vi "Microscope.vi"() -> ()   [LabVIEW 2012]
uses:
  typedefs/Graph.ctl
  typedefs/HWsettings.ctl
  typedefs/Stage Parameters.ctl
  typedefs/ScanMode.ctl
  typedefs/Scan Parameters.ctl
  typedefs/PMTs.ctl
  classes/Microscope.lvclass
  classes/MCCPMT.lvclass
  typedefs/StageEvent.ctl
  typedefs/MicroscopeEvent.ctl
  variables/GlobalUI.vi
  sequences/full_restart_acquire_sequence.vi
panel:
  out "must be an integer":dbl=82.0
  in  "Tab Control":enum32{"Run", "Settings"}(tab)
  in  "Close":bool
  in  "Rot":bool
  in  "SpecWiz":bool
  in  "MG17Motor":refnum<k7>(container)
  in  "dV":dbl=0.5 min=0.0 step=0.25
  in  "Stokes":bool=TRUE
  in  "Pump":bool=TRUE
  out "XY Graph":T1={[0.0, 0.20101165771484375, 0.4090237617492676, 0.6170353889465332, 0.825047492980957, 1.0170583724975586, 1.2410712242126465, 1.432082176208496, 1.6400938034057617, 1.8321051597595215, 2.0721187591552734], [0.8903510861280485, 0.8953041634908552, 0.8929806592987812, 0.8912776295731716, 0.8909548875762202, 0.8924578410823198, 0.8944300209603651, 0.8951743521341458, 0.8952005525914619, 0.8928044016768294]}
  out "XY Graph 2":T1={[0.0, 0.20101165771484375, 0.4090237617492676, 0.6170353889465332, 0.825047492980957, 1.0170583724975586, 1.2410712242126465, 1.432082176208496, 1.6400938034057617, 1.8321051597595215, 2.0721187591552734], [0.0045469702743902015, 0.004504096798780445, 0.0043075933689024, 0.00459937118902435, 0.004633908155487764, 0.004538633765243861, 0.004433831935975568, 0.004408822408536544, 0.004301638719512153, 0.00419088224085362]}
  out "XY Graph 3":T1={[0.0, 0.20101165771484375, 0.4090237617492676, 0.6170353889465332, 0.825047492980957, 1.0170583724975586, 1.2410712242126465, 1.432082176208496, 1.6400938034057617, 1.8321051597595215, 2.0721187591552734], [3.0555949885670746, 3.0528808593750005, 3.052250857469512, 3.0531321455792657, 3.0502929687499982, 3.0587985899390246, 3.0497058403201254, 3.0519769435975626, 3.0576517244664645, 3.065386814024396]}
  out "intensity1":dbl=0.8928044016768294 format="%#.4f"
  out "intensity2":dbl=0.00419088224085362 format="%#.4f"
  out "intensity3":dbl=3.065386814024396 format="%#.4f"
  in  "Use Image Controls Min Max values for tiff":bool=TRUE
  in  "preset3":bool
  in  "zero3":bool
  out "PMT3":bool
  in  "PMT3":dbl(slide)=0.7 min=0.0 max=1.0 step=0.01 scale=0.0..1.0
  in  "Hi-Res Mode":bool
  in  "autoscale1":bool
  in  "Sample Description":string="AXN static 25d"
  in  "Stokes Power (mW)":string="200"
  in  "Pump Power (mW)":string="5"
  in  "max1":dbl=250.0 caption="max" step=250.0 format="%#.0f"
  in  "min1":dbl format="%#.0f"
  in  "NormalMode":bool
  in  "SpeedMode":bool
  in  "Target position mm":dbl=82.1047 step=0.025 format="%_6g"
  out "PMT2":bool
  out "PMT1":bool
  in  "MoveStageTarget":bool
  in  "grayscale":bool
  in  "jet":bool
  in  "preset2":bool
  in  "preset1":bool
  in  "PMT2":dbl(slide)=0.7 min=0.0 max=1.0 step=0.01 scale=0.0..1.0
  in  "PMT1":dbl(slide)=0.6 min=0.0 max=1.0 step=0.01 scale=0.0..1.0 scale format="%#_1g"
  in  "Save This":bool
  in  "Acquire":bool
  in  "Zoom":dbl=4.0
  out "CH1":dbl[][](graph)=[[93.19026295731707, 104.20636432926828, 92.89253048780488, 100.93130716463415, 83.36509146341463, 82.17416158536585, 89.31974085365853, 99.74037728658537, 93.78572789634147, 90.21293826219512, 85.44921875, 94.08346036585365, 87.23561356707317, 91.4038681402439, 89.02200838414635, 93.78572789634147, 83.66282393292683, 84.8537538109756, 85.44921875, 91.9993330792683, 73.5399199695122, 100.33584222560977, 86.93788109756098, 92.2970655487805, 94.38119283536585, 89.31974085365853, 90.21293826219512, 86.93788109756098, 86.0446836890244, 85.1514862804878, 100.03810975609757, 92.2970655487805, 91.9993330792683, 91.4038681402439, 90.21293826219512, 97.3585175304878, 86.93788109756098, 83.36509146341463, 89.02200838414635, 89.31974085365853, 88.72427591463415, 90.8084032012195, 95.57212271341463, 84.8537538109756, 90.21293826219512, 75.32631478658537, 84.25828887195121, 81.28096417682927, 105.39729420731707, 90.8084032012195], [98.2517149390244, 83.96055640243902, 93.78572789634147, 100.33584222560977, 95.86985518292683, 90.8084032012195, 89.91520579268293, 89.61747332317073, 88.42654344512195, 96.16758765243902, 95.57212271341463, 99.14491234756098, 89.31974085365853, 94.38119283536585, 99.14491234756098, 93.78572789634147, 88.42654344512195, 87.23561356707317, 81.87642911585365, 79.4945693597561, 86.64014862804879, 80.38776676829268, 90.21293826219512, 92.59479801829268, 90.21293826219512, 88.42654344512195, 88.72427591463415, 91.7016006097561, 88.12881097560977, 89.02200838414635, 86.93788109756098, 101.82450457317074, 97.0607850609756, 94.97665777439023, 85.1514862804878, 100.33584222560977, 89.61747332317073, 96.16758765243902, 92.2970655487805, 91.1061356707317, 98.54944740853658, 89.02200838414635, 86.64014862804879, 87.83107850609755, 88.12881097560977, 91.4038681402439, 89.91520579268293, 91.9993330792683, 86.64014862804879, 91.9993330792683], [97.0607850609756, 90.51067073170732, 89.31974085365853, 99.14491234756098, 90.8084032012195, 77.41044207317073, 88.72427591463415, 89.91520579268293, 84.25828887195121, 98.2517149390244, 80.38776676829268, 93.78572789634147, 90.51067073170732, 100.63357469512195, 94.67892530487805, 96.16758765243902, 92.59479801829268, 82.76962652439023, 89.02200838414635, 90.51067073170732, 84.55602134146342, 87.23561356707317, 92.2970655487805, 88.12881097560977, 83.06735899390245, 89.02200838414635, 85.1514862804878, 83.66282393292683, 86.93788109756098, 87.53334603658537, 94.38119283536585, 96.76305259146342, 80.38776676829268, 100.03810975609757, 96.46532012195121, 84.25828887195121, 85.44921875, 103.6108993902439, 92.59479801829268, 87.53334603658537, 89.02200838414635, 86.0446836890244, 98.2517149390244, 88.12881097560977, 95.86985518292683, 91.7016006097561, 87.53334603658537, 84.25828887195121, 80.68549923780488, 89.61747332317073], [90.21293826219512, 88.42654344512195, 96.46532012195121, 93.78572789634147, 90.21293826219512, 88.42654344512195, 91.9993330792683, 85.44921875, 87.53334603658537, 77.11270960365853, 90.21293826219512, 94.67892530487805, 83.96055640243902, 90.8084032012195, 86.0446836890244, 86.34241615853658, 89.91520579268293, 87.83107850609755, 102.12223704268293, 91.9993330792683, 89.31974085365853, 98.54944740853658, 104.20636432926828, 80.98323170731707, 85.44921875, 83.96055640243902, 88.42654344512195, 86.64014862804879, 87.53334603658537, 91.7016006097561, 88.72427591463415, 91.7016006097561, 84.25828887195121, 88.42654344512195, 85.1514862804878, 82.47189405487805, 88.72427591463415, 102.71770198170731, 98.54944740853658, 81.28096417682927, 98.54944740853658, 82.17416158536585, 91.9993330792683, 83.36509146341463, 97.3585175304878, 86.93788109756098, 102.71770198170731, 97.9539824695122, 89.61747332317073, 91.4038681402439], [87.23561356707317, 93.48799542682927, 87.23561356707317, 85.44921875, 93.48799542682927, 89.31974085365853, 89.61747332317073, 92.89253048780488, 95.86985518292683, 86.64014862804879, 79.1968368902439, 85.7469512195122, 82.47189405487805, 89.61747332317073, 78.8991044207317, 86.34241615853658, 84.25828887195121, 83.06735899390245, 92.59479801829268, 88.12881097560977, 92.89253048780488, 78.30363948170732, 94.08346036585365, 82.17416158536585, 87.23561356707317, 94.08346036585365, 80.0900342987805, 92.59479801829268, 87.83107850609755, 87.53334603658537, 77.70817454268293, 76.51724466463415, 86.64014862804879, 81.87642911585365, 86.0446836890244, 80.98323170731707, 96.46532012195121, 88.12881097560977, 97.9539824695122, 86.64014862804879, 93.19026295731707, 91.9993330792683, 86.64014862804879, 87.53334603658537, 91.4038681402439, 85.7469512195122, 88.72427591463415, 85.7469512195122, 86.34241615853658, 81.57869664634147], [105.39729420731707, 88.12881097560977, 89.31974085365853, 88.12881097560977, 98.54944740853658, 76.81497713414635, 96.46532012195121, 94.38119283536585, 84.55602134146342, 76.21951219512195, 97.9539824695122, 80.0900342987805, 89.91520579268293, 87.83107850609755, 84.55602134146342, 86.64014862804879, 87.83107850609755, 95.86985518292683, 93.78572789634147, 84.25828887195121, 98.54944740853658, 87.83107850609755, 87.83107850609755, 89.61747332317073, 84.25828887195121, 94.08346036585365, 83.06735899390245, 98.84717987804879, 83.66282393292683, 77.11270960365853, 91.1061356707317, 90.51067073170732, 83.96055640243902, 86.64014862804879, 90.8084032012195, 85.7469512195122, 76.21951219512195, 84.25828887195121, 87.53334603658537, 86.0446836890244, 89.91520579268293, 88.72427591463415, 83.66282393292683, 88.42654344512195, 94.38119283536585, 90.51067073170732, 95.27439024390245, 84.25828887195121, 87.23561356707317, 84.8537538109756], [91.9993330792683, 88.72427591463415, 79.7923018292683, 75.32631478658537, 90.21293826219512, 86.93788109756098, 90.51067073170732, 94.08346036585365, 94.08346036585365, 94.38119283536585, 91.1061356707317, 99.74037728658537, 85.44921875, 92.2970655487805, 87.83107850609755, 86.93788109756098, 86.93788109756098, 93.19026295731707, 83.66282393292683, 93.48799542682927, 86.0446836890244, 101.82450457317074, 87.83107850609755, 97.9539824695122, 87.23561356707317, 90.8084032012195, 87.23561356707317, 90.8084032012195, 84.8537538109756, 79.4945693597561, 81.28096417682927, 87.23561356707317, 86.34241615853658, 94.08346036585365, 88.12881097560977, 85.7469512195122, 85.7469512195122, 89.91520579268293, 89.61747332317073, 88.42654344512195, 87.53334603658537, 97.65625, 87.23561356707317, 92.59479801829268, 97.65625, 96.16758765243902, 91.4038681402439, 95.86985518292683, 89.61747332317073, 83.66282393292683], [88.42654344512195, 89.02200838414635, 95.57212271341463, 85.44921875, 91.7016006097561, 87.53334603658537, 81.87642911585365, 79.7923018292683, 96.46532012195121, 80.38776676829268, 92.89253048780488, 94.08346036585365, 95.86985518292683, 78.8991044207317, 93.48799542682927, 87.23561356707317, 89.61747332317073, 73.8376524390244, 77.11270960365853, 83.36509146341463, 83.36509146341463, 100.33584222560977, 87.23561356707317, 86.34241615853658, 104.50409679878048, 83.36509146341463, 91.9993330792683, 85.7469512195122, 100.03810975609757, 86.0446836890244, 89.61747332317073, 91.4038681402439, 97.0607850609756, 92.2970655487805, 88.12881097560977, 89.02200838414635, 90.8084032012195, 90.8084032012195, 83.66282393292683, 91.7016006097561, 81.28096417682927, 82.76962652439023, 94.08346036585365, 82.47189405487805, 91.1061356707317, 83.06735899390245, 93.78572789634147, 82.76962652439023, 89.61747332317073, 89.61747332317073], [89.02200838414635, 83.36509146341463, 93.78572789634147, 99.44264481707317, 91.7016006097561, 86.93788109756098, 87.23561356707317, 90.8084032012195, 90.21293826219512, 87.23561356707317, 90.51067073170732, 94.97665777439023, 87.83107850609755, 88.72427591463415, 88.12881097560977, 84.55602134146342, 84.55602134146342, 109.86328125, 75.32631478658537, 85.7469512195122, 80.38776676829268, 82.47189405487805, 93.78572789634147, 80.0900342987805, 91.4038681402439, 85.7469512195122, 87.83107850609755, 79.7923018292683, 95.57212271341463, 90.8084032012195, 89.91520579268293, 84.55602134146342, 88.42654344512195, 91.1061356707317, 87.53334603658537, 95.57212271341463, 95.27439024390245, 69.37166539634147, 94.08346036585365, 90.8084032012195, 82.47189405487805, 86.0446836890244, 98.84717987804879, 90.51067073170732, 97.65625, 84.25828887195121, 100.03810975609757, 79.4945693597561, 89.91520579268293, 94.67892530487805], [96.76305259146342, 84.8537538109756, 96.76305259146342, 85.1514862804878, 90.51067073170732, 88.12881097560977, 89.31974085365853, 84.8537538109756, 96.16758765243902, 78.00590701219512, 82.47189405487805, 92.59479801829268, 87.83107850609755, 84.25828887195121, 94.67892530487805, 86.64014862804879, 92.2970655487805, 78.00590701219512, 86.0446836890244, 91.9993330792683, 84.8537538109756, 86.64014862804879, 90.51067073170732, 81.28096417682927, 75.92177972560977, 86.64014862804879, 79.7923018292683, 71.75352515243902, 89.91520579268293, 83.36509146341463, 88.12881097560977, 82.17416158536585, 95.86985518292683, 90.21293826219512, 88.12881097560977, 88.42654344512195, 94.67892530487805, 91.9993330792683, 90.8084032012195, 84.8537538109756, 88.12881097560977, 93.19026295731707, 95.27439024390245, 94.08346036585365, 81.87642911585365, 94.67892530487805, 94.67892530487805, 96.76305259146342, 83.96055640243902, 82.47189405487805], [86.34241615853658, 91.7016006097561, 96.46532012195121, 88.12881097560977, 89.91520579268293, 103.9086318597561, 98.54944740853658, 96.76305259146342, 92.89253048780488, 98.84717987804879, 81.28096417682927, 94.38119283536585, 89.91520579268293, 90.21293826219512, 92.59479801829268, 88.72427591463415, 92.2970655487805, 90.21293826219512, 86.34241615853658, 91.9993330792683, 78.00590701219512, 84.55602134146342, 81.57869664634147, 97.3585175304878, 83.66282393292683, 88.72427591463415, 100.03810975609757, 83.66282393292683, 91.9993330792683, 104.80182926829269, 89.61747332317073, 90.21293826219512, 92.59479801829268, 88.72427591463415, 96.16758765243902, 89.02200838414635, 88.72427591463415, 88.72427591463415, 91.7016006097561, 87.83107850609755, 89.31974085365853, 87.53334603658537, 104.20636432926828, 86.34241615853658, 85.1514862804878, 96.16758765243902, 88.42654344512195, 78.8991044207317, 92.59479801829268, 94.97665777439023], [91.9993330792683, 86.0446836890244, 98.84717987804879, 89.61747332317073, 85.1514862804878, 85.1514862804878, 94.08346036585365, 88.12881097560977, 100.93130716463415, 84.55602134146342, 89.91520579268293, 86.64014862804879, 83.66282393292683, 93.48799542682927, 99.14491234756098, 86.93788109756098, 93.78572789634147, 95.86985518292683, 86.34241615853658, 104.20636432926828, 104.20636432926828, 93.48799542682927, 94.08346036585365, 86.34241615853658, 102.41996951219512, 93.78572789634147, 94.38119283536585, 79.4945693597561, 86.64014862804879, 88.42654344512195, 89.61747332317073, 86.0446836890244, 80.98323170731707, 86.64014862804879, 84.8537538109756, 90.21293826219512, 88.42654344512195, 91.9993330792683, 87.53334603658537, 98.2517149390244, 93.78572789634147, 87.23561356707317, 93.48799542682927, 81.57869664634147, 91.4038681402439, 98.2517149390244, 86.93788109756098, 92.89253048780488, 84.8537538109756, 99.44264481707317], [87.83107850609755, 91.1061356707317, 91.1061356707317, 90.8084032012195, 90.8084032012195, 76.81497713414635, 79.7923018292683, 95.57212271341463, 89.91520579268293, 93.78572789634147, 94.08346036585365, 93.78572789634147, 89.91520579268293, 88.12881097560977, 96.46532012195121, 95.86985518292683, 93.78572789634147, 88.72427591463415, 83.96055640243902, 89.91520579268293, 88.72427591463415, 86.34241615853658, 88.12881097560977, 87.83107850609755, 98.2517149390244, 90.21293826219512, 95.57212271341463, 89.31974085365853, 89.91520579268293, 82.76962652439023, 88.42654344512195, 86.34241615853658, 93.19026295731707, 95.57212271341463, 85.1514862804878, 89.91520579268293, 87.53334603658537, 101.82450457317074, 93.48799542682927, 86.0446836890244, 89.91520579268293, 85.1514862804878, 82.17416158536585, 93.78572789634147, 90.8084032012195, 94.08346036585365, 87.23561356707317, 100.33584222560977, 89.61747332317073, 80.98323170731707], [94.08346036585365, 94.08346036585365, 92.59479801829268, 91.9993330792683, 86.34241615853658, 87.83107850609755, 86.0446836890244, 79.7923018292683, 94.97665777439023, 88.72427591463415, 95.57212271341463, 81.57869664634147, 83.96055640243902, 93.48799542682927, 87.23561356707317, 94.08346036585365, 85.7469512195122, 88.72427591463415, 94.67892530487805, 100.63357469512195, 84.55602134146342, 95.27439024390245, 88.42654344512195, 102.41996951219512, 91.1061356707317, 93.78572789634147, 98.54944740853658, 100.03810975609757, 94.08346036585365, 90.8084032012195, 91.9993330792683, 92.2970655487805, 96.16758765243902, 89.61747332317073, 92.89253048780488, 91.7016006097561, 87.53334603658537, 91.1061356707317, 86.64014862804879, 79.4945693597561, 82.17416158536585, 93.48799542682927, 94.38119283536585, 91.7016006097561, 85.1514862804878, 92.89253048780488, 86.93788109756098, 99.44264481707317, 92.59479801829268, 87.53334603658537], [91.9993330792683, 87.53334603658537, 87.23561356707317, 91.1061356707317, 78.00590701219512, 83.96055640243902, 78.30363948170732, 99.14491234756098, 94.97665777439023, 86.93788109756098, 94.97665777439023, 91.7016006097561, 84.25828887195121, 90.8084032012195, 82.17416158536585, 98.54944740853658, 88.72427591463415, 91.1061356707317, 81.57869664634147, 85.44921875, 88.72427591463415, 83.06735899390245, 91.4038681402439, 98.2517149390244, 83.96055640243902, 89.31974085365853, 80.0900342987805, 106.88595655487805, 88.72427591463415, 81.87642911585365, 89.02200838414635, 92.2970655487805, 86.93788109756098, 89.61747332317073, 94.08346036585365, 81.87642911585365, 85.7469512195122, 91.4038681402439, 83.06735899390245, 86.64014862804879, 87.83107850609755, 86.0446836890244, 83.66282393292683, 94.67892530487805, 98.2517149390244, 86.93788109756098, 98.84717987804879, 80.38776676829268, 103.9086318597561, 94.38119283536585], [86.64014862804879, 82.76962652439023, 81.57869664634147, 96.16758765243902, 89.91520579268293, 78.8991044207317, 101.22903963414633, 88.42654344512195, 70.26486280487805, 81.28096417682927, 81.28096417682927, 92.89253048780488, 88.12881097560977, 88.72427591463415, 95.27439024390245, 87.83107850609755, 85.44921875, 93.78572789634147, 79.7923018292683, 83.36509146341463, 93.48799542682927, 95.86985518292683, 88.12881097560977, 87.23561356707317, 96.16758765243902, 83.06735899390245, 78.00590701219512, 86.0446836890244, 93.48799542682927, 78.30363948170732, 93.19026295731707, 99.44264481707317, 90.21293826219512, 90.51067073170732, 94.67892530487805, 80.68549923780488, 91.1061356707317, 92.89253048780488, 90.8084032012195, 88.42654344512195, 92.59479801829268, 94.67892530487805, 89.31974085365853, 73.2421875, 94.38119283536585, 94.38119283536585, 89.31974085365853, 93.19026295731707, 89.02200838414635, 88.12881097560977], [92.2970655487805, 92.59479801829268, 97.0607850609756, 98.2517149390244, 82.17416158536585, 95.57212271341463, 78.00590701219512, 88.12881097560977, 95.86985518292683, 89.02200838414635, 91.7016006097561, 83.06735899390245, 80.98323170731707, 90.51067073170732, 82.76962652439023, 99.44264481707317, 85.7469512195122, 89.31974085365853, 86.34241615853658, 97.9539824695122, 88.12881097560977, 91.9993330792683, 72.34899009146342, 95.27439024390245, 94.97665777439023, 91.4038681402439, 87.53334603658537, 81.57869664634147, 83.96055640243902, 91.4038681402439, 94.97665777439023, 83.66282393292683, 95.57212271341463, 84.8537538109756, 94.38119283536585, 91.9993330792683, 92.89253048780488, 81.87642911585365, 103.01543445121952, 95.27439024390245, 94.97665777439023, 85.7469512195122, 91.4038681402439, 94.08346036585365, 94.67892530487805, 81.57869664634147, 95.86985518292683, 96.76305259146342, 89.31974085365853, 87.23561356707317], [85.44921875, 87.83107850609755, 96.76305259146342, 97.0607850609756, 91.9993330792683, 99.14491234756098, 81.57869664634147, 84.55602134146342, 94.38119283536585, 88.72427591463415, 81.87642911585365, 80.0900342987805, 85.1514862804878, 93.19026295731707, 84.55602134146342, 95.86985518292683, 96.76305259146342, 85.7469512195122, 93.19026295731707, 89.31974085365853, 88.42654344512195, 94.97665777439023, 104.80182926829269, 86.34241615853658, 88.72427591463415, 88.72427591463415, 97.65625, 94.67892530487805, 86.93788109756098, 76.51724466463415, 85.7469512195122, 88.42654344512195, 91.9993330792683, 83.06735899390245, 79.4945693597561, 82.76962652439023, 88.72427591463415, 89.61747332317073, 109.86328125, 82.76962652439023, 97.0607850609756, 85.7469512195122, 83.66282393292683, 98.2517149390244, 93.19026295731707, 91.4038681402439, 90.51067073170732, 86.0446836890244, 86.93788109756098, 87.23561356707317], [97.0607850609756, 86.93788109756098, 75.62404725609755, 85.7469512195122, 89.91520579268293, 90.21293826219512, 80.38776676829268, 82.17416158536585, 75.92177972560977, 99.44264481707317, 88.72427591463415, 85.7469512195122, 94.67892530487805, 79.7923018292683, 86.93788109756098, 100.63357469512195, 92.89253048780488, 75.92177972560977, 89.02200838414635, 87.23561356707317, 95.86985518292683, 96.76305259146342, 75.62404725609755, 85.44921875, 83.36509146341463, 100.63357469512195, 96.46532012195121, 87.83107850609755, 93.19026295731707, 91.1061356707317, 88.12881097560977, 97.65625, 86.64014862804879, 94.67892530487805, 81.87642911585365, 89.91520579268293, 99.74037728658537, 96.46532012195121, 81.28096417682927, 87.23561356707317, 90.21293826219512, 92.2970655487805, 101.22903963414633, 97.9539824695122, 88.12881097560977, 88.12881097560977, 97.0607850609756, 86.34241615853658, 88.42654344512195, 101.52677210365854], [86.64014862804879, 92.2970655487805, 89.31974085365853, 84.55602134146342, 83.96055640243902, 95.86985518292683, 86.93788109756098, 86.34241615853658, 87.53334603658537, 83.06735899390245, 86.0446836890244, 97.0607850609756, 89.91520579268293, 94.97665777439023, 88.42654344512195, 99.44264481707317, 92.2970655487805, 88.12881097560977, 88.12881097560977, 84.8537538109756, 90.8084032012195, 85.7469512195122, 90.21293826219512, 95.57212271341463, 90.8084032012195, 90.51067073170732, 84.25828887195121, 87.53334603658537, 92.2970655487805, 79.7923018292683, 82.17416158536585, 91.7016006097561, 97.0607850609756, 88.72427591463415, 87.83107850609755, 87.23561356707317, 87.23561356707317, 80.68549923780488, 88.42654344512195, 93.19026295731707, 91.4038681402439, 78.6013719512195, 92.89253048780488, 93.19026295731707, 95.57212271341463, 82.17416158536585, 98.2517149390244, 89.91520579268293, 102.71770198170731, 89.31974085365853], [89.02200838414635, 89.02200838414635, 98.84717987804879, 86.0446836890244, 80.38776676829268, 89.02200838414635, 91.1061356707317, 94.67892530487805, 78.6013719512195, 87.53334603658537, 89.91520579268293, 89.31974085365853, 88.72427591463415, 93.48799542682927, 83.96055640243902, 92.59479801829268, 86.64014862804879, 86.64014862804879, 91.4038681402439, 95.86985518292683, 89.61747332317073, 87.53334603658537, 88.12881097560977, 85.7469512195122, 93.78572789634147, 94.67892530487805, 90.21293826219512, 91.1061356707317, 85.1514862804878, 89.02200838414635, 88.12881097560977, 84.8537538109756, 81.28096417682927, 92.59479801829268, 83.06735899390245, 85.1514862804878, 85.1514862804878, 90.51067073170732, 89.02200838414635, 81.87642911585365, 93.19026295731707, 93.19026295731707, 89.61747332317073, 81.87642911585365, 89.91520579268293, 91.1061356707317, 108.67235137195121, 89.31974085365853, 84.25828887195121, 79.4945693597561], [98.2517149390244, 95.57212271341463, 81.57869664634147, 87.53334603658537, 105.39729420731707, 97.0607850609756, 91.7016006097561, 91.4038681402439, 97.0607850609756, 90.8084032012195, 90.8084032012195, 86.64014862804879, 90.21293826219512, 90.8084032012195, 85.7469512195122, 84.25828887195121, 78.00590701219512, 82.76962652439023, 92.59479801829268, 95.57212271341463, 85.1514862804878, 86.64014862804879, 83.96055640243902, 89.02200838414635, 88.72427591463415, 91.9993330792683, 91.7016006097561, 95.57212271341463, 88.72427591463415, 94.97665777439023, 89.02200838414635, 94.08346036585365, 93.48799542682927, 98.84717987804879, 83.96055640243902, 81.28096417682927, 87.83107850609755, 84.25828887195121, 89.91520579268293, 88.12881097560977, 93.78572789634147, 89.91520579268293, 82.76962652439023, 82.76962652439023, 95.86985518292683, 79.7923018292683, 91.4038681402439, 81.57869664634147, 81.57869664634147, 83.06735899390245], [89.91520579268293, 86.34241615853658, 95.86985518292683, 82.76962652439023, 78.00590701219512, 89.31974085365853, 84.55602134146342, 97.3585175304878, 91.1061356707317, 88.72427591463415, 90.51067073170732, 94.08346036585365, 89.61747332317073, 82.47189405487805, 89.91520579268293, 83.66282393292683, 78.8991044207317, 88.72427591463415, 86.64014862804879, 91.4038681402439, 93.48799542682927, 86.0446836890244, 89.31974085365853, 102.12223704268293, 83.36509146341463, 90.51067073170732, 93.78572789634147, 96.16758765243902, 83.66282393292683, 81.87642911585365, 83.66282393292683, 83.36509146341463, 83.66282393292683, 94.38119283536585, 96.76305259146342, 85.7469512195122, 97.0607850609756, 87.53334603658537, 90.8084032012195, 87.53334603658537, 97.65625, 80.98323170731707, 89.61747332317073, 77.70817454268293, 81.87642911585365, 80.38776676829268, 87.83107850609755, 93.78572789634147, 90.8084032012195, 87.83107850609755], [82.17416158536585, 87.83107850609755, 87.23561356707317, 81.87642911585365, 83.96055640243902, 86.93788109756098, 98.54944740853658, 94.67892530487805, 83.36509146341463, 92.2970655487805, 90.8084032012195, 92.59479801829268, 90.21293826219512, 83.36509146341463, 85.44921875, 91.9993330792683, 81.57869664634147, 83.96055640243902, 94.67892530487805, 78.6013719512195, 97.0607850609756, 89.61747332317073, 85.44921875, 93.19026295731707, 88.12881097560977, 90.21293826219512, 86.93788109756098, 83.96055640243902, 91.9993330792683, 88.12881097560977, 92.59479801829268, 92.2970655487805, 93.48799542682927, 87.53334603658537, 84.25828887195121, 86.64014862804879, 81.28096417682927, 90.21293826219512, 91.7016006097561, 95.57212271341463, 88.12881097560977, 90.51067073170732, 72.9444550304878, 92.2970655487805, 82.17416158536585, 92.2970655487805, 76.21951219512195, 82.47189405487805, 88.72427591463415, 94.38119283536585], [95.57212271341463, 86.93788109756098, 84.8537538109756, 83.06735899390245, 82.17416158536585, 88.12881097560977, 94.08346036585365, 83.06735899390245, 87.53334603658537, 88.42654344512195, 83.36509146341463, 99.14491234756098, 80.38776676829268, 92.89253048780488, 89.02200838414635, 86.64014862804879, 86.93788109756098, 93.48799542682927, 87.23561356707317, 73.2421875, 81.28096417682927, 89.61747332317073, 91.9993330792683, 79.1968368902439, 85.7469512195122, 85.1514862804878, 83.36509146341463, 89.02200838414635, 91.4038681402439, 85.1514862804878, 92.59479801829268, 94.38119283536585, 94.38119283536585, 84.25828887195121, 81.28096417682927, 82.76962652439023, 79.1968368902439, 97.3585175304878, 96.46532012195121, 85.1514862804878, 97.3585175304878, 89.91520579268293, 99.44264481707317, 93.78572789634147, 93.78572789634147, 102.12223704268293, 92.59479801829268, 77.11270960365853, 83.96055640243902, 91.4038681402439], [93.19026295731707, 86.0446836890244, 83.96055640243902, 76.81497713414635, 90.51067073170732, 88.72427591463415, 88.42654344512195, 86.93788109756098, 87.23561356707317, 91.7016006097561, 98.84717987804879, 105.69502667682926, 96.46532012195121, 84.55602134146342, 99.74037728658537, 86.0446836890244, 82.47189405487805, 95.57212271341463, 90.8084032012195, 90.51067073170732, 80.0900342987805, 78.30363948170732, 88.72427591463415, 86.93788109756098, 97.3585175304878, 88.72427591463415, 91.9993330792683, 90.51067073170732, 83.36509146341463, 86.93788109756098, 91.7016006097561, 88.12881097560977, 103.31316692073172, 87.83107850609755, 95.86985518292683, 85.7469512195122, 98.84717987804879, 92.59479801829268, 93.48799542682927, 94.08346036585365, 94.97665777439023, 87.53334603658537, 84.55602134146342, 86.93788109756098, 97.3585175304878, 80.98323170731707, 82.76962652439023, 89.91520579268293, 87.83107850609755, 88.12881097560977], [103.9086318597561, 90.8084032012195, 88.72427591463415, 79.4945693597561, 83.66282393292683, 84.55602134146342, 80.38776676829268, 91.1061356707317, 93.48799542682927, 92.59479801829268, 96.76305259146342, 91.1061356707317, 94.67892530487805, 94.67892530487805, 89.02200838414635, 90.8084032012195, 88.42654344512195, 90.51067073170732, 89.61747332317073, 93.48799542682927, 85.7469512195122, 86.64014862804879, 84.8537538109756, 101.52677210365854, 92.2970655487805, 94.67892530487805, 89.91520579268293, 93.48799542682927, 87.53334603658537, 78.30363948170732, 89.31974085365853, 86.93788109756098, 78.30363948170732, 91.7016006097561, 84.8537538109756, 86.93788109756098, 100.33584222560977, 79.1968368902439, 87.83107850609755, 87.53334603658537, 89.02200838414635, 90.8084032012195, 101.52677210365854, 87.23561356707317, 87.53334603658537, 87.53334603658537, 101.22903963414633, 73.8376524390244, 87.53334603658537, 86.64014862804879], [93.19026295731707, 84.25828887195121, 69.37166539634147, 90.51067073170732, 84.25828887195121, 85.7469512195122, 91.7016006097561, 87.53334603658537, 91.1061356707317, 90.51067073170732, 77.70817454268293, 86.64014862804879, 89.61747332317073, 81.87642911585365, 78.6013719512195, 92.89253048780488, 84.25828887195121, 96.46532012195121, 89.91520579268293, 97.9539824695122, 99.44264481707317, 95.57212271341463, 84.8537538109756, 85.7469512195122, 83.66282393292683, 86.64014862804879, 80.0900342987805, 83.66282393292683, 84.25828887195121, 89.02200838414635, 86.93788109756098, 91.9993330792683, 88.12881097560977, 101.82450457317074, 101.82450457317074, 90.8084032012195, 84.8537538109756, 82.17416158536585, 83.36509146341463, 96.46532012195121, 109.86328125, 86.64014862804879, 84.8537538109756, 85.44921875, 77.41044207317073, 88.42654344512195, 87.83107850609755, 83.36509146341463, 84.8537538109756, 96.16758765243902], [98.54944740853658, 97.9539824695122, 96.46532012195121, 93.19026295731707, 89.31974085365853, 97.0607850609756, 95.57212271341463, 96.16758765243902, 80.38776676829268, 92.2970655487805, 92.59479801829268, 92.2970655487805, 89.02200838414635, 82.47189405487805, 89.31974085365853, 86.34241615853658, 77.41044207317073, 97.0607850609756, 86.64014862804879, 89.31974085365853, 84.55602134146342, 86.64014862804879, 82.47189405487805, 98.84717987804879, 83.66282393292683, 96.46532012195121, 89.61747332317073, 87.53334603658537, 98.84717987804879, 80.98323170731707, 94.08346036585365, 83.06735899390245, 88.12881097560977, 96.76305259146342, 91.1061356707317, 93.48799542682927, 89.02200838414635, 89.61747332317073, 91.4038681402439, 86.93788109756098, 86.34241615853658, 89.91520579268293, 91.4038681402439, 93.48799542682927, 80.68549923780488, 98.2517149390244, 91.1061356707317, 94.67892530487805, 95.57212271341463, 96.16758765243902], [80.68549923780488, 95.27439024390245, 80.68549923780488, 84.8537538109756, 86.0446836890244, 78.00590701219512, 78.8991044207317, 92.2970655487805, 84.8537538109756, 90.8084032012195, 78.8991044207317, 82.47189405487805, 87.23561356707317, 96.16758765243902, 89.31974085365853, 93.48799542682927, 83.66282393292683, 99.14491234756098, 90.51067073170732, 73.5399199695122, 91.4038681402439, 88.72427591463415, 87.53334603658537, 80.0900342987805, 96.16758765243902, 87.53334603658537, 86.64014862804879, 78.00590701219512, 88.12881097560977, 88.42654344512195, 81.87642911585365, 86.34241615853658, 97.3585175304878, 80.38776676829268, 100.03810975609757, 92.89253048780488, 92.59479801829268, 84.25828887195121, 87.83107850609755, 83.96055640243902, 74.73084984756098, 86.0446836890244, 99.14491234756098, 94.67892530487805, 79.1968368902439, 82.47189405487805, 84.25828887195121, 79.1968368902439, 89.31974085365853, 84.55602134146342], [84.55602134146342, 96.76305259146342, 79.1968368902439, 97.0607850609756, 94.97665777439023, 88.72427591463415, 93.78572789634147, 94.67892530487805, 89.61747332317073, 84.8537538109756, 89.02200838414635, 89.61747332317073, 89.02200838414635, 88.12881097560977, 90.8084032012195, 98.84717987804879, 80.0900342987805, 101.82450457317074, 94.97665777439023, 93.78572789634147, 84.25828887195121, 86.93788109756098, 89.31974085365853, 93.19026295731707, 97.65625, 91.1061356707317, 90.8084032012195, 92.89253048780488, 83.36509146341463, 89.31974085365853, 74.73084984756098, 90.21293826219512, 89.02200838414635, 85.1514862804878, 88.12881097560977, 92.59479801829268, 94.08346036585365, 94.08346036585365, 90.51067073170732, 90.8084032012195, 88.42654344512195, 93.48799542682927, 90.21293826219512, 85.7469512195122, 90.21293826219512, 85.7469512195122, 95.27439024390245, 95.86985518292683, 90.21293826219512, 92.89253048780488], [83.66282393292683, 88.42654344512195, 72.6467225609756, 86.0446836890244, 79.4945693597561, 91.1061356707317, 92.59479801829268, 89.61747332317073, 82.76962652439023, 101.22903963414633, 83.66282393292683, 80.98323170731707, 84.25828887195121, 83.36509146341463, 89.31974085365853, 87.53334603658537, 83.36509146341463, 83.66282393292683, 102.12223704268293, 89.31974085365853, 85.44921875, 90.51067073170732, 85.1514862804878, 90.21293826219512, 85.1514862804878, 92.2970655487805, 93.78572789634147, 93.48799542682927, 80.98323170731707, 91.1061356707317, 87.53334603658537, 81.57869664634147, 92.59479801829268, 102.12223704268293, 87.83107850609755, 96.16758765243902, 91.4038681402439, 87.53334603658537, 91.1061356707317, 88.12881097560977, 91.9993330792683, 86.34241615853658, 86.93788109756098, 84.8537538109756, 84.25828887195121, 97.3585175304878, 86.34241615853658, 84.55602134146342, 80.0900342987805, 82.76962652439023], [91.4038681402439, 88.42654344512195, 96.46532012195121, 90.51067073170732, 86.34241615853658, 87.23561356707317, 88.72427591463415, 87.83107850609755, 89.31974085365853, 101.52677210365854, 83.36509146341463, 75.32631478658537, 94.08346036585365, 94.97665777439023, 95.86985518292683, 90.21293826219512, 85.1514862804878, 94.97665777439023, 88.12881097560977, 90.21293826219512, 91.4038681402439, 96.16758765243902, 89.02200838414635, 94.97665777439023, 93.19026295731707, 86.34241615853658, 96.16758765243902, 91.1061356707317, 98.2517149390244, 81.28096417682927, 90.51067073170732, 82.47189405487805, 93.19026295731707, 88.72427591463415, 83.96055640243902, 85.7469512195122, 89.02200838414635, 89.61747332317073, 91.9993330792683, 82.76962652439023, 89.61747332317073, 89.91520579268293, 86.34241615853658, 96.76305259146342, 86.34241615853658, 83.66282393292683, 88.72427591463415, 92.2970655487805, 83.66282393292683, 98.84717987804879], [78.6013719512195, 86.34241615853658, 83.96055640243902, 76.21951219512195, 80.0900342987805, 90.51067073170732, 85.44921875, 92.2970655487805, 90.21293826219512, 93.19026295731707, 86.64014862804879, 96.16758765243902, 85.1514862804878, 84.25828887195121, 93.48799542682927, 89.61747332317073, 94.97665777439023, 89.02200838414635, 102.41996951219512, 93.78572789634147, 83.96055640243902, 85.44921875, 89.61747332317073, 81.87642911585365, 92.89253048780488, 84.55602134146342, 91.4038681402439, 88.42654344512195, 90.21293826219512, 91.7016006097561, 83.66282393292683, 81.87642911585365, 89.91520579268293, 86.93788109756098, 93.78572789634147, 103.01543445121952, 89.02200838414635, 99.14491234756098, 94.08346036585365, 89.61747332317073, 80.68549923780488, 101.22903963414633, 74.43311737804879, 90.21293826219512, 94.08346036585365, 90.51067073170732, 89.02200838414635, 96.16758765243902, 84.25828887195121, 86.93788109756098], [94.67892530487805, 87.23561356707317, 85.44921875, 94.97665777439023, 94.97665777439023, 89.61747332317073, 93.78572789634147, 93.19026295731707, 86.34241615853658, 89.02200838414635, 104.80182926829269, 80.0900342987805, 95.86985518292683, 89.31974085365853, 85.1514862804878, 88.72427591463415, 88.12881097560977, 86.0446836890244, 86.64014862804879, 90.51067073170732, 100.63357469512195, 87.53334603658537, 84.8537538109756, 75.92177972560977, 88.42654344512195, 89.61747332317073, 94.08346036585365, 96.16758765243902, 92.89253048780488, 76.51724466463415, 90.51067073170732, 91.9993330792683, 83.06735899390245, 76.21951219512195, 88.12881097560977, 83.36509146341463, 98.2517149390244, 99.44264481707317, 91.4038681402439, 80.0900342987805, 91.9993330792683, 80.98323170731707, 86.34241615853658, 87.83107850609755, 83.66282393292683, 89.31974085365853, 96.76305259146342, 83.96055640243902, 91.7016006097561, 100.63357469512195], [89.31974085365853, 93.48799542682927, 77.70817454268293, 91.1061356707317, 96.16758765243902, 87.53334603658537, 74.43311737804879, 89.02200838414635, 91.1061356707317, 77.41044207317073, 85.7469512195122, 92.59479801829268, 89.31974085365853, 98.54944740853658, 83.96055640243902, 90.8084032012195, 88.72427591463415, 85.44921875, 99.44264481707317, 86.64014862804879, 94.97665777439023, 91.1061356707317, 86.0446836890244, 83.36509146341463, 85.1514862804878, 87.23561356707317, 98.54944740853658, 84.25828887195121, 91.7016006097561, 80.38776676829268, 83.66282393292683, 97.0607850609756, 89.61747332317073, 85.44921875, 84.8537538109756, 86.34241615853658, 82.47189405487805, 95.27439024390245, 87.83107850609755, 86.93788109756098, 88.12881097560977, 94.97665777439023, 100.93130716463415, 84.55602134146342, 90.21293826219512, 83.96055640243902, 80.68549923780488, 83.66282393292683, 82.47189405487805, 84.8537538109756], [89.91520579268293, 83.36509146341463, 88.42654344512195, 93.78572789634147, 88.42654344512195, 86.64014862804879, 88.72427591463415, 81.57869664634147, 92.59479801829268, 95.57212271341463, 86.0446836890244, 94.08346036585365, 83.96055640243902, 84.55602134146342, 92.89253048780488, 97.3585175304878, 87.23561356707317, 92.59479801829268, 87.53334603658537, 86.0446836890244, 85.7469512195122, 93.78572789634147, 91.9993330792683, 88.72427591463415, 89.61747332317073, 96.46532012195121, 80.38776676829268, 97.3585175304878, 86.64014862804879, 88.12881097560977, 89.31974085365853, 87.23561356707317, 95.86985518292683, 88.42654344512195, 78.6013719512195, 97.9539824695122, 97.3585175304878, 81.57869664634147, 95.57212271341463, 84.25828887195121, 95.86985518292683, 85.1514862804878, 100.03810975609757, 91.9993330792683, 96.46532012195121, 88.42654344512195, 88.42654344512195, 83.06735899390245, 86.64014862804879, 84.8537538109756], [86.93788109756098, 97.65625, 101.22903963414633, 89.02200838414635, 76.81497713414635, 93.78572789634147, 89.02200838414635, 97.0607850609756, 86.0446836890244, 96.76305259146342, 92.89253048780488, 93.48799542682927, 78.00590701219512, 87.23561356707317, 83.06735899390245, 106.29049161585367, 85.44921875, 78.8991044207317, 90.8084032012195, 93.19026295731707, 87.83107850609755, 83.36509146341463, 88.12881097560977, 94.97665777439023, 85.1514862804878, 83.36509146341463, 91.1061356707317, 86.64014862804879, 93.48799542682927, 96.76305259146342, 80.98323170731707, 92.59479801829268, 84.55602134146342, 91.4038681402439, 94.08346036585365, 84.25828887195121, 100.63357469512195, 100.63357469512195, 88.72427591463415, 81.87642911585365, 88.12881097560977, 80.98323170731707, 98.84717987804879, 88.42654344512195, 92.2970655487805, 96.16758765243902, 90.21293826219512, 81.28096417682927, 93.19026295731707, 94.38119283536585], [72.9444550304878, 101.22903963414633, 90.8084032012195, 95.86985518292683, 92.89253048780488, 94.97665777439023, 85.1514862804878, 91.1061356707317, 92.59479801829268, 89.31974085365853, 81.87642911585365, 84.55602134146342, 83.06735899390245, 94.08346036585365, 72.05125762195121, 82.17416158536585, 91.9993330792683, 89.02200838414635, 94.38119283536585, 84.25828887195121, 87.23561356707317, 88.72427591463415, 75.32631478658537, 89.91520579268293, 91.7016006097561, 91.4038681402439, 90.8084032012195, 93.19026295731707, 98.84717987804879, 99.14491234756098, 86.0446836890244, 77.11270960365853, 94.67892530487805, 78.6013719512195, 91.9993330792683, 85.44921875, 94.67892530487805, 86.0446836890244, 93.78572789634147, 90.8084032012195, 89.91520579268293, 86.64014862804879, 97.65625, 78.8991044207317, 87.83107850609755, 85.7469512195122, 89.31974085365853, 84.25828887195121, 88.12881097560977, 95.86985518292683], [96.76305259146342, 84.55602134146342, 79.7923018292683, 97.65625, 97.65625, 95.27439024390245, 95.86985518292683, 93.19026295731707, 96.46532012195121, 92.89253048780488, 86.34241615853658, 83.36509146341463, 81.87642911585365, 79.1968368902439, 84.25828887195121, 95.86985518292683, 84.55602134146342, 96.76305259146342, 92.59479801829268, 96.16758765243902, 77.70817454268293, 86.34241615853658, 90.8084032012195, 81.87642911585365, 89.91520579268293, 97.0607850609756, 89.31974085365853, 89.91520579268293, 90.8084032012195, 88.42654344512195, 79.7923018292683, 84.25828887195121, 83.06735899390245, 80.98323170731707, 92.89253048780488, 83.66282393292683, 91.1061356707317, 85.1514862804878, 81.57869664634147, 77.11270960365853, 90.21293826219512, 80.68549923780488, 90.21293826219512, 94.38119283536585, 92.59479801829268, 92.2970655487805, 86.93788109756098, 82.76962652439023, 81.57869664634147, 76.81497713414635], [80.0900342987805, 92.59479801829268, 84.55602134146342, 96.46532012195121, 90.21293826219512, 73.5399199695122, 86.34241615853658, 83.36509146341463, 97.3585175304878, 95.57212271341463, 87.83107850609755, 95.27439024390245, 89.91520579268293, 93.19026295731707, 81.28096417682927, 93.48799542682927, 85.44921875, 84.8537538109756, 103.9086318597561, 93.48799542682927, 101.22903963414633, 83.66282393292683, 84.55602134146342, 97.9539824695122, 92.89253048780488, 86.0446836890244, 91.4038681402439, 91.7016006097561, 93.19026295731707, 86.34241615853658, 86.0446836890244, 83.96055640243902, 85.44921875, 80.0900342987805, 91.1061356707317, 89.61747332317073, 83.96055640243902, 89.02200838414635, 98.2517149390244, 99.44264481707317, 82.47189405487805, 90.21293826219512, 87.53334603658537, 87.23561356707317, 97.65625, 86.0446836890244, 80.38776676829268, 101.82450457317074, 95.57212271341463, 93.19026295731707], [83.36509146341463, 97.0607850609756, 88.72427591463415, 86.93788109756098, 89.91520579268293, 94.67892530487805, 89.91520579268293, 89.61747332317073, 87.83107850609755, 98.54944740853658, 77.70817454268293, 92.89253048780488, 91.1061356707317, 93.48799542682927, 100.03810975609757, 94.67892530487805, 85.1514862804878, 89.02200838414635, 92.89253048780488, 94.08346036585365, 90.8084032012195, 87.83107850609755, 89.91520579268293, 80.0900342987805, 89.91520579268293, 94.67892530487805, 85.7469512195122, 82.17416158536585, 94.08346036585365, 85.44921875, 103.6108993902439, 90.8084032012195, 98.54944740853658, 95.57212271341463, 86.0446836890244, 79.7923018292683, 88.12881097560977, 90.21293826219512, 76.51724466463415, 84.25828887195121, 82.17416158536585, 82.76962652439023, 88.12881097560977, 96.46532012195121, 78.8991044207317, 105.69502667682926, 81.87642911585365, 89.31974085365853, 80.98323170731707, 79.7923018292683], [91.1061356707317, 102.71770198170731, 85.7469512195122, 91.4038681402439, 91.4038681402439, 90.8084032012195, 95.27439024390245, 91.7016006097561, 71.75352515243902, 88.42654344512195, 92.89253048780488, 89.02200838414635, 80.38776676829268, 81.87642911585365, 84.8537538109756, 92.2970655487805, 86.0446836890244, 82.47189405487805, 96.16758765243902, 89.61747332317073, 80.98323170731707, 85.44921875, 86.0446836890244, 97.65625, 109.26781631097562, 98.84717987804879, 88.12881097560977, 82.76962652439023, 84.25828887195121, 91.4038681402439, 88.72427591463415, 78.6013719512195, 96.46532012195121, 89.61747332317073, 89.02200838414635, 84.55602134146342, 95.86985518292683, 90.51067073170732, 85.7469512195122, 94.38119283536585, 92.2970655487805, 88.72427591463415, 87.23561356707317, 88.42654344512195, 82.47189405487805, 88.42654344512195, 82.17416158536585, 85.7469512195122, 88.42654344512195, 99.14491234756098], [78.6013719512195, 103.31316692073172, 82.76962652439023, 82.17416158536585, 82.76962652439023, 83.96055640243902, 90.51067073170732, 85.7469512195122, 94.67892530487805, 89.31974085365853, 83.96055640243902, 84.55602134146342, 82.76962652439023, 103.9086318597561, 88.42654344512195, 95.27439024390245, 87.53334603658537, 82.47189405487805, 81.57869664634147, 90.8084032012195, 88.42654344512195, 95.27439024390245, 89.61747332317073, 81.87642911585365, 90.51067073170732, 95.27439024390245, 96.46532012195121, 88.42654344512195, 96.16758765243902, 80.0900342987805, 94.38119283536585, 90.21293826219512, 88.72427591463415, 93.78572789634147, 86.93788109756098, 82.47189405487805, 78.30363948170732, 81.57869664634147, 91.7016006097561, 86.34241615853658, 89.91520579268293, 84.25828887195121, 79.7923018292683, 92.59479801829268, 90.8084032012195, 98.54944740853658, 85.1514862804878, 85.1514862804878, 100.33584222560977, 101.22903963414633], [80.68549923780488, 83.06735899390245, 87.23561356707317, 95.27439024390245, 82.17416158536585, 94.38119283536585, 89.61747332317073, 105.09956173780488, 92.89253048780488, 84.55602134146342, 81.57869664634147, 82.17416158536585, 85.7469512195122, 100.63357469512195, 89.61747332317073, 102.12223704268293, 82.47189405487805, 91.1061356707317, 83.36509146341463, 91.4038681402439, 93.78572789634147, 94.08346036585365, 91.9993330792683, 86.64014862804879, 97.9539824695122, 92.59479801829268, 87.53334603658537, 85.44921875, 89.02200838414635, 90.8084032012195, 90.21293826219512, 83.36509146341463, 106.58822408536585, 94.67892530487805, 90.51067073170732, 88.42654344512195, 89.02200838414635, 77.70817454268293, 83.66282393292683, 103.9086318597561, 71.45579268292683, 93.19026295731707, 94.38119283536585, 90.8084032012195, 91.1061356707317, 85.7469512195122, 84.8537538109756, 87.53334603658537, 91.7016006097561, 83.96055640243902], [89.02200838414635, 81.57869664634147, 78.8991044207317, 85.44921875, 91.7016006097561, 79.1968368902439, 71.45579268292683, 82.17416158536585, 89.02200838414635, 89.91520579268293, 101.82450457317074, 93.48799542682927, 89.02200838414635, 86.34241615853658, 87.23561356707317, 83.96055640243902, 91.7016006097561, 101.82450457317074, 83.66282393292683, 89.31974085365853, 101.22903963414633, 76.81497713414635, 89.31974085365853, 80.68549923780488, 83.66282393292683, 87.83107850609755, 87.53334603658537, 82.17416158536585, 91.4038681402439, 94.08346036585365, 89.61747332317073, 85.1514862804878, 93.48799542682927, 92.59479801829268, 99.44264481707317, 101.22903963414633, 83.36509146341463, 86.93788109756098, 88.72427591463415, 83.06735899390245, 91.4038681402439, 95.86985518292683, 83.66282393292683, 89.61747332317073, 84.25828887195121, 87.83107850609755, 85.44921875, 100.93130716463415, 97.0607850609756, 89.61747332317073], [87.23561356707317, 78.30363948170732, 90.8084032012195, 89.61747332317073, 97.65625, 88.42654344512195, 89.61747332317073, 89.02200838414635, 86.34241615853658, 84.55602134146342, 89.31974085365853, 93.19026295731707, 88.42654344512195, 91.9993330792683, 89.61747332317073, 88.42654344512195, 90.51067073170732, 80.68549923780488, 84.25828887195121, 87.23561356707317, 92.59479801829268, 91.4038681402439, 96.46532012195121, 90.51067073170732, 86.0446836890244, 78.00590701219512, 87.53334603658537, 95.86985518292683, 83.06735899390245, 86.93788109756098, 97.3585175304878, 91.9993330792683, 86.0446836890244, 98.2517149390244, 88.42654344512195, 90.51067073170732, 94.08346036585365, 90.51067073170732, 79.1968368902439, 80.38776676829268, 86.93788109756098, 91.1061356707317, 91.4038681402439, 85.1514862804878, 94.08346036585365, 84.8537538109756, 88.42654344512195, 96.46532012195121, 92.89253048780488, 92.89253048780488], [87.23561356707317, 78.00590701219512, 77.41044207317073, 80.68549923780488, 79.1968368902439, 93.48799542682927, 89.31974085365853, 88.42654344512195, 87.53334603658537, 92.89253048780488, 83.36509146341463, 88.72427591463415, 83.36509146341463, 86.93788109756098, 84.25828887195121, 78.30363948170732, 86.0446836890244, 87.23561356707317, 83.06735899390245, 83.96055640243902, 89.61747332317073, 83.66282393292683, 84.8537538109756, 78.30363948170732, 97.65625, 90.51067073170732, 83.96055640243902, 89.02200838414635, 78.30363948170732, 82.47189405487805, 91.4038681402439, 86.34241615853658, 82.17416158536585, 82.47189405487805, 83.96055640243902, 96.16758765243902, 87.23561356707317, 78.6013719512195, 93.78572789634147, 82.17416158536585, 81.28096417682927, 87.83107850609755, 79.1968368902439, 84.8537538109756, 91.4038681402439, 93.48799542682927, 80.68549923780488, 82.76962652439023, 90.51067073170732, 84.55602134146342], [96.46532012195121, 91.9993330792683, 87.83107850609755, 96.16758765243902, 82.76962652439023, 89.31974085365853, 82.76962652439023, 97.3585175304878, 85.44921875, 93.19026295731707, 82.76962652439023, 93.78572789634147, 78.8991044207317, 87.23561356707317, 88.72427591463415, 89.91520579268293, 81.28096417682927, 88.42654344512195, 86.34241615853658, 97.9539824695122, 98.54944740853658, 89.61747332317073, 90.21293826219512, 86.34241615853658, 90.51067073170732, 94.38119283536585, 74.13538490853658, 93.78572789634147, 95.57212271341463, 86.93788109756098, 83.96055640243902, 92.59479801829268, 87.53334603658537, 82.76962652439023, 90.8084032012195, 82.76962652439023, 83.36509146341463, 91.4038681402439, 89.91520579268293, 90.51067073170732, 95.57212271341463, 86.34241615853658, 78.00590701219512, 76.81497713414635, 85.7469512195122, 99.14491234756098, 85.44921875, 83.66282393292683, 91.1061356707317, 94.38119283536585], [89.02200838414635, 85.7469512195122, 82.47189405487805, 100.33584222560977, 85.7469512195122, 91.9993330792683, 84.25828887195121, 99.14491234756098, 92.59479801829268, 83.36509146341463, 82.76962652439023, 92.89253048780488, 86.0446836890244, 82.76962652439023, 92.59479801829268, 87.23561356707317, 87.23561356707317, 92.89253048780488, 91.9993330792683, 89.31974085365853, 95.86985518292683, 77.11270960365853, 101.52677210365854, 95.27439024390245, 94.38119283536585, 88.42654344512195, 89.31974085365853, 88.72427591463415, 86.34241615853658, 100.03810975609757, 98.2517149390244, 90.8084032012195, 90.8084032012195, 78.30363948170732, 89.91520579268293, 90.8084032012195, 86.93788109756098, 82.17416158536585, 86.34241615853658, 80.0900342987805, 97.9539824695122, 95.86985518292683, 105.39729420731707, 89.61747332317073, 89.02200838414635, 92.59479801829268, 91.9993330792683, 94.08346036585365, 88.72427591463415, 94.67892530487805]]
  out "CH2":dbl[][](graph)=[[0.2977324695121951, 0.5954649390243902, 0.0, 0.0, 0.5954649390243902, 0.2977324695121951, 0.0, 0.2977324695121951, 0.5954649390243902, 0.8931974085365854, 0.0, 0.2977324695121951, 0.2977324695121951, 0.0, 0.0, 0.5954649390243902, 0.2977324695121951, 0.2977324695121951, 0.2977324695121951, 0.8931974085365854, 5.656916920731708, 0.0, 0.5954649390243902, 0.2977324695121951, 0.5954649390243902, 0.0, 0.2977324695121951, 0.0, 0.0, 0.5954649390243902, 0.2977324695121951, 1.1909298780487805, 0.0, 0.0, 0.5954649390243902, 2.0841272865853657, 0.2977324695121951, 0.5954649390243902, 0.5954649390243902, 0.0, 0.0, 0.0, 0.2977324695121951, 0.0, 0.0, 0.0, 0.0, 0.0, 0.5954649390243902, 0.2977324695121951], [0.2977324695121951, 0.0, 0.2977324695121951, 0.0, 0.0, 0.2977324695121951, 0.0, 0.0, 0.0, 1.7863948170731707, 0.0, 0.2977324695121951, 0.5954649390243902, 0.0, 0.2977324695121951, 4.763719512195122, 0.0, 0.8931974085365854, 0.0, 0.2977324695121951, 0.0, 0.0, 0.0, 0.2977324695121951, 0.0, 0.0, 0.5954649390243902, 0.0, 0.0, 0.0, 0.0, 0.0, 5.061451981707317, 0.2977324695121951, 0.0, 1.1909298780487805, 0.0, 0.2977324695121951, 0.2977324695121951, 1.7863948170731707, 0.0, 0.2977324695121951, 1.1909298780487805, 0.0, 0.0, 0.0, 0.0, 0.2977324695121951, 0.0, 0.0], [0.5954649390243902, 0.0, 0.2977324695121951, 0.0, 0.0, 0.0, 0.2977324695121951, 0.0, 0.5954649390243902, 0.0, 0.0, 0.0, 0.0, 0.2977324695121951, 0.0, 0.0, 0.0, 3.2750571646341466, 0.8931974085365854, 0.2977324695121951, 0.0, 0.0, 0.5954649390243902, 0.2977324695121951, 0.2977324695121951, 0.0, 0.5954649390243902, 0.0, 0.2977324695121951, 0.8931974085365854, 0.2977324695121951, 0.8931974085365854, 0.0, 1.7863948170731707, 0.0, 0.0, 0.2977324695121951, 0.5954649390243902, 2.0841272865853657, 0.0, 0.0, 0.0, 0.0, 0.5954649390243902, 0.5954649390243902, 0.0, 0.2977324695121951, 0.5954649390243902, 0.0, 0.2977324695121951], [0.0, 0.2977324695121951, 0.0, 0.0, 0.0, 2.679592225609756, 0.5954649390243902, 0.2977324695121951, 0.2977324695121951, 0.8931974085365854, 0.5954649390243902, 0.0, 0.2977324695121951, 0.0, 0.0, 0.2977324695121951, 0.0, 0.2977324695121951, 0.0, 0.0, 0.0, 0.0, 0.2977324695121951, 0.2977324695121951, 0.2977324695121951, 0.0, 0.0, 0.0, 0.5954649390243902, 0.0, 0.2977324695121951, 0.0, 0.0, 0.0, 0.2977324695121951, 0.2977324695121951, 0.0, 0.2977324695121951, 0.8931974085365854, 0.0, 0.0, 1.1909298780487805, 0.0, 0.2977324695121951, 0.2977324695121951, 0.0, 0.2977324695121951, 0.2977324695121951, 2.0841272865853657, 0.2977324695121951], [0.2977324695121951, 0.2977324695121951, 0.2977324695121951, 0.0, 0.0, 0.2977324695121951, 0.0, 0.0, 0.0, 0.0, 0.0, 0.0, 0.2977324695121951, 0.0, 0.0, 0.0, 0.0, 0.2977324695121951, 0.0, 0.0, 0.2977324695121951, 0.0, 0.0, 0.0, 0.0, 0.5954649390243902, 0.0, 0.0, 0.8931974085365854, 0.0, 0.2977324695121951, 0.0, 1.7863948170731707, 0.8931974085365854, 0.5954649390243902, 0.0, 0.2977324695121951, 0.2977324695121951, 0.2977324695121951, 0.0, 2.679592225609756, 0.0, 0.0, 4.1682545731707314, 1.1909298780487805, 1.4886623475609757, 0.0, 0.0, 0.0, 0.2977324695121951], [0.2977324695121951, 0.0, 0.0, 0.2977324695121951, 0.0, 0.0, 0.0, 0.0, 0.0, 0.0, 0.2977324695121951, 0.0, 0.2977324695121951, 0.2977324695121951, 0.2977324695121951, 0.0, 0.0, 0.2977324695121951, 0.2977324695121951, 0.0, 0.0, 0.0, 0.0, 0.2977324695121951, 2.0841272865853657, 0.0, 0.5954649390243902, 0.0, 0.5954649390243902, 2.9773246951219514, 0.2977324695121951, 0.2977324695121951, 0.0, 0.2977324695121951, 0.2977324695121951, 0.0, 0.0, 3.5727896341463414, 0.0, 0.0, 0.2977324695121951, 0.2977324695121951, 0.2977324695121951, 0.0, 0.2977324695121951, 0.0, 0.0, 0.0, 0.0, 0.0], [0.0, 0.0, 0.5954649390243902, 0.5954649390243902, 0.0, 0.2977324695121951, 0.0, 0.0, 0.0, 0.2977324695121951, 0.0, 0.8931974085365854, 0.2977324695121951, 0.5954649390243902, 0.0, 0.0, 0.2977324695121951, 0.2977324695121951, 1.4886623475609757, 0.2977324695121951, 0.0, 0.0, 0.0, 0.0, 0.0, 0.0, 0.2977324695121951, 0.0, 0.0, 0.0, 0.0, 0.2977324695121951, 0.0, 0.0, 0.0, 0.2977324695121951, 0.5954649390243902, 0.0, 0.5954649390243902, 0.0, 0.0, 0.0, 0.0, 0.0, 0.0, 1.4886623475609757, 0.0, 0.2977324695121951, 0.0, 0.2977324695121951], [0.2977324695121951, 0.2977324695121951, 0.0, 0.0, 0.0, 0.0, 0.0, 0.2977324695121951, 0.2977324695121951, 2.9773246951219514, 0.0, 0.0, 2.0841272865853657, 0.0, 0.0, 0.0, 0.0, 0.0, 0.5954649390243902, 0.2977324695121951, 2.381859756097561, 2.9773246951219514, 0.2977324695121951, 0.0, 0.0, 0.0, 0.0, 0.8931974085365854, 0.0, 0.8931974085365854, 0.0, 0.0, 0.2977324695121951, 0.5954649390243902, 0.0, 0.0, 0.0, 0.0, 0.0, 0.0, 0.5954649390243902, 0.5954649390243902, 0.2977324695121951, 1.4886623475609757, 0.2977324695121951, 0.0, 0.0, 0.2977324695121951, 0.2977324695121951, 0.0], [0.0, 0.0, 0.2977324695121951, 0.2977324695121951, 5.359184451219512, 0.0, 0.5954649390243902, 0.0, 0.2977324695121951, 2.381859756097561, 0.2977324695121951, 0.0, 0.2977324695121951, 0.5954649390243902, 0.2977324695121951, 1.1909298780487805, 0.0, 0.5954649390243902, 0.2977324695121951, 0.5954649390243902, 0.0, 0.0, 0.2977324695121951, 1.1909298780487805, 0.2977324695121951, 0.2977324695121951, 0.0, 0.0, 0.0, 0.5954649390243902, 0.8931974085365854, 0.0, 0.2977324695121951, 0.5954649390243902, 0.0, 0.0, 0.8931974085365854, 0.2977324695121951, 0.0, 0.8931974085365854, 0.5954649390243902, 0.2977324695121951, 0.0, 0.2977324695121951, 0.0, 0.2977324695121951, 0.2977324695121951, 0.0, 0.8931974085365854, 0.2977324695121951], [0.5954649390243902, 0.0, 0.0, 0.0, 0.0, 0.0, 0.0, 0.2977324695121951, 0.0, 0.2977324695121951, 0.2977324695121951, 0.0, 0.2977324695121951, 0.5954649390243902, 0.2977324695121951, 0.0, 0.2977324695121951, 0.0, 0.8931974085365854, 0.0, 0.5954649390243902, 0.0, 0.8931974085365854, 0.5954649390243902, 0.2977324695121951, 0.0, 0.0, 0.2977324695121951, 0.8931974085365854, 0.0, 5.359184451219512, 0.0, 0.8931974085365854, 0.0, 0.2977324695121951, 0.2977324695121951, 0.2977324695121951, 2.0841272865853657, 1.1909298780487805, 0.0, 0.0, 0.0, 0.2977324695121951, 0.8931974085365854, 0.2977324695121951, 0.0, 0.2977324695121951, 0.2977324695121951, 1.7863948170731707, 0.0], [0.0, 0.0, 0.0, 0.2977324695121951, 0.0, 0.0, 0.2977324695121951, 0.0, 0.0, 0.0, 0.5954649390243902, 0.5954649390243902, 2.9773246951219514, 0.8931974085365854, 1.7863948170731707, 0.5954649390243902, 0.2977324695121951, 0.0, 0.5954649390243902, 0.2977324695121951, 0.5954649390243902, 0.0, 0.0, 0.0, 0.5954649390243902, 0.0, 0.5954649390243902, 0.5954649390243902, 0.0, 0.5954649390243902, 0.2977324695121951, 0.5954649390243902, 0.5954649390243902, 0.2977324695121951, 0.2977324695121951, 0.5954649390243902, 0.2977324695121951, 0.0, 0.0, 0.0, 0.2977324695121951, 0.0, 0.0, 1.4886623475609757, 0.2977324695121951, 0.2977324695121951, 0.0, 0.5954649390243902, 0.5954649390243902, 0.0], [0.2977324695121951, 0.0, 0.2977324695121951, 0.5954649390243902, 0.2977324695121951, 0.2977324695121951, 0.5954649390243902, 0.0, 0.5954649390243902, 0.0, 0.2977324695121951, 2.679592225609756, 0.0, 0.0, 0.8931974085365854, 0.5954649390243902, 0.2977324695121951, 0.0, 0.0, 0.0, 0.2977324695121951, 5.656916920731708, 0.0, 0.8931974085365854, 0.0, 0.5954649390243902, 0.0, 0.2977324695121951, 1.1909298780487805, 0.0, 0.0, 0.0, 0.0, 0.0, 0.2977324695121951, 0.2977324695121951, 0.0, 0.0, 0.0, 0.2977324695121951, 1.4886623475609757, 0.2977324695121951, 0.2977324695121951, 0.2977324695121951, 0.0, 0.2977324695121951, 0.0, 0.0, 0.0, 0.8931974085365854], [0.0, 0.8931974085365854, 0.0, 0.2977324695121951, 0.0, 0.2977324695121951, 0.2977324695121951, 0.0, 0.5954649390243902, 0.0, 0.2977324695121951, 0.0, 0.0, 0.0, 1.4886623475609757, 0.2977324695121951, 0.5954649390243902, 0.0, 0.0, 0.0, 0.0, 1.1909298780487805, 0.0, 0.2977324695121951, 0.0, 0.0, 0.2977324695121951, 1.1909298780487805, 0.0, 0.2977324695121951, 0.5954649390243902, 0.2977324695121951, 0.0, 0.0, 0.2977324695121951, 0.0, 0.5954649390243902, 0.0, 0.2977324695121951, 0.0, 0.0, 0.0, 0.0, 0.5954649390243902, 0.2977324695121951, 0.2977324695121951, 0.0, 0.2977324695121951, 0.2977324695121951, 0.0], [0.2977324695121951, 0.0, 0.0, 0.0, 0.2977324695121951, 0.0, 0.2977324695121951, 1.1909298780487805, 0.2977324695121951, 0.0, 0.0, 0.2977324695121951, 0.0, 0.5954649390243902, 0.0, 0.0, 0.0, 0.0, 0.0, 0.0, 0.5954649390243902, 0.0, 0.2977324695121951, 0.5954649390243902, 0.0, 0.0, 0.2977324695121951, 0.0, 0.2977324695121951, 0.2977324695121951, 1.4886623475609757, 0.2977324695121951, 0.2977324695121951, 0.2977324695121951, 0.2977324695121951, 0.2977324695121951, 0.5954649390243902, 0.0, 0.0, 0.5954649390243902, 0.0, 0.0, 0.0, 0.2977324695121951, 0.0, 0.2977324695121951, 0.0, 0.2977324695121951, 0.2977324695121951, 0.2977324695121951], [0.2977324695121951, 0.2977324695121951, 0.5954649390243902, 0.0, 0.0, 2.679592225609756, 0.0, 0.8931974085365854, 0.2977324695121951, 0.0, 1.1909298780487805, 0.0, 0.5954649390243902, 0.5954649390243902, 0.0, 0.2977324695121951, 0.2977324695121951, 1.4886623475609757, 0.0, 1.1909298780487805, 0.5954649390243902, 0.0, 0.2977324695121951, 1.4886623475609757, 0.2977324695121951, 0.0, 1.1909298780487805, 0.5954649390243902, 0.2977324695121951, 0.0, 0.2977324695121951, 0.0, 0.0, 0.2977324695121951, 0.2977324695121951, 0.2977324695121951, 0.2977324695121951, 0.2977324695121951, 0.0, 0.2977324695121951, 0.5954649390243902, 2.679592225609756, 0.2977324695121951, 0.2977324695121951, 0.2977324695121951, 0.2977324695121951, 0.5954649390243902, 0.0, 0.2977324695121951, 1.1909298780487805], [0.0, 0.2977324695121951, 0.0, 0.0, 2.381859756097561, 0.8931974085365854, 0.0, 1.7863948170731707, 0.0, 0.0, 0.0, 0.0, 0.0, 0.5954649390243902, 0.2977324695121951, 0.0, 0.5954649390243902, 0.0, 0.0, 0.0, 0.8931974085365854, 9.527439024390244, 0.0, 0.2977324695121951, 0.2977324695121951, 0.2977324695121951, 0.0, 0.0, 0.2977324695121951, 0.2977324695121951, 0.0, 0.0, 0.0, 1.4886623475609757, 0.8931974085365854, 1.1909298780487805, 0.5954649390243902, 0.0, 0.2977324695121951, 0.0, 0.0, 0.2977324695121951, 0.2977324695121951, 0.2977324695121951, 0.0, 1.7863948170731707, 0.2977324695121951, 0.5954649390243902, 0.0, 0.0], [0.0, 0.2977324695121951, 0.0, 0.0, 0.0, 0.0, 0.2977324695121951, 0.0, 0.2977324695121951, 0.0, 0.5954649390243902, 0.0, 0.0, 0.2977324695121951, 0.8931974085365854, 1.1909298780487805, 0.2977324695121951, 0.2977324695121951, 0.0, 0.2977324695121951, 0.2977324695121951, 1.4886623475609757, 0.2977324695121951, 0.2977324695121951, 0.2977324695121951, 0.0, 0.2977324695121951, 0.0, 0.8931974085365854, 0.8931974085365854, 0.0, 0.0, 0.0, 0.2977324695121951, 0.5954649390243902, 0.8931974085365854, 0.8931974085365854, 0.0, 0.0, 0.0, 0.0, 0.0, 0.2977324695121951, 0.2977324695121951, 0.2977324695121951, 0.0, 0.2977324695121951, 0.0, 0.0, 0.0], [3.2750571646341466, 0.5954649390243902, 0.2977324695121951, 0.0, 0.2977324695121951, 0.2977324695121951, 2.9773246951219514, 0.0, 0.0, 0.2977324695121951, 0.0, 0.0, 0.0, 0.0, 0.0, 0.2977324695121951, 0.0, 0.2977324695121951, 2.381859756097561, 4.465987042682927, 0.8931974085365854, 0.2977324695121951, 0.2977324695121951, 0.2977324695121951, 2.381859756097561, 0.2977324695121951, 0.0, 0.0, 0.0, 0.2977324695121951, 1.4886623475609757, 0.0, 0.0, 0.0, 0.0, 0.0, 0.0, 0.2977324695121951, 0.0, 0.5954649390243902, 0.2977324695121951, 2.381859756097561, 0.0, 0.0, 0.0, 0.0, 0.0, 0.0, 0.0, 0.2977324695121951], [0.2977324695121951, 0.0, 0.0, 0.0, 0.2977324695121951, 0.2977324695121951, 0.5954649390243902, 0.5954649390243902, 0.2977324695121951, 3.2750571646341466, 0.2977324695121951, 0.8931974085365854, 0.8931974085365854, 0.0, 0.0, 0.0, 0.2977324695121951, 0.5954649390243902, 0.5954649390243902, 0.0, 2.679592225609756, 0.0, 0.0, 0.2977324695121951, 0.2977324695121951, 0.0, 0.0, 0.2977324695121951, 0.5954649390243902, 0.5954649390243902, 0.2977324695121951, 0.2977324695121951, 0.0, 3.5727896341463414, 0.8931974085365854, 0.0, 0.2977324695121951, 0.2977324695121951, 0.0, 0.2977324695121951, 0.0, 1.1909298780487805, 0.2977324695121951, 0.2977324695121951, 0.0, 0.5954649390243902, 0.5954649390243902, 0.0, 0.2977324695121951, 0.5954649390243902], [0.0, 0.0, 0.2977324695121951, 0.0, 0.0, 0.2977324695121951, 0.0, 0.5954649390243902, 0.0, 0.2977324695121951, 0.0, 0.0, 0.0, 0.0, 1.4886623475609757, 2.0841272865853657, 0.2977324695121951, 9.527439024390244, 0.0, 0.8931974085365854, 0.0, 0.0, 0.0, 0.2977324695121951, 0.2977324695121951, 0.2977324695121951, 0.8931974085365854, 0.2977324695121951, 0.2977324695121951, 0.0, 0.2977324695121951, 0.8931974085365854, 0.0, 0.0, 0.2977324695121951, 0.8931974085365854, 0.0, 0.8931974085365854, 0.0, 0.0, 0.0, 0.0, 0.0, 0.0, 0.0, 0.2977324695121951, 0.2977324695121951, 0.0, 0.2977324695121951, 0.0], [0.0, 0.2977324695121951, 0.0, 0.2977324695121951, 0.2977324695121951, 0.0, 0.2977324695121951, 0.0, 0.0, 0.2977324695121951, 0.2977324695121951, 0.8931974085365854, 0.2977324695121951, 0.8931974085365854, 0.2977324695121951, 0.0, 0.2977324695121951, 0.2977324695121951, 0.5954649390243902, 1.7863948170731707, 0.2977324695121951, 0.2977324695121951, 0.2977324695121951, 0.2977324695121951, 0.0, 0.0, 0.2977324695121951, 0.2977324695121951, 0.8931974085365854, 0.0, 0.2977324695121951, 0.2977324695121951, 0.0, 0.2977324695121951, 0.0, 1.1909298780487805, 1.1909298780487805, 0.2977324695121951, 0.0, 0.2977324695121951, 0.0, 0.2977324695121951, 1.1909298780487805, 0.2977324695121951, 0.8931974085365854, 0.2977324695121951, 0.0, 0.0, 0.0, 0.0], [2.679592225609756, 0.8931974085365854, 0.2977324695121951, 0.0, 0.0, 0.0, 0.0, 1.1909298780487805, 2.9773246951219514, 0.2977324695121951, 2.381859756097561, 0.0, 0.2977324695121951, 0.2977324695121951, 1.7863948170731707, 0.8931974085365854, 0.0, 0.0, 0.0, 0.5954649390243902, 0.2977324695121951, 0.2977324695121951, 0.0, 0.0, 0.2977324695121951, 0.0, 0.0, 0.0, 0.0, 0.0, 0.5954649390243902, 0.0, 0.0, 0.0, 0.0, 2.679592225609756, 0.2977324695121951, 0.0, 0.0, 0.0, 0.2977324695121951, 0.2977324695121951, 0.2977324695121951, 0.0, 0.0, 0.0, 0.2977324695121951, 0.2977324695121951, 0.8931974085365854, 0.0], [0.0, 0.2977324695121951, 0.0, 0.8931974085365854, 0.2977324695121951, 0.0, 0.2977324695121951, 0.0, 0.0, 0.2977324695121951, 1.4886623475609757, 1.4886623475609757, 0.2977324695121951, 0.0, 0.0, 1.1909298780487805, 0.5954649390243902, 0.5954649390243902, 0.2977324695121951, 0.0, 0.0, 0.0, 0.2977324695121951, 0.8931974085365854, 0.2977324695121951, 0.0, 0.0, 0.0, 0.0, 0.0, 0.2977324695121951, 0.0, 0.2977324695121951, 5.061451981707317, 0.2977324695121951, 0.2977324695121951, 0.2977324695121951, 0.0, 0.0, 0.0, 0.0, 0.0, 0.8931974085365854, 0.2977324695121951, 0.2977324695121951, 0.2977324695121951, 0.8931974085365854, 0.0, 0.5954649390243902, 0.0], [0.0, 0.2977324695121951, 0.2977324695121951, 0.2977324695121951, 0.0, 0.2977324695121951, 0.5954649390243902, 0.0, 0.5954649390243902, 2.0841272865853657, 0.0, 0.0, 0.5954649390243902, 0.0, 0.8931974085365854, 0.0, 1.7863948170731707, 0.8931974085365854, 0.2977324695121951, 0.0, 0.5954649390243902, 0.2977324695121951, 2.381859756097561, 0.2977324695121951, 0.2977324695121951, 0.2977324695121951, 0.0, 2.9773246951219514, 0.2977324695121951, 0.0, 0.0, 0.0, 0.2977324695121951, 0.2977324695121951, 0.0, 0.2977324695121951, 0.0, 0.0, 0.0, 0.0, 0.8931974085365854, 0.2977324695121951, 0.2977324695121951, 0.2977324695121951, 0.2977324695121951, 3.5727896341463414, 0.5954649390243902, 0.0, 0.2977324695121951, 1.7863948170731707], [0.0, 0.0, 0.0, 0.0, 0.0, 0.0, 0.5954649390243902, 0.8931974085365854, 0.0, 2.679592225609756, 0.2977324695121951, 0.0, 0.0, 0.5954649390243902, 2.0841272865853657, 0.0, 0.2977324695121951, 1.1909298780487805, 0.0, 0.2977324695121951, 0.0, 0.2977324695121951, 0.0, 0.2977324695121951, 0.2977324695121951, 0.0, 0.2977324695121951, 0.0, 1.1909298780487805, 0.0, 0.5954649390243902, 0.0, 1.1909298780487805, 1.4886623475609757, 0.0, 1.7863948170731707, 0.0, 0.2977324695121951, 0.5954649390243902, 0.2977324695121951, 0.2977324695121951, 0.2977324695121951, 0.0, 2.679592225609756, 3.5727896341463414, 0.2977324695121951, 0.5954649390243902, 2.679592225609756, 0.0, 0.2977324695121951], [0.2977324695121951, 0.2977324695121951, 0.5954649390243902, 0.0, 0.0, 0.0, 0.5954649390243902, 0.0, 0.2977324695121951, 0.0, 0.5954649390243902, 0.0, 0.0, 0.0, 0.5954649390243902, 0.2977324695121951, 0.0, 0.8931974085365854, 0.0, 0.0, 0.0, 0.0, 0.2977324695121951, 1.7863948170731707, 0.0, 0.2977324695121951, 0.0, 0.5954649390243902, 0.2977324695121951, 0.2977324695121951, 0.0, 0.0, 0.0, 0.0, 1.4886623475609757, 2.0841272865853657, 0.5954649390243902, 0.2977324695121951, 0.2977324695121951, 0.0, 0.2977324695121951, 0.0, 0.0, 0.2977324695121951, 0.0, 0.0, 0.0, 1.4886623475609757, 2.679592225609756, 0.0], [0.2977324695121951, 0.2977324695121951, 0.0, 4.1682545731707314, 0.0, 0.0, 0.5954649390243902, 0.2977324695121951, 0.0, 1.4886623475609757, 0.2977324695121951, 0.5954649390243902, 0.2977324695121951, 0.5954649390243902, 0.2977324695121951, 0.2977324695121951, 0.0, 0.8931974085365854, 0.8931974085365854, 0.0, 0.2977324695121951, 0.2977324695121951, 0.0, 0.0, 0.2977324695121951, 0.8931974085365854, 0.2977324695121951, 0.2977324695121951, 0.0, 0.0, 0.2977324695121951, 0.0, 0.0, 0.0, 0.0, 0.8931974085365854, 0.0, 1.4886623475609757, 3.5727896341463414, 0.0, 0.0, 0.0, 0.0, 0.0, 0.0, 0.2977324695121951, 0.0, 0.0, 1.7863948170731707, 0.0], [0.5954649390243902, 0.2977324695121951, 0.2977324695121951, 0.5954649390243902, 0.0, 0.2977324695121951, 0.5954649390243902, 1.7863948170731707, 0.2977324695121951, 0.0, 0.2977324695121951, 0.0, 1.1909298780487805, 0.0, 0.5954649390243902, 0.0, 0.2977324695121951, 0.2977324695121951, 0.2977324695121951, 0.2977324695121951, 0.2977324695121951, 0.0, 2.679592225609756, 0.0, 1.1909298780487805, 0.2977324695121951, 1.7863948170731707, 0.0, 0.0, 0.2977324695121951, 0.0, 0.2977324695121951, 0.2977324695121951, 0.2977324695121951, 0.8931974085365854, 0.5954649390243902, 0.2977324695121951, 0.5954649390243902, 1.1909298780487805, 0.0, 0.0, 0.0, 0.0, 1.1909298780487805, 0.0, 1.4886623475609757, 2.679592225609756, 0.2977324695121951, 1.4886623475609757, 0.2977324695121951], [0.2977324695121951, 0.0, 0.2977324695121951, 0.2977324695121951, 0.0, 1.4886623475609757, 0.2977324695121951, 0.0, 0.0, 0.2977324695121951, 0.0, 2.381859756097561, 0.2977324695121951, 0.0, 2.381859756097561, 0.0, 0.2977324695121951, 0.0, 0.0, 0.2977324695121951, 2.0841272865853657, 0.5954649390243902, 0.5954649390243902, 1.4886623475609757, 0.0, 0.2977324695121951, 0.0, 0.0, 0.0, 0.0, 0.0, 0.2977324695121951, 0.8931974085365854, 0.0, 0.0, 0.2977324695121951, 0.2977324695121951, 0.0, 5.359184451219512, 0.2977324695121951, 1.7863948170731707, 1.1909298780487805, 0.2977324695121951, 1.4886623475609757, 0.2977324695121951, 0.0, 0.0, 0.0, 0.2977324695121951, 0.0], [0.0, 0.2977324695121951, 0.0, 0.0, 1.7863948170731707, 0.0, 0.5954649390243902, 0.2977324695121951, 0.5954649390243902, 0.0, 5.061451981707317, 0.8931974085365854, 0.0, 0.0, 0.0, 0.2977324695121951, 0.0, 0.2977324695121951, 0.5954649390243902, 0.0, 0.2977324695121951, 0.2977324695121951, 0.0, 0.2977324695121951, 0.2977324695121951, 0.2977324695121951, 0.0, 0.2977324695121951, 0.0, 0.0, 0.0, 0.0, 0.0, 0.0, 0.2977324695121951, 0.5954649390243902, 0.0, 2.679592225609756, 0.5954649390243902, 0.0, 0.2977324695121951, 0.5954649390243902, 0.2977324695121951, 0.5954649390243902, 0.0, 0.0, 0.0, 0.2977324695121951, 0.5954649390243902, 2.381859756097561], [0.2977324695121951, 0.5954649390243902, 0.0, 0.2977324695121951, 0.2977324695121951, 2.381859756097561, 0.2977324695121951, 0.2977324695121951, 1.1909298780487805, 0.2977324695121951, 0.2977324695121951, 2.9773246951219514, 0.5954649390243902, 0.2977324695121951, 0.2977324695121951, 0.0, 0.5954649390243902, 3.8705221036585367, 0.0, 0.2977324695121951, 0.2977324695121951, 0.0, 0.2977324695121951, 0.2977324695121951, 0.2977324695121951, 0.2977324695121951, 0.2977324695121951, 0.2977324695121951, 0.0, 0.0, 0.2977324695121951, 0.2977324695121951, 0.2977324695121951, 0.0, 0.2977324695121951, 0.0, 0.0, 1.1909298780487805, 1.7863948170731707, 0.2977324695121951, 0.2977324695121951, 0.2977324695121951, 0.2977324695121951, 0.2977324695121951, 0.2977324695121951, 0.2977324695121951, 0.2977324695121951, 0.0, 0.2977324695121951, 0.5954649390243902], [0.2977324695121951, 0.0, 0.5954649390243902, 0.0, 0.2977324695121951, 0.0, 0.2977324695121951, 0.2977324695121951, 0.2977324695121951, 0.0, 0.2977324695121951, 0.0, 0.0, 0.5954649390243902, 1.4886623475609757, 0.2977324695121951, 0.0, 0.5954649390243902, 0.5954649390243902, 0.5954649390243902, 0.0, 0.8931974085365854, 0.2977324695121951, 0.0, 0.5954649390243902, 0.2977324695121951, 0.0, 0.2977324695121951, 1.1909298780487805, 0.2977324695121951, 0.8931974085365854, 0.2977324695121951, 0.0, 0.8931974085365854, 0.0, 0.0, 1.4886623475609757, 0.0, 0.2977324695121951, 2.381859756097561, 0.2977324695121951, 1.1909298780487805, 0.2977324695121951, 2.381859756097561, 0.0, 0.0, 1.1909298780487805, 0.0, 0.0, 0.2977324695121951], [0.2977324695121951, 1.4886623475609757, 0.0, 0.0, 0.2977324695121951, 0.5954649390243902, 0.2977324695121951, 0.2977324695121951, 0.2977324695121951, 0.2977324695121951, 0.5954649390243902, 0.2977324695121951, 0.5954649390243902, 0.2977324695121951, 0.0, 0.2977324695121951, 0.2977324695121951, 0.0, 0.0, 0.2977324695121951, 0.2977324695121951, 0.2977324695121951, 0.0, 0.2977324695121951, 0.0, 0.0, 0.2977324695121951, 0.0, 0.0, 0.2977324695121951, 0.0, 0.0, 0.5954649390243902, 0.8931974085365854, 0.0, 0.0, 0.2977324695121951, 0.2977324695121951, 0.0, 0.2977324695121951, 0.2977324695121951, 0.0, 2.9773246951219514, 1.1909298780487805, 0.0, 0.2977324695121951, 0.0, 0.2977324695121951, 0.2977324695121951, 0.2977324695121951], [0.2977324695121951, 0.2977324695121951, 0.0, 0.0, 0.0, 0.0, 3.2750571646341466, 0.8931974085365854, 0.0, 0.2977324695121951, 0.0, 0.2977324695121951, 0.2977324695121951, 0.2977324695121951, 0.0, 0.2977324695121951, 0.2977324695121951, 0.0, 0.0, 0.0, 0.0, 0.5954649390243902, 0.0, 0.0, 0.0, 0.0, 0.5954649390243902, 2.0841272865853657, 0.0, 0.2977324695121951, 2.0841272865853657, 0.0, 0.2977324695121951, 0.2977324695121951, 0.0, 3.5727896341463414, 0.2977324695121951, 0.8931974085365854, 2.9773246951219514, 3.5727896341463414, 0.0, 0.0, 0.0, 0.5954649390243902, 0.8931974085365854, 0.2977324695121951, 0.5954649390243902, 0.0, 0.5954649390243902, 0.2977324695121951], [0.0, 0.0, 0.2977324695121951, 0.0, 0.2977324695121951, 0.2977324695121951, 0.0, 0.5954649390243902, 0.0, 2.381859756097561, 4.1682545731707314, 0.2977324695121951, 0.0, 0.8931974085365854, 0.2977324695121951, 0.2977324695121951, 0.8931974085365854, 0.0, 0.0, 0.0, 3.2750571646341466, 0.0, 0.2977324695121951, 0.0, 0.2977324695121951, 0.0, 0.2977324695121951, 0.5954649390243902, 0.0, 0.0, 0.0, 3.2750571646341466, 0.0, 0.2977324695121951, 0.2977324695121951, 0.2977324695121951, 0.0, 4.763719512195122, 0.5954649390243902, 0.2977324695121951, 0.2977324695121951, 0.0, 0.0, 2.0841272865853657, 1.7863948170731707, 1.7863948170731707, 0.0, 0.0, 0.0, 0.0], [0.8931974085365854, 2.0841272865853657, 0.2977324695121951, 0.0, 0.0, 0.0, 0.0, 0.0, 0.8931974085365854, 2.381859756097561, 2.9773246951219514, 0.0, 0.0, 0.2977324695121951, 0.2977324695121951, 0.0, 0.0, 0.0, 0.0, 0.5954649390243902, 0.0, 0.0, 0.0, 0.0, 0.0, 0.2977324695121951, 1.1909298780487805, 0.0, 0.0, 0.5954649390243902, 0.0, 0.0, 0.0, 0.0, 0.2977324695121951, 0.2977324695121951, 0.8931974085365854, 0.2977324695121951, 0.8931974085365854, 0.0, 0.8931974085365854, 0.0, 0.5954649390243902, 0.8931974085365854, 1.1909298780487805, 0.5954649390243902, 0.8931974085365854, 0.5954649390243902, 0.8931974085365854, 0.0], [0.5954649390243902, 1.4886623475609757, 0.8931974085365854, 0.5954649390243902, 0.0, 1.7863948170731707, 0.2977324695121951, 0.5954649390243902, 0.0, 0.8931974085365854, 0.0, 0.0, 0.0, 2.0841272865853657, 0.0, 0.2977324695121951, 1.7863948170731707, 0.0, 0.0, 1.7863948170731707, 0.2977324695121951, 0.8931974085365854, 0.5954649390243902, 2.0841272865853657, 0.5954649390243902, 1.4886623475609757, 0.2977324695121951, 0.0, 0.2977324695121951, 0.2977324695121951, 1.1909298780487805, 0.2977324695121951, 0.2977324695121951, 0.5954649390243902, 2.9773246951219514, 2.9773246951219514, 0.2977324695121951, 0.2977324695121951, 0.2977324695121951, 0.2977324695121951, 0.0, 0.0, 0.2977324695121951, 0.5954649390243902, 0.0, 0.2977324695121951, 0.0, 0.0, 0.0, 0.2977324695121951], [0.8931974085365854, 0.0, 0.2977324695121951, 0.0, 0.2977324695121951, 0.2977324695121951, 0.0, 0.0, 0.2977324695121951, 0.5954649390243902, 0.5954649390243902, 0.0, 0.2977324695121951, 0.2977324695121951, 1.4886623475609757, 0.0, 1.7863948170731707, 0.2977324695121951, 0.5954649390243902, 0.5954649390243902, 0.0, 0.0, 0.0, 0.2977324695121951, 0.0, 0.0, 0.0, 3.2750571646341466, 0.2977324695121951, 0.2977324695121951, 0.0, 0.2977324695121951, 0.5954649390243902, 0.0, 0.0, 0.2977324695121951, 0.2977324695121951, 0.0, 0.2977324695121951, 0.2977324695121951, 0.0, 0.2977324695121951, 0.0, 0.0, 0.2977324695121951, 0.2977324695121951, 0.2977324695121951, 0.8931974085365854, 0.0, 0.0], [0.2977324695121951, 0.2977324695121951, 0.0, 0.5954649390243902, 2.381859756097561, 1.7863948170731707, 0.2977324695121951, 0.0, 1.4886623475609757, 0.2977324695121951, 0.2977324695121951, 0.0, 0.0, 0.0, 0.2977324695121951, 0.5954649390243902, 0.0, 0.0, 0.0, 0.0, 0.0, 0.0, 0.0, 0.2977324695121951, 1.4886623475609757, 0.0, 0.0, 0.0, 0.0, 0.0, 2.0841272865853657, 0.0, 0.8931974085365854, 0.0, 0.0, 2.679592225609756, 0.8931974085365854, 0.2977324695121951, 0.2977324695121951, 0.0, 2.381859756097561, 0.5954649390243902, 0.2977324695121951, 0.0, 0.0, 0.2977324695121951, 0.0, 0.0, 0.0, 0.0], [0.0, 3.2750571646341466, 0.0, 0.2977324695121951, 0.2977324695121951, 0.0, 0.2977324695121951, 0.0, 0.2977324695121951, 0.0, 0.0, 0.0, 0.0, 0.2977324695121951, 0.0, 0.5954649390243902, 0.0, 0.5954649390243902, 0.0, 2.0841272865853657, 1.1909298780487805, 0.2977324695121951, 0.8931974085365854, 0.0, 0.2977324695121951, 0.0, 0.0, 0.0, 0.0, 0.0, 0.0, 0.0, 0.2977324695121951, 0.0, 0.2977324695121951, 1.4886623475609757, 0.0, 0.0, 1.1909298780487805, 0.2977324695121951, 0.2977324695121951, 0.0, 0.0, 0.0, 0.0, 0.0, 0.2977324695121951, 2.679592225609756, 0.0, 0.8931974085365854], [1.1909298780487805, 0.0, 0.0, 0.8931974085365854, 0.5954649390243902, 0.2977324695121951, 0.0, 0.0, 0.0, 0.2977324695121951, 0.2977324695121951, 0.0, 0.2977324695121951, 0.8931974085365854, 0.2977324695121951, 0.0, 0.2977324695121951, 0.5954649390243902, 0.0, 0.0, 0.0, 0.2977324695121951, 0.2977324695121951, 0.2977324695121951, 0.2977324695121951, 0.0, 0.2977324695121951, 0.2977324695121951, 0.0, 0.0, 0.0, 0.0, 0.2977324695121951, 0.2977324695121951, 0.0, 5.656916920731708, 0.2977324695121951, 0.8931974085365854, 0.2977324695121951, 0.5954649390243902, 0.2977324695121951, 4.1682545731707314, 3.5727896341463414, 7.741044207317073, 0.2977324695121951, 0.2977324695121951, 0.2977324695121951, 0.0, 0.0, 0.0], [0.0, 0.5954649390243902, 0.5954649390243902, 0.0, 0.0, 0.0, 1.7863948170731707, 0.8931974085365854, 0.0, 0.2977324695121951, 0.8931974085365854, 2.9773246951219514, 0.0, 0.2977324695121951, 1.4886623475609757, 0.0, 0.0, 0.0, 0.0, 0.2977324695121951, 0.2977324695121951, 0.0, 0.0, 0.5954649390243902, 0.2977324695121951, 0.5954649390243902, 0.5954649390243902, 2.9773246951219514, 2.381859756097561, 0.0, 0.8931974085365854, 0.8931974085365854, 0.5954649390243902, 0.2977324695121951, 0.0, 0.0, 2.381859756097561, 0.2977324695121951, 0.0, 1.1909298780487805, 0.0, 1.1909298780487805, 0.8931974085365854, 0.0, 0.5954649390243902, 0.8931974085365854, 0.2977324695121951, 8.931974085365853, 0.0, 0.0], [0.2977324695121951, 0.2977324695121951, 0.2977324695121951, 0.2977324695121951, 0.2977324695121951, 0.5954649390243902, 0.2977324695121951, 2.381859756097561, 0.5954649390243902, 1.1909298780487805, 0.0, 0.0, 0.0, 0.0, 0.0, 0.0, 0.8931974085365854, 0.0, 0.2977324695121951, 0.2977324695121951, 0.8931974085365854, 0.0, 0.0, 0.0, 0.2977324695121951, 0.0, 0.2977324695121951, 0.2977324695121951, 0.0, 0.0, 0.0, 0.8931974085365854, 0.0, 0.0, 0.0, 0.0, 0.0, 0.5954649390243902, 0.2977324695121951, 0.5954649390243902, 1.7863948170731707, 0.5954649390243902, 0.0, 0.0, 0.0, 1.7863948170731707, 0.0, 0.0, 0.0, 0.0], [0.0, 0.0, 0.0, 0.0, 0.0, 0.2977324695121951, 0.2977324695121951, 0.2977324695121951, 0.0, 0.0, 0.0, 0.2977324695121951, 0.0, 0.2977324695121951, 0.2977324695121951, 0.2977324695121951, 0.0, 0.5954649390243902, 0.0, 0.2977324695121951, 0.0, 0.8931974085365854, 0.8931974085365854, 0.2977324695121951, 0.2977324695121951, 0.0, 0.2977324695121951, 0.2977324695121951, 0.0, 0.2977324695121951, 2.0841272865853657, 4.1682545731707314, 0.0, 0.2977324695121951, 0.8931974085365854, 0.0, 0.8931974085365854, 0.0, 3.2750571646341466, 0.2977324695121951, 0.2977324695121951, 0.0, 0.8931974085365854, 1.1909298780487805, 0.2977324695121951, 0.5954649390243902, 0.8931974085365854, 0.2977324695121951, 0.0, 0.2977324695121951], [0.0, 0.2977324695121951, 0.0, 0.2977324695121951, 0.5954649390243902, 0.5954649390243902, 0.2977324695121951, 0.5954649390243902, 0.0, 0.5954649390243902, 0.0, 0.0, 0.0, 0.2977324695121951, 0.0, 0.5954649390243902, 0.2977324695121951, 0.2977324695121951, 2.0841272865853657, 0.2977324695121951, 0.0, 0.0, 0.0, 0.0, 0.0, 0.2977324695121951, 0.5954649390243902, 0.0, 1.4886623475609757, 1.1909298780487805, 0.5954649390243902, 0.0, 0.2977324695121951, 0.2977324695121951, 1.1909298780487805, 0.2977324695121951, 0.2977324695121951, 0.2977324695121951, 0.2977324695121951, 0.5954649390243902, 1.1909298780487805, 0.2977324695121951, 0.0, 0.2977324695121951, 4.1682545731707314, 0.2977324695121951, 0.2977324695121951, 0.8931974085365854, 0.0, 0.0], [0.0, 0.0, 0.2977324695121951, 0.0, 0.0, 0.0, 3.8705221036585367, 0.0, 0.0, 0.0, 1.1909298780487805, 0.5954649390243902, 0.2977324695121951, 0.0, 0.8931974085365854, 0.0, 1.1909298780487805, 0.0, 0.2977324695121951, 0.0, 0.0, 1.4886623475609757, 0.0, 0.0, 0.0, 0.0, 0.0, 0.2977324695121951, 2.0841272865853657, 0.0, 0.0, 0.2977324695121951, 0.2977324695121951, 0.2977324695121951, 0.0, 2.0841272865853657, 0.2977324695121951, 0.2977324695121951, 0.8931974085365854, 0.5954649390243902, 0.8931974085365854, 3.8705221036585367, 0.0, 1.7863948170731707, 2.679592225609756, 0.2977324695121951, 0.2977324695121951, 0.8931974085365854, 0.0, 0.2977324695121951], [0.2977324695121951, 0.2977324695121951, 0.2977324695121951, 1.1909298780487805, 0.0, 1.4886623475609757, 0.0, 0.2977324695121951, 1.1909298780487805, 0.0, 1.1909298780487805, 3.2750571646341466, 0.0, 0.2977324695121951, 2.679592225609756, 0.5954649390243902, 0.0, 0.2977324695121951, 0.2977324695121951, 0.0, 0.8931974085365854, 0.0, 0.0, 0.0, 0.2977324695121951, 0.2977324695121951, 0.2977324695121951, 0.2977324695121951, 0.0, 0.0, 0.2977324695121951, 0.5954649390243902, 0.0, 0.2977324695121951, 0.0, 0.0, 0.0, 0.0, 1.4886623475609757, 0.2977324695121951, 0.0, 0.0, 2.9773246951219514, 0.5954649390243902, 1.4886623475609757, 3.2750571646341466, 1.1909298780487805, 0.0, 0.5954649390243902, 0.2977324695121951], [0.2977324695121951, 0.2977324695121951, 0.0, 0.0, 0.2977324695121951, 0.0, 0.2977324695121951, 0.5954649390243902, 0.2977324695121951, 0.2977324695121951, 0.5954649390243902, 0.2977324695121951, 0.0, 0.2977324695121951, 5.359184451219512, 0.0, 0.0, 0.2977324695121951, 0.0, 0.8931974085365854, 0.2977324695121951, 0.2977324695121951, 0.0, 0.0, 0.0, 2.381859756097561, 0.2977324695121951, 0.0, 0.0, 0.0, 0.2977324695121951, 0.5954649390243902, 0.5954649390243902, 0.0, 0.0, 0.2977324695121951, 0.5954649390243902, 0.0, 0.0, 0.0, 0.5954649390243902, 0.5954649390243902, 0.0, 0.2977324695121951, 0.2977324695121951, 0.8931974085365854, 0.2977324695121951, 0.5954649390243902, 3.5727896341463414, 0.8931974085365854], [0.0, 0.0, 0.0, 0.5954649390243902, 0.0, 0.2977324695121951, 0.2977324695121951, 0.0, 0.2977324695121951, 0.0, 0.0, 1.1909298780487805, 0.0, 0.0, 0.0, 0.8931974085365854, 0.0, 0.0, 0.2977324695121951, 0.0, 0.0, 0.2977324695121951, 0.0, 0.2977324695121951, 0.0, 0.0, 0.2977324695121951, 0.0, 0.5954649390243902, 0.2977324695121951, 0.0, 0.2977324695121951, 1.4886623475609757, 0.0, 2.9773246951219514, 0.2977324695121951, 0.5954649390243902, 0.0, 0.0, 0.0, 0.8931974085365854, 0.2977324695121951, 0.0, 1.4886623475609757, 1.4886623475609757, 0.0, 0.2977324695121951, 0.0, 0.2977324695121951, 0.5954649390243902], [0.0, 0.0, 0.2977324695121951, 2.0841272865853657, 1.1909298780487805, 0.2977324695121951, 1.1909298780487805, 0.0, 0.0, 0.2977324695121951, 0.2977324695121951, 1.1909298780487805, 0.5954649390243902, 0.2977324695121951, 0.8931974085365854, 0.2977324695121951, 0.0, 0.0, 0.0, 0.0, 0.5954649390243902, 0.0, 0.2977324695121951, 0.2977324695121951, 0.2977324695121951, 0.0, 0.8931974085365854, 0.2977324695121951, 0.0, 0.2977324695121951, 0.2977324695121951, 1.4886623475609757, 0.0, 0.5954649390243902, 0.2977324695121951, 0.2977324695121951, 0.0, 0.0, 1.1909298780487805, 3.8705221036585367, 0.0, 0.5954649390243902, 0.0, 0.0, 0.5954649390243902, 0.2977324695121951, 0.2977324695121951, 0.0, 0.0, 0.2977324695121951]]
  in  "right":bool
  in  "left":bool
  in  "up":bool
  in  "down":bool
  in  "center":bool
  in  "zero1":bool
  in  "zero2":bool
  in  "MoveStageTarget 2":bool
  in  "Target position mm 2":dbl=78.45775 step=0.025 format="%_6g"
  in  "Target position mm 3":dbl=77.0 step=0.025 format="%_6g"
  in  "MoveStageTarget 3":bool
  in  "min2":dbl caption="min1" format="%#.0f"
  in  "max2":dbl=250.0 caption="max" step=250.0 format="%#.0f"
  in  "max3":dbl=500.0 caption="max" min=0.0 step=250.0 format="%#.0f"
  in  "min3":dbl=283.1435785060976 caption="min1" format="%#.0f"
  in  "autoscale3":bool
  in  "autoscale2":bool
  in  "Stage Acquire Parameters":T2={"Scan Mode"=enum."None", "Start position mm"=79.5, "End position mm"=83.0, "Velocity um/sec (continuous)"=100.0, "Step size microns (discrete)"=100.0, "Frames to grab (grab)"=1} {"Frames to grab (grab)" min=1 step=1; "Velocity um/sec (continuous)" min=0.1 max=10000.0 step=1.0 format="%.1f"; "End position mm" min=0.0 max=220.0 step=0.1 format="%_6g"; "Start position mm" min=0.0 max=220.0 step=0.1 format="%_6g"; "Step size microns (discrete)" min=0.1 max=1000.0 step=1.0 format="%.1f"}
  in  "Velocity mm/s":sgl=5.0 min=0.01 max=10 step=0.1
  in  "Save Path":path=path "C:/Users/Trent/Documents/Jeremy"
  out "CH3":dbl[][](graph)=[[399.854706554878, 357.8744283536585, 360.8517530487805, 356.3857660060976, 398.06831173780483, 372.7610518292683, 358.4698932926829, 373.0587842987805, 353.1107088414634, 352.51524390243907, 342.3923399390244, 355.49256859756093, 352.51524390243907, 362.9358803353659, 383.7771532012195, 357.2789634146341, 327.8034489329268, 350.1333841463415, 349.24018673780483, 322.7419969512195, 347.4537919207317, 331.07850609756093, 372.4633193597561, 331.9717035060976, 392.11366234756093, 367.4018673780488, 350.1333841463415, 316.4896150914634, 368.8905297256098, 349.5379192073171, 324.5283917682927, 394.4955221036585, 357.8744283536585, 366.5086699695122, 347.4537919207317, 367.9973323170732, 351.026581554878, 363.233612804878, 373.3565167682927, 363.8290777439024, 370.0814596036585, 348.3469893292683, 364.1268102134146, 359.9585556402439, 372.7610518292683, 384.9680830792683, 354.8971036585366, 388.5408727134146, 364.1268102134146, 384.6703506097561], [400.7479039634147, 356.0880335365854, 356.0880335365854, 382.5862233231707, 381.6930259146341, 372.4633193597561, 377.2270388719512, 370.97465701219517, 338.2240853658537, 362.9358803353659, 372.1655868902439, 360.2562881097561, 338.2240853658537, 376.6315739329268, 349.24018673780483, 356.981230945122, 368.8905297256098, 369.4859946646341, 353.1107088414634, 373.9519817073171, 340.30821265243907, 349.5379192073171, 340.30821265243907, 342.6900724085366, 346.8583269817073, 350.4311166158537, 367.4018673780488, 331.3762385670732, 347.1560594512195, 352.2175114329268, 364.4245426829268, 348.0492568597561, 321.5510670731707, 329.58984375, 346.8583269817073, 366.2109375, 355.1948361280488, 371.5701219512195, 374.2497141768293, 337.03315548780483, 357.2789634146341, 373.3565167682927, 367.1041349085366, 393.3045922256098, 388.8386051829268, 368.5927972560976, 376.92930640243907, 373.3565167682927, 368.5927972560976, 384.6703506097561], [379.3111661585366, 381.395293445122, 384.6703506097561, 365.0200076219512, 351.3243140243902, 334.9490282012195, 364.72227515243907, 365.9132050304878, 372.4633193597561, 339.1172827743902, 372.4633193597561, 338.2240853658537, 322.7419969512195, 359.0653582317073, 333.7580983231707, 337.03315548780483, 323.0397294207317, 340.6059451219512, 339.4150152439024, 342.0946074695122, 323.6351943597561, 370.3791920731707, 326.3147865853659, 325.1238567073171, 363.8290777439024, 371.8678544207317, 359.6608231707317, 307.5576410060976, 374.5474466463415, 351.3243140243902, 346.56059451219517, 335.5444931402439, 376.0361089939024, 381.9907583841463, 363.8290777439024, 314.1077553353659, 362.3404153963415, 344.4764672256098, 369.4859946646341, 359.6608231707317, 375.440644054878, 380.5020960365854, 381.9907583841463, 372.7610518292683, 358.4698932926829, 379.3111661585366, 362.3404153963415, 368.2950647865854, 410.57307545731703, 365.0200076219512], [353.4084413109756, 376.6315739329268, 372.4633193597561, 373.3565167682927, 311.4281631097561, 355.49256859756093, 352.51524390243907, 351.026581554878, 387.3499428353659, 365.0200076219512, 347.1560594512195, 340.6059451219512, 318.87147484756093, 359.3630907012195, 370.6769245426829, 345.9651295731707, 335.5444931402439, 327.5057164634146, 352.8129763719512, 326.612519054878, 325.7193216463415, 340.30821265243907, 356.981230945122, 344.1787347560976, 327.2079839939024, 310.8326981707317, 324.2306592987805, 342.9878048780488, 359.0653582317073, 349.24018673780483, 331.07850609756093, 360.8517530487805, 368.2950647865854, 358.4698932926829, 336.7354230182927, 368.5927972560976, 352.8129763719512, 371.8678544207317, 379.0134336890244, 358.76762576219517, 379.6088986280488, 354.5993711890244, 357.2789634146341, 370.3791920731707, 379.6088986280488, 380.7998285060976, 380.2043635670732, 343.8810022865854, 358.1721608231707, 376.92930640243907], [384.0748856707317, 350.1333841463415, 346.2628620426829, 372.7610518292683, 356.981230945122, 354.3016387195122, 354.00390625, 394.4955221036585, 350.4311166158537, 339.1172827743902, 348.3469893292683, 347.1560594512195, 352.2175114329268, 367.4018673780488, 354.3016387195122, 357.2789634146341, 328.9943788109756, 341.4991425304878, 328.3989138719512, 326.3147865853659, 346.56059451219517, 343.28553734756093, 313.8100228658537, 318.2760099085366, 329.58984375, 359.0653582317073, 317.6805449695122, 363.8290777439024, 347.1560594512195, 360.2562881097561, 368.2950647865854, 320.360137195122, 368.2950647865854, 330.4830411585366, 355.7903010670732, 311.1304306402439, 356.0880335365854, 359.6608231707317, 382.2884908536585, 329.58984375, 379.3111661585366, 340.9036775914634, 336.4376905487805, 381.395293445122, 399.2592416158537, 356.0880335365854, 346.8583269817073, 357.5766958841463, 378.7157012195122, 358.1721608231707], [373.0587842987805, 365.3177400914634, 355.7903010670732, 373.0587842987805, 347.7515243902439, 394.1977896341463, 347.4537919207317, 364.1268102134146, 321.8487995426829, 362.3404153963415, 322.7419969512195, 339.1172827743902, 354.3016387195122, 319.1692073170732, 294.45741234756093, 343.8810022865854, 351.3243140243902, 319.1692073170732, 335.2467606707317, 333.7580983231707, 357.2789634146341, 362.9358803353659, 319.4669397865854, 327.2079839939024, 327.8034489329268, 348.9424542682927, 305.7712461890244, 329.2921112804878, 330.7807736280488, 340.0104801829268, 359.0653582317073, 357.5766958841463, 338.819550304878, 349.24018673780483, 336.1399580792683, 354.3016387195122, 358.1721608231707, 330.7807736280488, 356.6834984756098, 376.6315739329268, 354.3016387195122, 354.5993711890244, 396.8773818597561, 365.3177400914634, 343.28553734756093, 353.4084413109756, 407.00028582317077, 379.0134336890244, 372.4633193597561, 347.4537919207317], [379.3111661585366, 351.026581554878, 341.2014100609756, 346.56059451219517, 359.3630907012195, 375.7383765243902, 357.2789634146341, 356.6834984756098, 358.76762576219517, 350.7288490853659, 367.4018673780488, 347.1560594512195, 326.3147865853659, 355.1948361280488, 304.5803163109756, 338.819550304878, 322.7419969512195, 373.9519817073171, 299.5188643292683, 350.1333841463415, 361.44721798780483, 342.6900724085366, 321.8487995426829, 348.6447217987805, 311.1304306402439, 331.9717035060976, 360.8517530487805, 327.8034489329268, 314.405487804878, 333.7580983231707, 342.9878048780488, 348.0492568597561, 341.4991425304878, 362.3404153963415, 324.82612423780483, 347.7515243902439, 338.5218178353659, 349.8356516768293, 356.981230945122, 327.2079839939024, 391.5181974085366, 349.5379192073171, 371.8678544207317, 388.2431402439024, 345.6673971036585, 367.69959984756093, 365.0200076219512, 379.0134336890244, 371.5701219512195, 378.41796875], [388.2431402439024, 372.1655868902439, 324.5283917682927, 373.0587842987805, 334.35356326219517, 363.5313452743902, 323.9329268292683, 351.6220464939024, 316.7873475609756, 363.8290777439024, 301.0075266768293, 351.026581554878, 356.0880335365854, 337.9263528963415, 372.4633193597561, 323.6351943597561, 328.9943788109756, 342.3923399390244, 320.0624047256098, 333.7580983231707, 340.9036775914634, 336.1399580792683, 318.5737423780488, 366.5086699695122, 297.73246951219517, 308.4508384146341, 329.8875762195122, 347.4537919207317, 334.0558307926829, 348.0492568597561, 300.1143292682927, 322.14653201219517, 338.5218178353659, 372.4633193597561, 381.395293445122, 330.1853086890244, 314.7032202743902, 373.65424923780483, 362.3404153963415, 364.1268102134146, 392.11366234756093, 341.4991425304878, 342.6900724085366, 369.4859946646341, 373.65424923780483, 337.03315548780483, 362.6381478658537, 376.3338414634146, 398.06831173780483, 335.2467606707317], [358.1721608231707, 382.2884908536585, 377.2270388719512, 370.6769245426829, 314.1077553353659, 365.6154725609756, 347.7515243902439, 363.8290777439024, 341.4991425304878, 367.4018673780488, 342.6900724085366, 349.8356516768293, 332.8649009146341, 315.5964176829268, 335.2467606707317, 334.6512957317073, 351.6220464939024, 337.3308879573171, 370.0814596036585, 348.0492568597561, 326.9102515243902, 344.4764672256098, 326.0170541158537, 352.2175114329268, 314.405487804878, 337.3308879573171, 350.1333841463415, 358.1721608231707, 338.2240853658537, 328.6966463414634, 370.3791920731707, 352.51524390243907, 311.7258955792683, 312.9168254573171, 328.10118140243907, 349.5379192073171, 336.1399580792683, 361.1494855182927, 396.2819169207317, 367.69959984756093, 354.8971036585366, 357.5766958841463, 362.3404153963415, 346.2628620426829, 353.1107088414634, 392.7091272865854, 299.5188643292683, 357.5766958841463, 343.8810022865854, 379.3111661585366], [393.0068597560976, 347.4537919207317, 375.1429115853659, 345.9651295731707, 362.6381478658537, 350.7288490853659, 374.8451791158537, 314.405487804878, 330.4830411585366, 314.405487804878, 326.612519054878, 333.4603658536585, 312.9168254573171, 339.1172827743902, 365.0200076219512, 284.9299733231707, 317.9782774390244, 308.153105945122, 315.89415015243907, 322.4442644817073, 344.774199695122, 318.87147484756093, 319.4669397865854, 294.7551448170732, 343.8810022865854, 366.2109375, 368.5927972560976, 326.9102515243902, 335.8422256097561, 326.0170541158537, 340.30821265243907, 342.0946074695122, 355.1948361280488, 348.3469893292683, 332.567168445122, 329.58984375, 340.9036775914634, 320.6578696646341, 324.5283917682927, 373.0587842987805, 360.8517530487805, 358.4698932926829, 358.4698932926829, 326.9102515243902, 391.2204649390244, 371.8678544207317, 368.8905297256098, 345.6673971036585, 338.5218178353659, 375.440644054878], [360.8517530487805, 369.7837271341463, 348.3469893292683, 333.1626333841463, 343.8810022865854, 361.44721798780483, 356.6834984756098, 333.1626333841463, 354.00390625, 334.6512957317073, 324.82612423780483, 330.1853086890244, 335.8422256097561, 319.1692073170732, 315.89415015243907, 339.1172827743902, 319.1692073170732, 316.1918826219512, 333.1626333841463, 311.4281631097561, 298.9233993902439, 354.5993711890244, 312.9168254573171, 315.2986852134146, 315.2986852134146, 299.5188643292683, 303.68711890243907, 325.7193216463415, 320.6578696646341, 339.4150152439024, 326.3147865853659, 330.4830411585366, 308.153105945122, 325.1238567073171, 355.7903010670732, 326.612519054878, 341.2014100609756, 327.2079839939024, 334.9490282012195, 377.8225038109756, 325.7193216463415, 366.5086699695122, 341.4991425304878, 354.3016387195122, 334.35356326219517, 357.5766958841463, 326.0170541158537, 376.3338414634146, 334.9490282012195, 379.90663109756093], [377.2270388719512, 307.2599085365854, 339.1172827743902, 353.7061737804878, 358.1721608231707, 330.7807736280488, 315.0009527439024, 302.198456554878, 313.8100228658537, 329.8875762195122, 327.5057164634146, 305.17578125, 328.9943788109756, 346.56059451219517, 357.2789634146341, 333.4603658536585, 341.2014100609756, 277.1889291158537, 304.5803163109756, 298.6256669207317, 303.3893864329268, 311.4281631097561, 342.9878048780488, 331.3762385670732, 297.4347370426829, 319.4669397865854, 310.8326981707317, 315.0009527439024, 291.48008765243907, 317.3828125, 321.8487995426829, 342.6900724085366, 305.17578125, 315.2986852134146, 315.5964176829268, 330.7807736280488, 318.87147484756093, 356.981230945122, 328.6966463414634, 346.8583269817073, 345.9651295731707, 336.1399580792683, 361.7449504573171, 356.3857660060976, 356.3857660060976, 371.5701219512195, 334.9490282012195, 323.0397294207317, 345.9651295731707, 351.026581554878], [367.4018673780488, 366.5086699695122, 338.819550304878, 373.3565167682927, 359.9585556402439, 322.7419969512195, 308.4508384146341, 359.0653582317073, 340.9036775914634, 335.8422256097561, 337.6286204268293, 294.45741234756093, 340.30821265243907, 303.0916539634146, 309.6417682926829, 333.1626333841463, 336.1399580792683, 302.7939214939024, 345.3696646341463, 306.9621760670732, 340.6059451219512, 316.7873475609756, 298.6256669207317, 294.1596798780488, 310.8326981707317, 289.991425304878, 315.89415015243907, 303.0916539634146, 332.8649009146341, 325.7193216463415, 362.6381478658537, 354.5993711890244, 317.0850800304878, 345.6673971036585, 348.9424542682927, 348.9424542682927, 337.6286204268293, 341.4991425304878, 328.6966463414634, 305.7712461890244, 354.00390625, 362.6381478658537, 340.9036775914634, 354.3016387195122, 357.8744283536585, 335.5444931402439, 374.2497141768293, 377.2270388719512, 375.1429115853659, 334.9490282012195], [387.647675304878, 349.24018673780483, 375.7383765243902, 353.4084413109756, 348.6447217987805, 358.1721608231707, 346.56059451219517, 330.4830411585366, 312.9168254573171, 305.17578125, 333.4603658536585, 345.0719321646341, 304.5803163109756, 278.6775914634146, 317.6805449695122, 347.7515243902439, 338.5218178353659, 301.6029916158537, 285.52543826219517, 322.4442644817073, 286.1209032012195, 329.58984375, 293.5642149390244, 311.7258955792683, 288.20503048780483, 322.4442644817073, 317.6805449695122, 319.1692073170732, 293.8619474085366, 297.1370045731707, 326.612519054878, 309.93950076219517, 341.4991425304878, 333.7580983231707, 325.1238567073171, 337.6286204268293, 308.4508384146341, 279.5707888719512, 348.6447217987805, 296.8392721036585, 334.35356326219517, 312.61909298780483, 338.5218178353659, 361.1494855182927, 343.28553734756093, 396.5796493902439, 381.6930259146341, 351.026581554878, 367.69959984756093, 352.2175114329268], [342.6900724085366, 363.5313452743902, 354.5993711890244, 373.0587842987805, 318.5737423780488, 344.1787347560976, 348.3469893292683, 292.96875, 323.6351943597561, 324.5283917682927, 343.5832698170732, 301.0075266768293, 321.5510670731707, 324.82612423780483, 329.2921112804878, 303.68711890243907, 271.8297446646341, 298.6256669207317, 291.48008765243907, 282.8458460365854, 327.8034489329268, 302.4961890243902, 287.6095655487805, 339.7127477134146, 258.7295160060976, 341.2014100609756, 324.82612423780483, 283.4413109756098, 313.5122903963415, 339.1172827743902, 337.3308879573171, 310.2372332317073, 334.35356326219517, 316.1918826219512, 301.6029916158537, 288.5027629573171, 312.61909298780483, 312.9168254573171, 324.2306592987805, 356.3857660060976, 315.5964176829268, 330.1853086890244, 362.9358803353659, 329.2921112804878, 303.3893864329268, 359.6608231707317, 349.24018673780483, 367.9973323170732, 342.9878048780488, 353.7061737804878], [373.0587842987805, 351.6220464939024, 343.5832698170732, 328.10118140243907, 296.2438071646341, 329.8875762195122, 311.7258955792683, 325.4215891768293, 296.5415396341463, 347.7515243902439, 302.198456554878, 322.4442644817073, 309.0463033536585, 275.7002667682927, 305.4735137195122, 265.577362804878, 313.5122903963415, 279.27305640243907, 284.0367759146341, 264.6841653963415, 287.6095655487805, 298.6256669207317, 326.0170541158537, 317.0850800304878, 303.9848513719512, 335.2467606707317, 322.14653201219517, 317.3828125, 292.0755525914634, 311.4281631097561, 287.9072980182927, 328.9943788109756, 339.4150152439024, 350.1333841463415, 349.24018673780483, 347.7515243902439, 343.8810022865854, 356.6834984756098, 298.6256669207317, 347.4537919207317, 348.3469893292683, 321.8487995426829, 309.0463033536585, 347.7515243902439, 305.17578125, 367.1041349085366, 365.0200076219512, 352.51524390243907, 342.9878048780488, 348.0492568597561], [353.4084413109756, 294.7551448170732, 364.1268102134146, 326.0170541158537, 341.2014100609756, 288.20503048780483, 311.1304306402439, 345.3696646341463, 349.8356516768293, 320.0624047256098, 304.2825838414634, 309.6417682926829, 316.1918826219512, 335.5444931402439, 318.2760099085366, 345.6673971036585, 290.2891577743902, 304.8780487804878, 321.8487995426829, 294.7551448170732, 325.7193216463415, 321.5510670731707, 309.3440358231707, 336.1399580792683, 330.4830411585366, 285.52543826219517, 317.0850800304878, 248.90434451219514, 325.1238567073171, 339.7127477134146, 307.2599085365854, 315.89415015243907, 313.5122903963415, 307.8553734756098, 323.3374618902439, 298.3279344512195, 301.3052591463415, 301.3052591463415, 319.1692073170732, 315.89415015243907, 332.8649009146341, 347.7515243902439, 331.9717035060976, 352.51524390243907, 342.6900724085366, 358.4698932926829, 334.6512957317073, 374.8451791158537, 352.2175114329268, 326.612519054878], [339.4150152439024, 311.1304306402439, 323.9329268292683, 342.6900724085366, 333.4603658536585, 301.6029916158537, 315.89415015243907, 315.5964176829268, 272.4252096036585, 358.1721608231707, 307.2599085365854, 322.14653201219517, 312.61909298780483, 313.8100228658537, 299.8165967987805, 294.45741234756093, 293.5642149390244, 296.2438071646341, 335.5444931402439, 304.8780487804878, 326.612519054878, 297.1370045731707, 273.31840701219517, 323.9329268292683, 282.5481135670732, 287.3118330792683, 297.1370045731707, 311.7258955792683, 290.8846227134146, 317.3828125, 281.9526486280488, 330.7807736280488, 300.7097942073171, 298.9233993902439, 317.9782774390244, 326.9102515243902, 288.8004954268293, 333.7580983231707, 328.6966463414634, 309.3440358231707, 356.0880335365854, 363.5313452743902, 288.8004954268293, 341.2014100609756, 344.774199695122, 318.5737423780488, 370.97465701219517, 337.03315548780483, 389.4340701219512, 343.28553734756093], [356.6834984756098, 350.4311166158537, 336.4376905487805, 300.41206173780483, 322.14653201219517, 318.2760099085366, 325.1238567073171, 317.3828125, 297.1370045731707, 331.6739710365854, 319.4669397865854, 282.8458460365854, 310.5349657012195, 307.8553734756098, 345.0719321646341, 300.41206173780483, 338.5218178353659, 318.5737423780488, 309.0463033536585, 287.0141006097561, 300.7097942073171, 275.4025342987805, 298.0302019817073, 265.2796303353659, 307.5576410060976, 304.8780487804878, 306.9621760670732, 307.5576410060976, 261.11137576219517, 322.14653201219517, 275.7002667682927, 353.1107088414634, 326.612519054878, 281.0594512195122, 291.7778201219512, 334.0558307926829, 302.198456554878, 259.324980945122, 309.93950076219517, 329.8875762195122, 300.7097942073171, 312.61909298780483, 328.10118140243907, 362.6381478658537, 311.7258955792683, 330.7807736280488, 358.4698932926829, 353.7061737804878, 328.6966463414634, 349.5379192073171], [364.4245426829268, 301.6029916158537, 311.4281631097561, 302.198456554878, 351.9197789634146, 315.89415015243907, 325.7193216463415, 280.4639862804878, 310.8326981707317, 323.3374618902439, 327.8034489329268, 283.739043445122, 315.2986852134146, 314.7032202743902, 294.45741234756093, 290.8846227134146, 309.93950076219517, 310.2372332317073, 303.0916539634146, 311.7258955792683, 277.784394054878, 278.9753239329268, 287.9072980182927, 304.2825838414634, 306.66444359756093, 315.0009527439024, 302.4961890243902, 302.4961890243902, 322.4442644817073, 313.2145579268293, 305.4735137195122, 281.6549161585366, 299.8165967987805, 294.1596798780488, 321.8487995426829, 321.5510670731707, 276.5934641768293, 331.9717035060976, 305.7712461890244, 332.8649009146341, 347.4537919207317, 348.3469893292683, 348.9424542682927, 323.3374618902439, 320.6578696646341, 327.5057164634146, 313.2145579268293, 343.5832698170732, 331.07850609756093, 364.4245426829268], [326.9102515243902, 321.8487995426829, 295.3506097560976, 303.0916539634146, 333.1626333841463, 338.2240853658537, 292.0755525914634, 311.4281631097561, 283.739043445122, 295.6483422256098, 281.9526486280488, 318.5737423780488, 354.8971036585366, 271.8297446646341, 307.5576410060976, 278.0821265243902, 276.5934641768293, 297.73246951219517, 314.7032202743902, 289.991425304878, 309.6417682926829, 299.5188643292683, 280.4639862804878, 275.7002667682927, 304.5803163109756, 259.9204458841463, 297.4347370426829, 290.2891577743902, 334.6512957317073, 295.6483422256098, 336.7354230182927, 287.0141006097561, 348.0492568597561, 292.96875, 296.2438071646341, 348.3469893292683, 304.5803163109756, 336.7354230182927, 309.6417682926829, 335.5444931402439, 250.98847179878047, 315.2986852134146, 330.4830411585366, 326.3147865853659, 332.2694359756098, 326.3147865853659, 362.6381478658537, 346.8583269817073, 350.1333841463415, 349.5379192073171], [358.1721608231707, 346.56059451219517, 327.2079839939024, 356.6834984756098, 326.612519054878, 344.1787347560976, 308.7485708841463, 333.1626333841463, 279.27305640243907, 308.4508384146341, 267.6614900914634, 320.6578696646341, 281.9526486280488, 296.8392721036585, 326.612519054878, 290.2891577743902, 283.739043445122, 285.52543826219517, 261.11137576219517, 298.6256669207317, 285.2277057926829, 288.5027629573171, 300.41206173780483, 303.0916539634146, 285.8231707317073, 305.17578125, 272.7229420731707, 269.7456173780488, 261.4091082317073, 271.2342797256098, 318.2760099085366, 292.6710175304878, 319.7646722560976, 310.8326981707317, 292.6710175304878, 309.6417682926829, 304.2825838414634, 288.5027629573171, 306.9621760670732, 312.0236280487805, 303.3893864329268, 331.07850609756093, 337.9263528963415, 325.4215891768293, 325.7193216463415, 369.4859946646341, 342.6900724085366, 351.6220464939024, 286.1209032012195, 327.2079839939024], [362.9358803353659, 307.5576410060976, 289.991425304878, 301.3052591463415, 309.93950076219517, 347.4537919207317, 297.1370045731707, 303.0916539634146, 270.3410823170732, 303.9848513719512, 289.991425304878, 312.9168254573171, 334.9490282012195, 277.1889291158537, 275.7002667682927, 302.198456554878, 278.6775914634146, 298.9233993902439, 251.28620426829266, 288.5027629573171, 272.4252096036585, 306.0689786585366, 275.99799923780483, 342.9878048780488, 270.04334984756093, 275.7002667682927, 259.6227134146341, 305.17578125, 294.45741234756093, 267.6614900914634, 253.07259908536585, 285.8231707317073, 311.7258955792683, 316.1918826219512, 313.2145579268293, 315.2986852134146, 304.8780487804878, 302.7939214939024, 308.7485708841463, 288.5027629573171, 345.3696646341463, 314.7032202743902, 294.45741234756093, 306.66444359756093, 325.7193216463415, 326.612519054878, 352.8129763719512, 337.3308879573171, 357.2789634146341, 326.0170541158537], [344.1787347560976, 279.5707888719512, 323.9329268292683, 312.3213605182927, 334.0558307926829, 306.66444359756093, 269.1501524390244, 334.0558307926829, 253.37033155487805, 310.8326981707317, 291.7778201219512, 264.9818978658537, 278.0821265243902, 277.4866615853659, 307.5576410060976, 289.3959603658537, 278.6775914634146, 304.2825838414634, 260.8136432926829, 241.16330030487805, 314.1077553353659, 284.0367759146341, 313.5122903963415, 307.2599085365854, 302.4961890243902, 274.2116044207317, 260.8136432926829, 328.3989138719512, 271.532012195122, 301.3052591463415, 297.73246951219517, 320.360137195122, 273.31840701219517, 309.3440358231707, 292.6710175304878, 296.2438071646341, 283.1435785060976, 320.0624047256098, 306.0689786585366, 278.3798589939024, 314.405487804878, 332.2694359756098, 331.6739710365854, 325.7193216463415, 330.4830411585366, 320.9556021341463, 330.4830411585366, 323.0397294207317, 335.8422256097561, 338.2240853658537], [342.3923399390244, 325.4215891768293, 299.2211318597561, 313.2145579268293, 298.6256669207317, 314.7032202743902, 266.7682926829268, 328.10118140243907, 281.6549161585366, 295.6483422256098, 330.7807736280488, 308.153105945122, 295.946074695122, 283.1435785060976, 291.1823551829268, 303.68711890243907, 298.3279344512195, 339.1172827743902, 298.6256669207317, 304.8780487804878, 262.8977705792683, 256.9431211890244, 316.1918826219512, 282.8458460365854, 287.3118330792683, 284.6322408536585, 289.991425304878, 295.946074695122, 299.5188643292683, 282.5481135670732, 271.8297446646341, 319.7646722560976, 283.4413109756098, 285.52543826219517, 341.2014100609756, 300.41206173780483, 297.73246951219517, 351.6220464939024, 320.0624047256098, 325.1238567073171, 300.1143292682927, 339.7127477134146, 292.3732850609756, 329.8875762195122, 322.7419969512195, 344.4764672256098, 339.4150152439024, 354.5993711890244, 322.14653201219517, 342.3923399390244], [327.8034489329268, 315.89415015243907, 300.1143292682927, 331.9717035060976, 306.3667111280488, 314.405487804878, 284.6322408536585, 273.0206745426829, 306.9621760670732, 275.4025342987805, 289.6936928353659, 297.1370045731707, 280.1662538109756, 285.52543826219517, 291.48008765243907, 282.8458460365854, 304.2825838414634, 311.1304306402439, 301.6029916158537, 278.9753239329268, 262.8977705792683, 289.3959603658537, 263.4932355182927, 223.8948170731707, 300.41206173780483, 297.1370045731707, 326.0170541158537, 310.8326981707317, 247.41568216463415, 292.96875, 261.11137576219517, 315.5964176829268, 233.12452362804876, 301.3052591463415, 301.3052591463415, 272.1274771341463, 314.7032202743902, 274.8070693597561, 287.0141006097561, 310.8326981707317, 289.0982278963415, 328.6966463414634, 274.2116044207317, 333.1626333841463, 351.3243140243902, 321.5510670731707, 301.3052591463415, 344.1787347560976, 334.0558307926829, 357.8744283536585], [325.7193216463415, 349.5379192073171, 275.1048018292683, 334.35356326219517, 298.6256669207317, 282.25038109756093, 280.4639862804878, 308.4508384146341, 307.8553734756098, 293.2664824695122, 287.3118330792683, 309.6417682926829, 265.2796303353659, 260.2181783536585, 258.4317835365854, 272.4252096036585, 310.5349657012195, 258.7295160060976, 295.946074695122, 284.9299733231707, 271.2342797256098, 301.0075266768293, 284.9299733231707, 278.0821265243902, 267.9592225609756, 312.0236280487805, 291.1823551829268, 273.6161394817073, 284.6322408536585, 286.7163681402439, 296.5415396341463, 309.93950076219517, 261.7068407012195, 274.8070693597561, 265.8750952743902, 297.73246951219517, 305.7712461890244, 285.52543826219517, 270.3410823170732, 337.9263528963415, 311.1304306402439, 311.4281631097561, 307.2599085365854, 289.6936928353659, 331.9717035060976, 312.61909298780483, 340.9036775914634, 320.0624047256098, 348.6447217987805, 321.8487995426829], [354.8971036585366, 318.5737423780488, 323.6351943597561, 312.61909298780483, 312.0236280487805, 282.25038109756093, 261.4091082317073, 287.0141006097561, 308.7485708841463, 267.3637576219512, 287.0141006097561, 269.7456173780488, 251.8816692073171, 302.4961890243902, 333.1626333841463, 265.2796303353659, 290.8846227134146, 270.9365472560976, 299.2211318597561, 310.5349657012195, 298.9233993902439, 319.4669397865854, 288.5027629573171, 315.2986852134146, 278.9753239329268, 315.2986852134146, 272.7229420731707, 243.8428925304878, 272.7229420731707, 305.7712461890244, 270.6388147865854, 264.6841653963415, 275.7002667682927, 282.8458460365854, 268.8524199695122, 294.45741234756093, 264.6841653963415, 303.3893864329268, 299.5188643292683, 317.6805449695122, 332.8649009146341, 346.2628620426829, 330.7807736280488, 322.7419969512195, 334.9490282012195, 310.2372332317073, 317.6805449695122, 337.3308879573171, 331.6739710365854, 316.4896150914634], [327.2079839939024, 285.2277057926829, 331.6739710365854, 312.3213605182927, 343.28553734756093, 313.5122903963415, 213.1764481707317, 261.7068407012195, 287.0141006097561, 277.4866615853659, 304.2825838414634, 257.5385861280488, 298.6256669207317, 256.0499237804878, 286.1209032012195, 277.1889291158537, 249.20207698170734, 270.3410823170732, 293.5642149390244, 270.6388147865854, 284.9299733231707, 277.1889291158537, 273.9138719512195, 313.5122903963415, 261.4091082317073, 270.04334984756093, 242.3542301829268, 266.1728277439024, 289.3959603658537, 260.5159108231707, 278.3798589939024, 309.0463033536585, 286.1209032012195, 323.6351943597561, 256.0499237804878, 280.76171875, 299.2211318597561, 320.6578696646341, 323.0397294207317, 344.4764672256098, 296.5415396341463, 316.1918826219512, 295.3506097560976, 296.5415396341463, 297.4347370426829, 339.1172827743902, 318.5737423780488, 344.1787347560976, 331.6739710365854, 339.7127477134146], [292.96875, 333.1626333841463, 298.0302019817073, 298.0302019817073, 296.2438071646341, 304.8780487804878, 270.3410823170732, 291.7778201219512, 280.4639862804878, 258.4317835365854, 281.6549161585366, 317.3828125, 272.7229420731707, 315.89415015243907, 314.7032202743902, 257.2408536585366, 270.9365472560976, 318.87147484756093, 277.784394054878, 306.66444359756093, 275.4025342987805, 273.6161394817073, 271.532012195122, 311.4281631097561, 279.5707888719512, 280.4639862804878, 292.3732850609756, 268.2569550304878, 255.15672637195124, 266.7682926829268, 272.4252096036585, 298.6256669207317, 303.68711890243907, 297.73246951219517, 312.61909298780483, 284.0367759146341, 263.79096798780483, 289.3959603658537, 319.1692073170732, 252.1794016768293, 287.9072980182927, 309.6417682926829, 349.24018673780483, 324.5283917682927, 344.4764672256098, 320.9556021341463, 321.8487995426829, 315.5964176829268, 298.6256669207317, 339.4150152439024], [317.3828125, 300.7097942073171, 264.9818978658537, 277.4866615853659, 296.2438071646341, 275.1048018292683, 288.5027629573171, 317.9782774390244, 299.5188643292683, 263.79096798780483, 247.71341463414635, 306.3667111280488, 301.6029916158537, 319.7646722560976, 252.1794016768293, 254.85899390243904, 262.8977705792683, 281.6549161585366, 258.4317835365854, 278.6775914634146, 281.6549161585366, 256.0499237804878, 229.84946646341461, 246.52248475609758, 279.27305640243907, 302.4961890243902, 248.6066120426829, 302.4961890243902, 280.1662538109756, 302.198456554878, 301.3052591463415, 281.3571836890244, 270.3410823170732, 304.5803163109756, 299.8165967987805, 299.5188643292683, 322.14653201219517, 293.2664824695122, 276.8911966463415, 308.7485708841463, 315.2986852134146, 278.3798589939024, 289.3959603658537, 312.0236280487805, 268.8524199695122, 304.5803163109756, 325.7193216463415, 304.5803163109756, 335.2467606707317, 372.1655868902439], [300.7097942073171, 266.1728277439024, 278.0821265243902, 291.7778201219512, 253.37033155487805, 284.9299733231707, 285.8231707317073, 279.5707888719512, 292.0755525914634, 260.8136432926829, 266.7682926829268, 260.2181783536585, 302.198456554878, 275.99799923780483, 269.7456173780488, 221.81068978658539, 292.96875, 295.3506097560976, 267.9592225609756, 250.3930068597561, 264.0887004573171, 297.73246951219517, 309.6417682926829, 270.9365472560976, 301.0075266768293, 244.4383574695122, 271.2342797256098, 247.71341463414635, 259.9204458841463, 279.27305640243907, 253.07259908536585, 281.6549161585366, 278.9753239329268, 283.1435785060976, 297.1370045731707, 310.8326981707317, 298.6256669207317, 308.7485708841463, 316.1918826219512, 289.991425304878, 317.9782774390244, 302.4961890243902, 337.6286204268293, 290.8846227134146, 312.9168254573171, 306.9621760670732, 303.3893864329268, 305.17578125, 357.5766958841463, 331.3762385670732], [298.3279344512195, 286.4186356707317, 270.6388147865854, 306.3667111280488, 318.87147484756093, 286.1209032012195, 309.93950076219517, 262.8977705792683, 282.5481135670732, 278.3798589939024, 256.9431211890244, 261.7068407012195, 290.8846227134146, 262.6000381097561, 259.6227134146341, 268.8524199695122, 256.0499237804878, 270.04334984756093, 283.1435785060976, 259.6227134146341, 268.5546875, 294.45741234756093, 298.0302019817073, 239.07917301829266, 231.04039634146343, 301.3052591463415, 272.7229420731707, 261.11137576219517, 263.79096798780483, 298.3279344512195, 298.6256669207317, 245.33155487804876, 302.4961890243902, 285.52543826219517, 270.3410823170732, 242.94969512195124, 255.45445884146343, 293.8619474085366, 273.0206745426829, 295.6483422256098, 264.0887004573171, 298.9233993902439, 305.4735137195122, 305.4735137195122, 291.7778201219512, 342.9878048780488, 295.6483422256098, 365.9132050304878, 334.0558307926829, 314.1077553353659], [293.5642149390244, 326.0170541158537, 285.8231707317073, 286.1209032012195, 285.8231707317073, 250.6907393292683, 305.4735137195122, 276.5934641768293, 281.6549161585366, 240.27010289634148, 304.8780487804878, 272.7229420731707, 278.3798589939024, 293.8619474085366, 234.31545350609758, 284.6322408536585, 258.1340510670732, 296.8392721036585, 245.62928734756096, 323.0397294207317, 239.6746379573171, 270.3410823170732, 329.58984375, 244.7360899390244, 260.8136432926829, 262.8977705792683, 262.0045731707317, 280.4639862804878, 257.5385861280488, 277.784394054878, 287.6095655487805, 252.77486661585365, 249.7975419207317, 257.5385861280488, 263.79096798780483, 345.6673971036585, 261.7068407012195, 296.8392721036585, 282.25038109756093, 275.4025342987805, 273.6161394817073, 289.6936928353659, 285.8231707317073, 303.68711890243907, 298.3279344512195, 362.9358803353659, 292.3732850609756, 337.03315548780483, 356.3857660060976, 316.7873475609756], [340.30821265243907, 283.739043445122, 284.9299733231707, 312.61909298780483, 255.45445884146343, 311.4281631097561, 314.1077553353659, 289.991425304878, 281.6549161585366, 310.8326981707317, 257.2408536585366, 278.0821265243902, 295.6483422256098, 294.1596798780488, 293.8619474085366, 287.9072980182927, 245.33155487804876, 289.6936928353659, 268.8524199695122, 270.04334984756093, 257.5385861280488, 287.3118330792683, 284.9299733231707, 236.69731326219514, 289.0982278963415, 250.98847179878047, 257.83631859756093, 262.0045731707317, 267.3637576219512, 288.5027629573171, 287.3118330792683, 294.7551448170732, 287.9072980182927, 268.8524199695122, 264.3864329268293, 276.2957317073171, 292.3732850609756, 260.2181783536585, 287.3118330792683, 242.65196265243904, 295.6483422256098, 275.1048018292683, 299.5188643292683, 304.2825838414634, 301.9007240853659, 322.4442644817073, 319.7646722560976, 313.5122903963415, 323.9329268292683, 310.2372332317073], [315.2986852134146, 318.2760099085366, 266.7682926829268, 293.5642149390244, 304.5803163109756, 225.08574695121953, 296.2438071646341, 287.9072980182927, 267.9592225609756, 276.5934641768293, 237.29277820121953, 277.4866615853659, 311.1304306402439, 287.0141006097561, 289.0982278963415, 274.5093368902439, 271.2342797256098, 306.9621760670732, 292.96875, 263.1955030487805, 244.4383574695122, 224.49028201219514, 254.85899390243904, 252.47713414634148, 264.9818978658537, 248.6066120426829, 262.3023056402439, 242.94969512195124, 272.7229420731707, 256.34765625, 291.1823551829268, 294.1596798780488, 270.6388147865854, 283.739043445122, 309.0463033536585, 252.1794016768293, 327.5057164634146, 262.0045731707317, 254.85899390243904, 305.17578125, 256.34765625, 296.8392721036585, 294.7551448170732, 295.3506097560976, 339.1172827743902, 308.7485708841463, 300.1143292682927, 309.0463033536585, 341.4991425304878, 334.9490282012195], [295.946074695122, 258.7295160060976, 291.1823551829268, 273.9138719512195, 327.2079839939024, 299.5188643292683, 277.1889291158537, 253.96579649390242, 315.0009527439024, 255.7521913109756, 300.41206173780483, 253.37033155487805, 275.99799923780483, 315.89415015243907, 257.83631859756093, 295.0528772865854, 274.8070693597561, 222.70388719512195, 281.9526486280488, 254.26352896341461, 255.45445884146343, 290.8846227134146, 227.16987423780486, 219.1310975609756, 254.85899390243904, 259.0272484756098, 230.44493140243904, 304.2825838414634, 223.59708460365852, 211.9855182926829, 243.8428925304878, 308.153105945122, 272.7229420731707, 294.7551448170732, 267.9592225609756, 277.4866615853659, 270.04334984756093, 300.1143292682927, 275.4025342987805, 276.5934641768293, 270.04334984756093, 267.9592225609756, 276.8911966463415, 352.51524390243907, 312.3213605182927, 323.3374618902439, 273.0206745426829, 323.9329268292683, 308.153105945122, 342.0946074695122], [345.0719321646341, 283.739043445122, 276.8911966463415, 296.5415396341463, 280.4639862804878, 246.52248475609758, 236.1018483231707, 292.6710175304878, 275.7002667682927, 301.9007240853659, 294.45741234756093, 303.9848513719512, 256.6453887195122, 287.0141006097561, 239.9723704268293, 266.1728277439024, 263.79096798780483, 228.06307164634148, 283.4413109756098, 249.49980945121953, 262.0045731707317, 242.65196265243904, 236.69731326219514, 249.7975419207317, 274.5093368902439, 262.0045731707317, 246.82021722560975, 230.44493140243904, 236.69731326219514, 278.6775914634146, 259.6227134146341, 253.37033155487805, 271.532012195122, 285.8231707317073, 252.47713414634148, 294.1596798780488, 265.8750952743902, 289.6936928353659, 276.2957317073171, 316.7873475609756, 308.4508384146341, 266.1728277439024, 314.405487804878, 280.76171875, 324.2306592987805, 340.0104801829268, 355.49256859756093, 287.6095655487805, 290.2891577743902, 308.4508384146341], [325.1238567073171, 310.8326981707317, 303.68711890243907, 317.0850800304878, 272.1274771341463, 258.1340510670732, 288.20503048780483, 263.1955030487805, 282.25038109756093, 286.7163681402439, 318.87147484756093, 250.3930068597561, 281.6549161585366, 301.9007240853659, 292.3732850609756, 251.58393673780486, 274.2116044207317, 265.8750952743902, 269.7456173780488, 234.61318597560975, 260.2181783536585, 237.8882431402439, 240.56783536585365, 264.0887004573171, 249.20207698170734, 249.7975419207317, 277.1889291158537, 308.4508384146341, 259.324980945122, 249.7975419207317, 246.82021722560975, 253.37033155487805, 241.16330030487805, 260.8136432926829, 255.7521913109756, 281.9526486280488, 296.5415396341463, 286.7163681402439, 306.9621760670732, 254.26352896341461, 287.9072980182927, 282.5481135670732, 243.5451600609756, 301.6029916158537, 295.3506097560976, 345.6673971036585, 292.0755525914634, 324.2306592987805, 331.9717035060976, 306.0689786585366], [324.5283917682927, 289.6936928353659, 296.8392721036585, 277.4866615853659, 272.4252096036585, 272.4252096036585, 286.1209032012195, 247.11794969512195, 320.9556021341463, 322.7419969512195, 295.3506097560976, 255.15672637195124, 257.83631859756093, 265.8750952743902, 232.82679115853657, 253.07259908536585, 259.6227134146341, 245.62928734756096, 221.81068978658539, 239.9723704268293, 219.1310975609756, 231.04039634146343, 282.5481135670732, 254.85899390243904, 226.57440929878047, 262.8977705792683, 258.7295160060976, 251.28620426829266, 263.79096798780483, 291.48008765243907, 230.44493140243904, 261.11137576219517, 265.577362804878, 283.739043445122, 290.8846227134146, 281.0594512195122, 291.48008765243907, 234.01772103658539, 308.7485708841463, 291.1823551829268, 306.3667111280488, 288.20503048780483, 314.1077553353659, 298.3279344512195, 314.1077553353659, 336.7354230182927, 326.9102515243902, 330.1853086890244, 315.5964176829268, 310.2372332317073], [345.6673971036585, 281.9526486280488, 314.7032202743902, 283.4413109756098, 273.6161394817073, 274.2116044207317, 270.6388147865854, 252.47713414634148, 284.9299733231707, 278.6775914634146, 268.2569550304878, 258.7295160060976, 244.140625, 253.37033155487805, 250.6907393292683, 231.93359375, 233.7199885670732, 240.86556783536585, 265.2796303353659, 260.8136432926829, 258.7295160060976, 253.07259908536585, 274.2116044207317, 279.5707888719512, 246.82021722560975, 256.9431211890244, 295.946074695122, 248.3088795731707, 220.3220274390244, 267.06602515243907, 287.9072980182927, 278.3798589939024, 264.6841653963415, 273.6161394817073, 270.04334984756093, 281.9526486280488, 271.8297446646341, 298.3279344512195, 285.8231707317073, 306.0689786585366, 267.9592225609756, 307.8553734756098, 284.0367759146341, 310.2372332317073, 325.1238567073171, 297.4347370426829, 314.7032202743902, 316.1918826219512, 288.5027629573171, 318.87147484756093], [329.58984375, 313.8100228658537, 278.6775914634146, 279.5707888719512, 304.8780487804878, 258.1340510670732, 301.6029916158537, 251.28620426829266, 299.5188643292683, 277.1889291158537, 284.9299733231707, 306.9621760670732, 288.20503048780483, 205.43540396341461, 234.61318597560975, 237.8882431402439, 235.80411585365852, 252.1794016768293, 246.82021722560975, 258.7295160060976, 234.31545350609758, 232.82679115853657, 234.01772103658539, 185.18959603658536, 234.31545350609758, 309.3440358231707, 252.47713414634148, 297.4347370426829, 248.6066120426829, 260.8136432926829, 283.1435785060976, 271.532012195122, 284.9299733231707, 280.1662538109756, 272.4252096036585, 246.52248475609758, 295.6483422256098, 291.1823551829268, 273.6161394817073, 285.8231707317073, 307.8553734756098, 300.1143292682927, 269.4478849085366, 293.8619474085366, 302.198456554878, 290.2891577743902, 294.45741234756093, 287.9072980182927, 333.4603658536585, 314.405487804878], [342.6900724085366, 300.1143292682927, 266.1728277439024, 320.360137195122, 261.7068407012195, 239.07917301829266, 300.7097942073171, 285.2277057926829, 270.3410823170732, 273.9138719512195, 250.98847179878047, 225.3834794207317, 273.6161394817073, 244.140625, 260.2181783536585, 275.4025342987805, 232.5290586890244, 230.44493140243904, 219.1310975609756, 237.8882431402439, 231.93359375, 275.7002667682927, 280.1662538109756, 277.784394054878, 209.3059260670732, 236.1018483231707, 220.61975990853657, 261.11137576219517, 241.75876524390242, 262.6000381097561, 236.99504573170734, 267.9592225609756, 230.44493140243904, 244.140625, 238.4837080792683, 274.2116044207317, 287.6095655487805, 273.0206745426829, 287.9072980182927, 271.2342797256098, 289.6936928353659, 298.9233993902439, 310.8326981707317, 259.324980945122, 318.87147484756093, 349.24018673780483, 292.0755525914634, 275.99799923780483, 332.2694359756098, 283.1435785060976], [312.0236280487805, 240.56783536585365, 313.2145579268293, 302.198456554878, 278.9753239329268, 271.532012195122, 262.8977705792683, 250.0952743902439, 277.784394054878, 250.6907393292683, 250.3930068597561, 288.8004954268293, 239.9723704268293, 274.5093368902439, 272.1274771341463, 260.5159108231707, 272.1274771341463, 225.08574695121953, 258.7295160060976, 206.03086890243904, 265.577362804878, 273.0206745426829, 219.4288300304878, 244.7360899390244, 268.8524199695122, 288.8004954268293, 200.9694169207317, 276.5934641768293, 281.9526486280488, 267.6614900914634, 278.9753239329268, 235.20865091463415, 261.7068407012195, 286.7163681402439, 244.7360899390244, 239.37690548780486, 286.1209032012195, 283.4413109756098, 316.7873475609756, 257.5385861280488, 305.4735137195122, 257.2408536585366, 267.3637576219512, 323.6351943597561, 293.5642149390244, 320.9556021341463, 312.3213605182927, 318.5737423780488, 322.14653201219517, 288.5027629573171], [335.2467606707317, 293.8619474085366, 264.0887004573171, 284.0367759146341, 311.1304306402439, 312.9168254573171, 262.8977705792683, 267.3637576219512, 259.6227134146341, 239.6746379573171, 283.1435785060976, 222.10842225609758, 283.739043445122, 309.0463033536585, 265.2796303353659, 211.6877858231707, 274.5093368902439, 284.3345083841463, 259.0272484756098, 241.16330030487805, 202.45807926829266, 253.66806402439025, 256.34765625, 242.05649771341461, 233.7199885670732, 218.83336509146343, 280.76171875, 242.3542301829268, 207.8172637195122, 242.3542301829268, 280.76171875, 280.76171875, 239.6746379573171, 262.8977705792683, 287.6095655487805, 259.9204458841463, 272.4252096036585, 275.4025342987805, 301.0075266768293, 324.82612423780483, 303.0916539634146, 287.0141006097561, 280.76171875, 292.6710175304878, 332.8649009146341, 337.3308879573171, 309.0463033536585, 280.4639862804878, 333.7580983231707, 322.14653201219517], [307.8553734756098, 283.4413109756098, 289.991425304878, 272.1274771341463, 256.6453887195122, 306.9621760670732, 289.0982278963415, 254.85899390243904, 242.3542301829268, 308.153105945122, 279.8685213414634, 269.1501524390244, 287.6095655487805, 233.12452362804876, 249.49980945121953, 232.5290586890244, 220.3220274390244, 272.7229420731707, 188.7623856707317, 256.6453887195122, 270.6388147865854, 225.6812118902439, 203.64900914634148, 247.41568216463415, 257.5385861280488, 208.71046112804876, 223.00161966463415, 243.24742759146343, 258.4317835365854, 230.44493140243904, 259.9204458841463, 222.70388719512195, 304.2825838414634, 275.4025342987805, 260.5159108231707, 275.7002667682927, 268.5546875, 293.8619474085366, 248.90434451219514, 302.4961890243902, 261.4091082317073, 307.2599085365854, 293.8619474085366, 308.4508384146341, 315.0009527439024, 316.4896150914634, 330.4830411585366, 315.5964176829268, 320.6578696646341, 307.2599085365854], [311.4281631097561, 326.3147865853659, 301.3052591463415, 338.5218178353659, 308.153105945122, 319.7646722560976, 287.3118330792683, 221.81068978658539, 268.2569550304878, 261.4091082317073, 247.41568216463415, 250.98847179878047, 290.2891577743902, 226.57440929878047, 253.37033155487805, 257.5385861280488, 249.20207698170734, 215.5583079268293, 256.34765625, 275.7002667682927, 301.0075266768293, 265.577362804878, 228.06307164634148, 245.9270198170732, 257.5385861280488, 254.85899390243904, 196.5034298780488, 263.4932355182927, 237.29277820121953, 277.4866615853659, 266.4705602134146, 224.49028201219514, 262.6000381097561, 270.9365472560976, 288.5027629573171, 282.8458460365854, 276.5934641768293, 273.9138719512195, 275.7002667682927, 287.9072980182927, 323.9329268292683, 259.6227134146341, 318.5737423780488, 262.6000381097561, 267.9592225609756, 328.10118140243907, 339.7127477134146, 315.0009527439024, 315.0009527439024, 326.0170541158537], [328.6966463414634, 330.4830411585366, 258.4317835365854, 253.37033155487805, 274.5093368902439, 283.1435785060976, 265.577362804878, 235.50638338414635, 279.8685213414634, 243.24742759146343, 295.3506097560976, 215.2605754573171, 291.7778201219512, 249.7975419207317, 250.6907393292683, 236.99504573170734, 248.3088795731707, 276.8911966463415, 251.28620426829266, 253.37033155487805, 262.6000381097561, 228.95626905487805, 256.6453887195122, 256.34765625, 276.2957317073171, 218.23790015243904, 229.84946646341461, 245.03382240853657, 243.24742759146343, 265.577362804878, 244.7360899390244, 225.6812118902439, 270.6388147865854, 272.7229420731707, 272.1274771341463, 286.1209032012195, 267.6614900914634, 269.1501524390244, 251.8816692073171, 275.99799923780483, 289.0982278963415, 252.47713414634148, 295.0528772865854, 299.2211318597561, 318.5737423780488, 317.6805449695122, 320.6578696646341, 316.7873475609756, 341.4991425304878, 282.8458460365854], [257.2408536585366, 277.784394054878, 312.61909298780483, 266.4705602134146, 300.41206173780483, 272.4252096036585, 306.0689786585366, 273.0206745426829, 259.9204458841463, 297.4347370426829, 287.6095655487805, 298.9233993902439, 261.7068407012195, 244.7360899390244, 257.5385861280488, 237.29277820121953, 251.58393673780486, 224.1925495426829, 261.4091082317073, 250.0952743902439, 257.2408536585366, 257.83631859756093, 259.324980945122, 267.3637576219512, 257.2408536585366, 287.6095655487805, 244.4383574695122, 249.49980945121953, 241.16330030487805, 224.49028201219514, 253.66806402439025, 259.9204458841463, 240.27010289634148, 275.7002667682927, 264.3864329268293, 291.1823551829268, 256.6453887195122, 294.45741234756093, 270.3410823170732, 281.0594512195122, 306.9621760670732, 293.2664824695122, 281.9526486280488, 260.8136432926829, 273.9138719512195, 309.0463033536585, 325.7193216463415, 342.0946074695122, 311.1304306402439, 293.5642149390244], [298.3279344512195, 299.8165967987805, 303.9848513719512, 299.5188643292683, 305.17578125, 272.4252096036585, 312.61909298780483, 284.0367759146341, 237.8882431402439, 229.84946646341461, 245.62928734756096, 309.93950076219517, 241.16330030487805, 265.8750952743902, 268.2569550304878, 248.3088795731707, 262.0045731707317, 211.6877858231707, 251.58393673780486, 253.37033155487805, 251.58393673780486, 211.9855182926829, 236.99504573170734, 259.9204458841463, 264.6841653963415, 259.9204458841463, 239.07917301829266, 249.20207698170734, 262.6000381097561, 281.0594512195122, 271.532012195122, 223.8948170731707, 280.4639862804878, 305.4735137195122, 243.8428925304878, 296.5415396341463, 291.48008765243907, 310.2372332317073, 250.6907393292683, 302.198456554878, 284.6322408536585, 283.1435785060976, 300.41206173780483, 302.7939214939024, 292.3732850609756, 302.4961890243902, 288.5027629573171, 314.7032202743902, 333.4603658536585, 302.4961890243902]]
  out "error out":errorcluster
  in  "Reading thresholds":dbl[](array[numeric])=[0.0, 0.0, 0.0]
  in  "Reading thresholds defaults":dbl[](array[numeric])=[0.0, 0.0, 0.0]
  in  "Preset PMT2":dbl=0.7 format="%.2f"
  in  "Scan Parameters":T4={"x pixels"=50, "x voltage min"=-7.0, "x voltage max"=9.0, "y voltage min"=-8.75, "y voltage max"=7.25, "fill frac"=0.5, "Zoom"=4.0, "BiDi"=FALSE, "scan rate (ms/line)"=4.0} {"fill frac" min=0.0 step=0.05 format="%.2f"; "y voltage max" format="%0.2p"; "y voltage min" format="%.2f"; "x voltage max" format="%0.2p"; "x voltage min" format="%0.2p"}
  in  "Preset PMT1":dbl=0.7 format="%.2g"
  in  "Hardware Settings":T5={"Galvo Channels"="Dev1/ao0:1", "Detector Channels"="Dev1/ai0:2", "Galvo Trigger"="/Dev1/ai/StartTrigger", "Shutter Lines"=["Dev1/port0/line7"], "Max Acquisition Rate"=5000000.0, "Recommended Acquisition Rate"=5000000.0, "Galvo Write Rate"=2500000.0, "Max Timebase Frequency (Hz)"=20000000.0, "MCC Shutter Lines"=["Dev0/AuxPort/Do1", "Dev0/AuxPort/Do2"], "Detector Task"="", "Shutter Tasks"=[], "Galvo Task"="", "Digital Image Multiplier"=[100.0, 100.0, 100.0]} {"Max Acquisition Rate" min=0.0 max=5000000.0 step=100000.0}
  out "Actual scan rate ms/line":dbl=3.3696 format="%#_3g"
  out "frames/sec":dbl=1.1592622269705604 format="%#_3g"
  in  "show flyback data":bool
  in  "disable averaging":bool
  in  "PMTs":T6={"PMT1"="Dev0/Ao0", "PMT2"="Dev0/Ao1", "PMT3"="Dev0/Ao2"}
  in  "Preset PMT3":dbl=0.7 format="%.2g"
  in  "Pass UI values":bool
  in  "configuration file":path=path "C:/Users/Trent/Dropbox/Shared/Jeremy/microscoper 2012/ConfigFiles/Jeremy.ini"
  # "Stage Controls"
  # "Detector Controls"
  # "575-625 nm"
  # "360-520 nm and < 425nm = 360-425 nm"
  # "425 nm - 775 nm"
  # "Image Controls"
  # "Scan Controls"
  # "Channel 1"
  # "Channel 2"
  # "Channel 3"
  # "File Controls"
  # "Photon Counting"
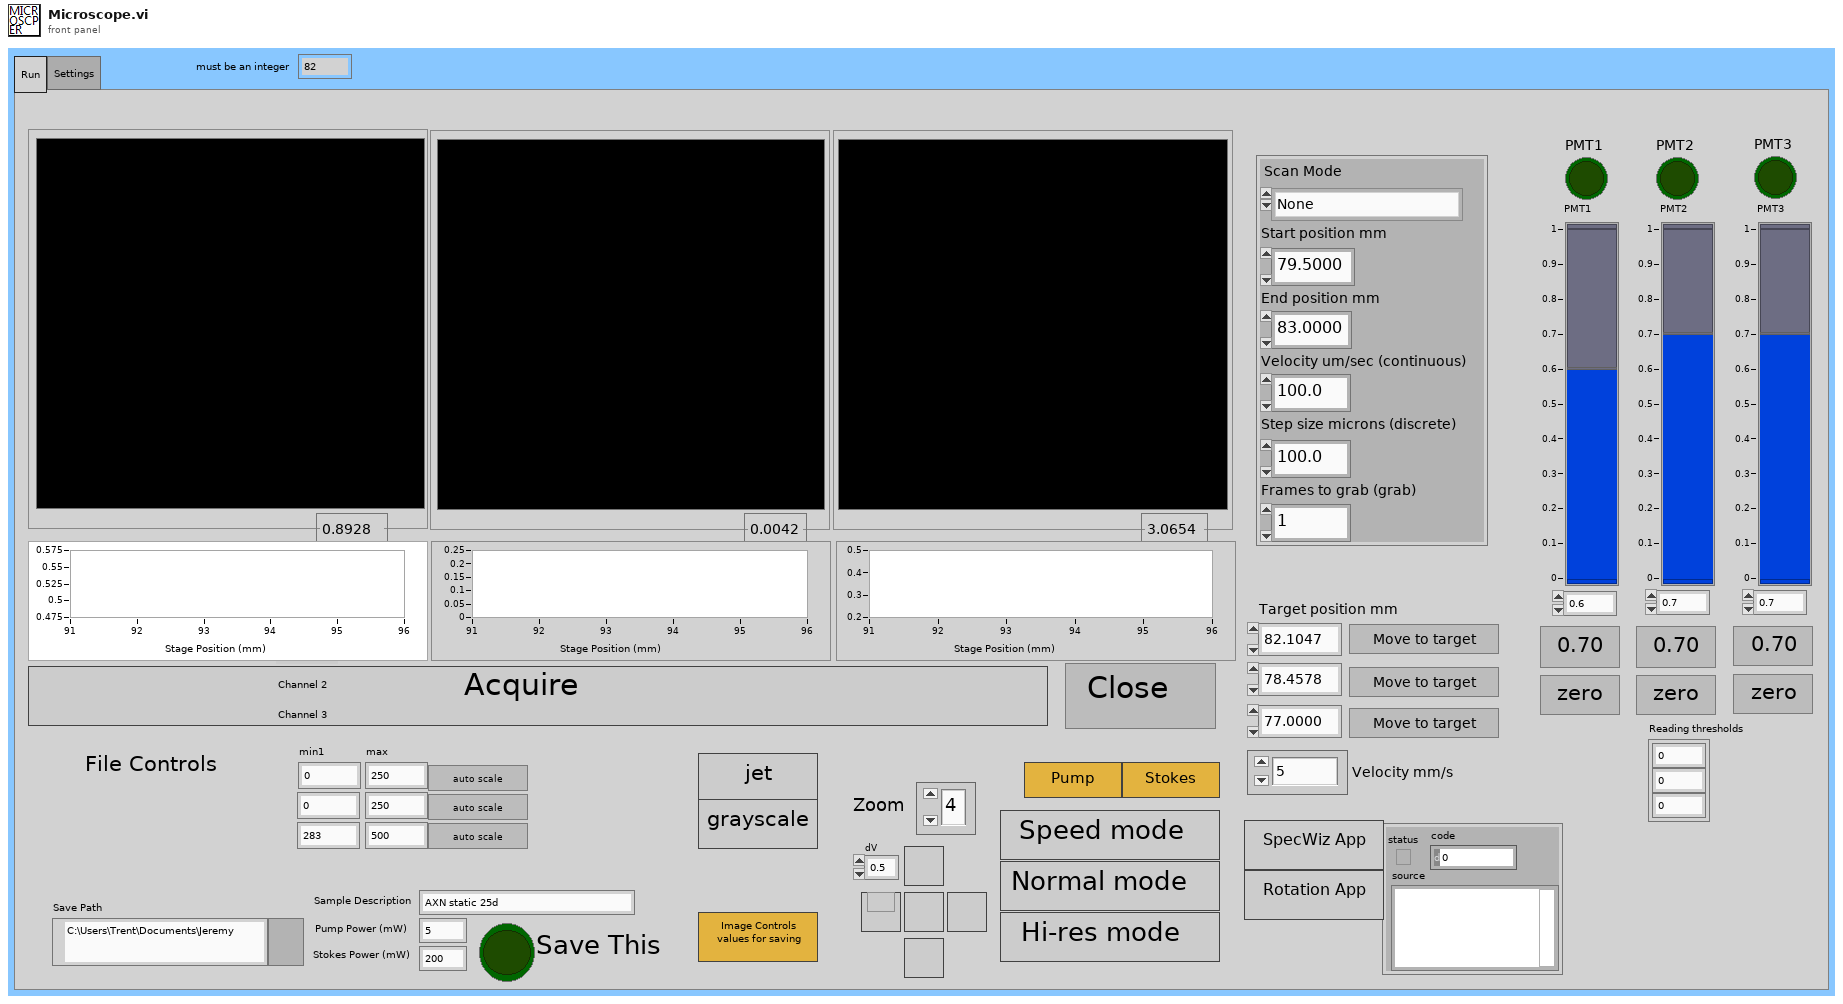
[diagram p1: front panel]
types:
  T1 = typedef "Graph.ctl" = cluster{dbl[], dbl[]}
  T2 = typedef "Stage Parameters.ctl" = cluster{"Scan Mode":T3, "Start position mm":dbl, "End position mm":dbl, "Velocity um/sec (continuous)":dbl, "Step size microns (discrete)":dbl, "Frames to grab (grab)":i32}
  T3 = typedef "ScanMode.ctl" = enum16{"None", "Continuous", "Point Scan (CH3 cursor)", "Point Scan Move (CH3 cursor)", "Grab", "Grab Move Stage", "Grab Move Z-stage", "Cont. Move Z-stage", "Spec Move Stage", "Spec Move Cont", "Surf Calib"}
  T4 = typedef "Scan Parameters.ctl" = cluster{"x pixels":i32, "x voltage min":dbl, "x voltage max":dbl, "y voltage min":dbl, "y voltage max":dbl, "fill frac":dbl, "Zoom":dbl, "BiDi":bool, "scan rate (ms/line)":dbl}
  T5 = typedef "HWsettings.ctl" = cluster{"Galvo Channels":tag, "Detector Channels":tag, "Galvo Trigger":tag, "Shutter Lines":tag[], "Max Acquisition Rate":dbl, "Recommended Acquisition Rate":dbl, "Galvo Write Rate":dbl, "Max Timebase Frequency (Hz)":dbl, "MCC Shutter Lines":refnum<k21>[], "Detector Task":refnum<k21>, "Shutter Tasks":refnum<k21>[], "Galvo Task":refnum<k21>, "Digital Image Multiplier":dbl[]}
  T6 = typedef "PMTs.ctl" = cluster{"PMT1":refnum<k21>, "PMT2":refnum<k21>, "PMT3":refnum<k21>}
  T7 = typedef "StageEvent.ctl" = enum16{"stage.TimeOut", "stage.FlushData", "stage.GetPosition", "stage.Init", "stage.MoveTo1", "stage.MoveTo2", "stage.MoveTo3", "stage.Stop"}
  T8 = enum32{"Invalid", "Standard", "Closed", "Hidden", "Minimized", "Maximized"}
  T9 = typedef "MicroscopeEvent.ctl" = enum16{"M.Wait", "M.RunRotation", "M.Flush", "M.Init", "M.InitStage", "M.InitImageData", "M.ReinitImageData", "M.ReinitImageParams", "M.GetSetParams", "M.InitFastHardware", "M.Pre-Acquire", "M.Acquire", "M.PostAcquire", "M.StopAcquire", "M.SetAcqStatusTrue", "M.SetAcqStatusFalse", "M.ClearImageData", "M.MoveStageDiscrete", "M.MoveStageToTarget1", "M.MoveStageToTarget2", "M.MoveStageToTarget3", "M.OpenShutters", "M.CloseShutters", "M.StartAcquireSequence", "M.ChangeParameters", "M.OpenStokes", "M.OpenPump", "M.RunSW"}
  T10 = typedef "Move Type.ctl" = enum16{"None", "Continuous", "Discrete"}
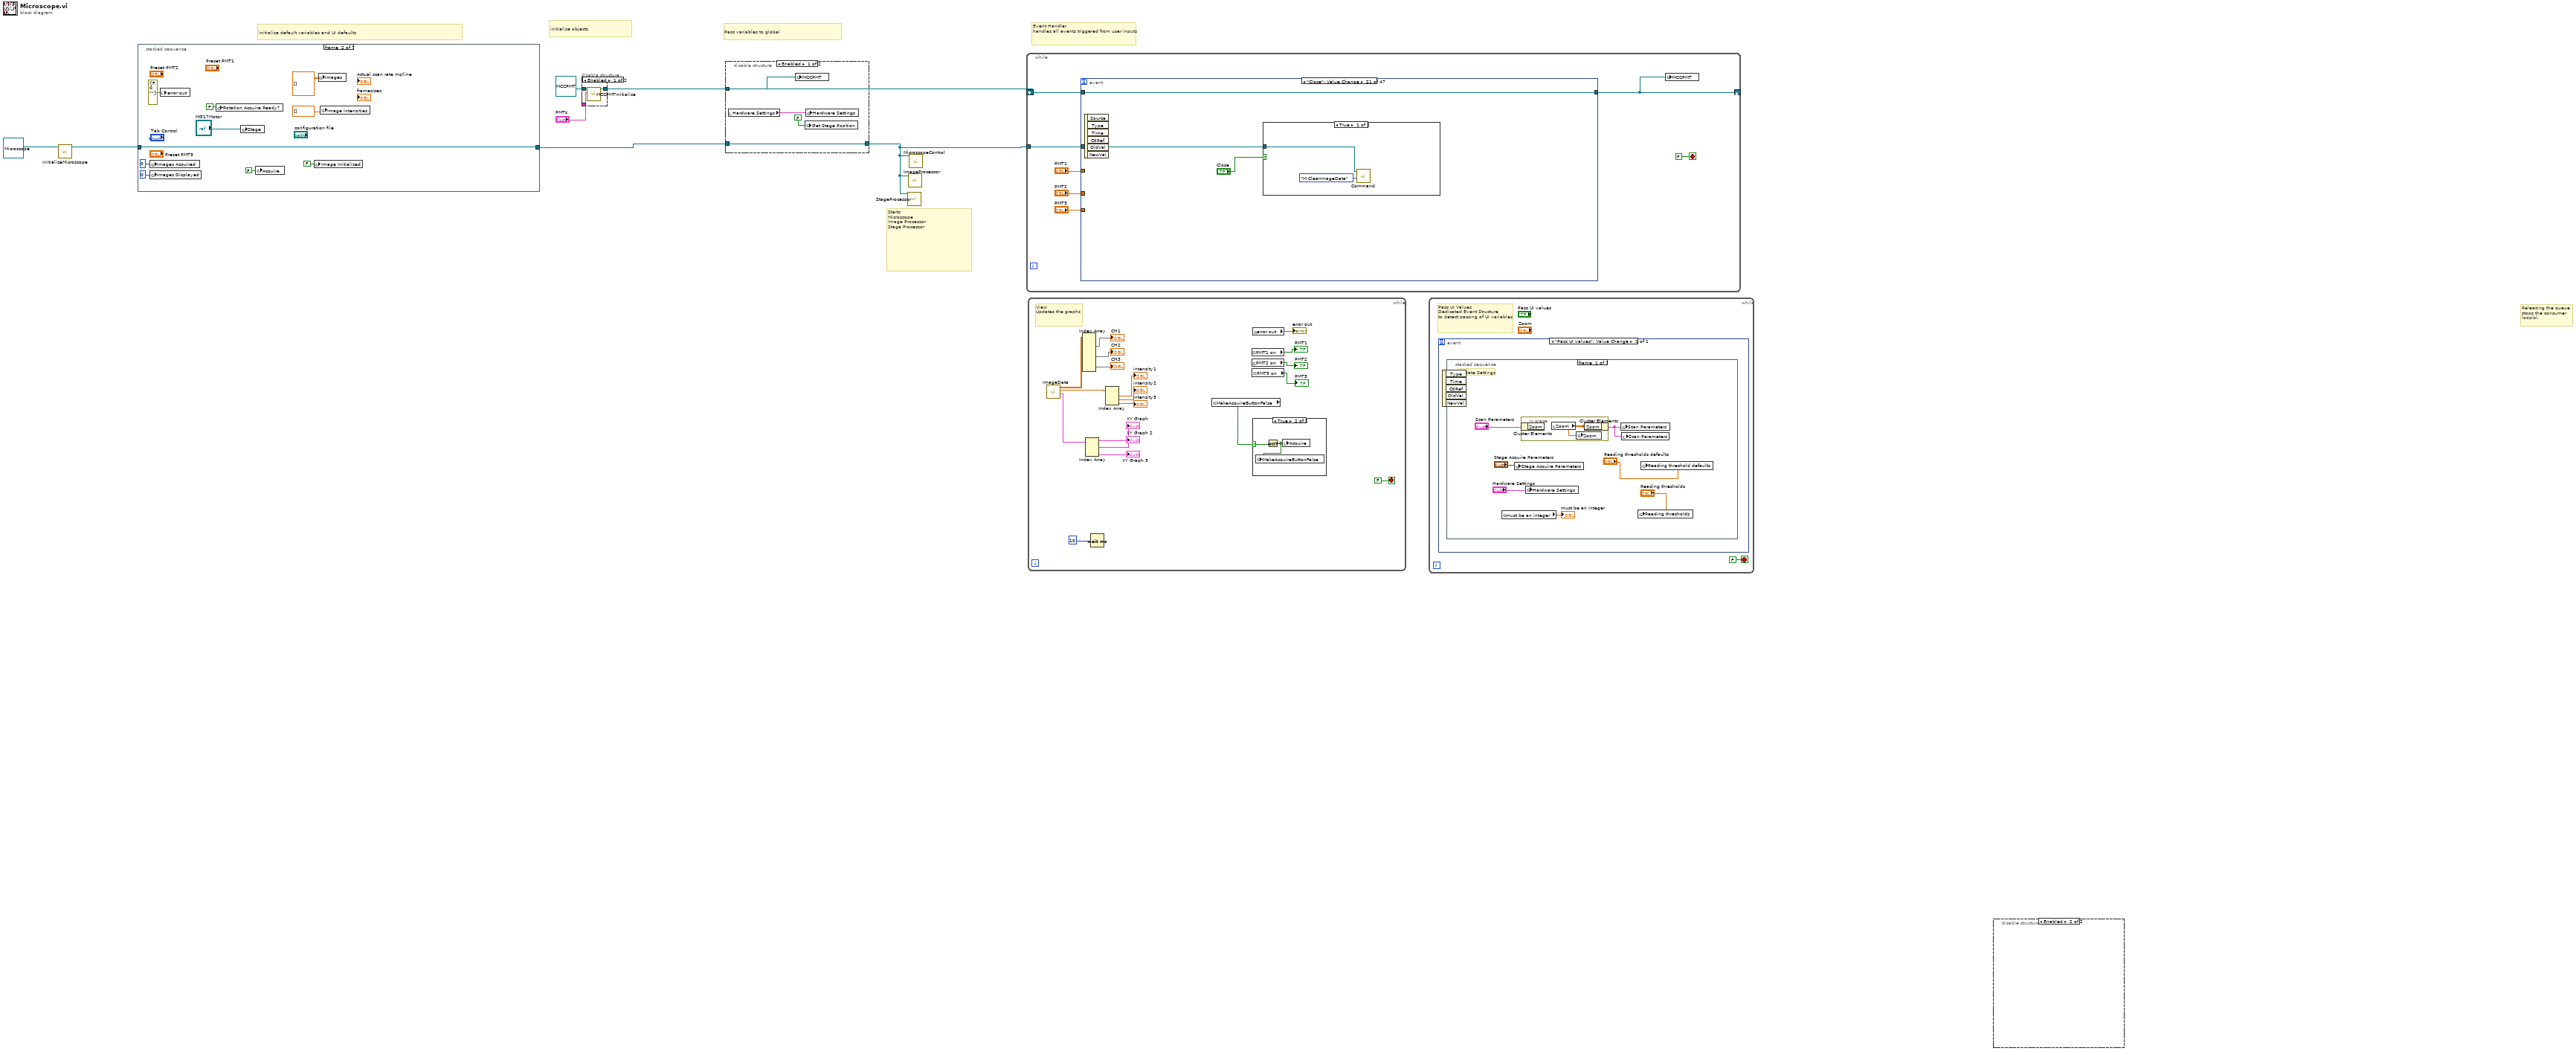
[diagram p0: block diagram]
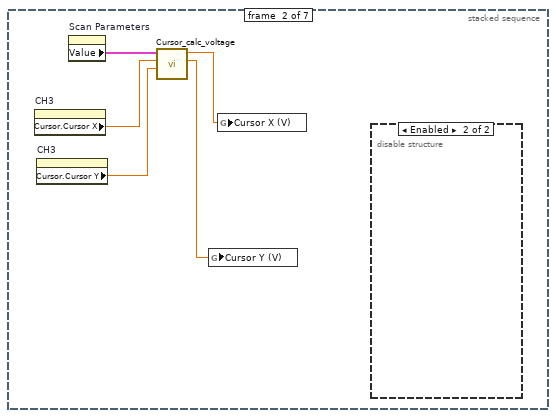
[diagram p2: hidden frame]
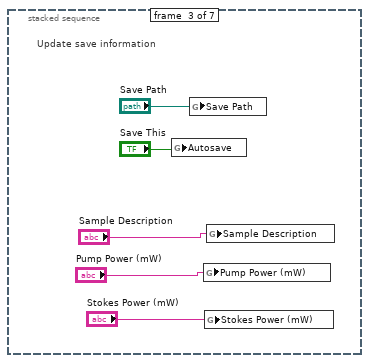
[diagram p4: hidden frame]
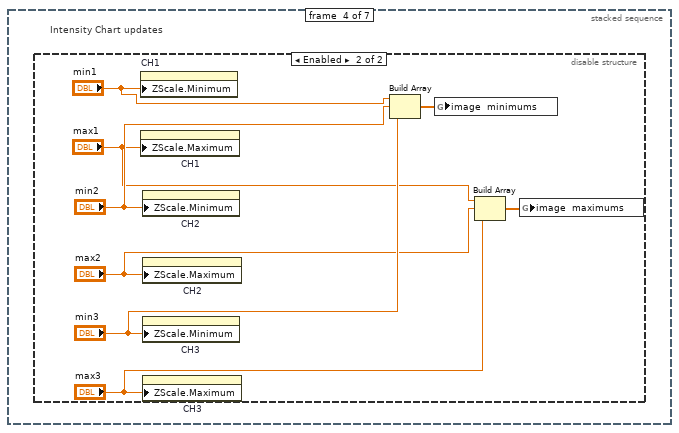
[diagram p5: hidden frame]
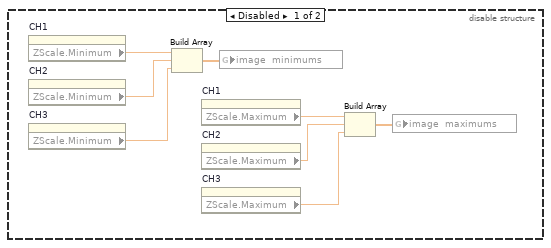
[diagram p6: hidden frame]
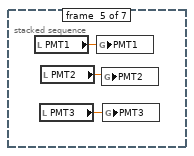
[diagram p7: hidden frame]
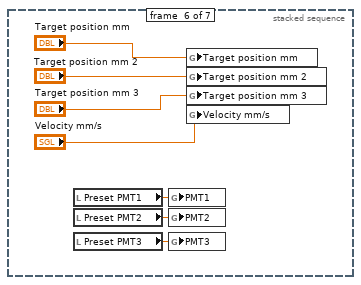
[diagram p8: hidden frame]
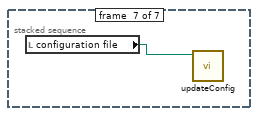
[diagram p9: hidden frame]
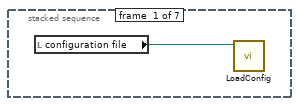
[diagram p13: hidden frame]
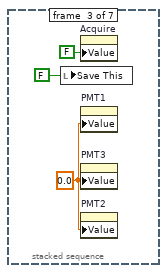
[diagram p14: hidden frame]
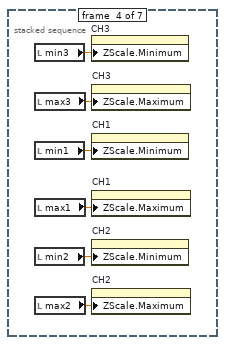
[diagram p15: hidden frame]
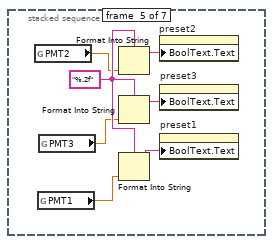
[diagram p16: hidden frame]
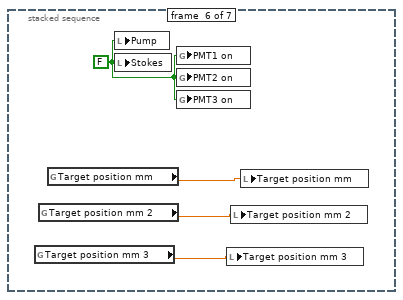
[diagram p17: hidden frame]
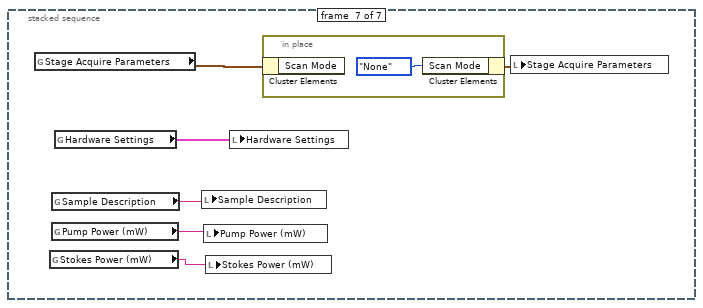
[diagram p18: hidden frame]
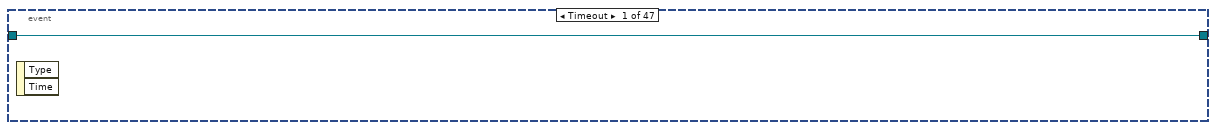
[diagram p19: hidden frame]
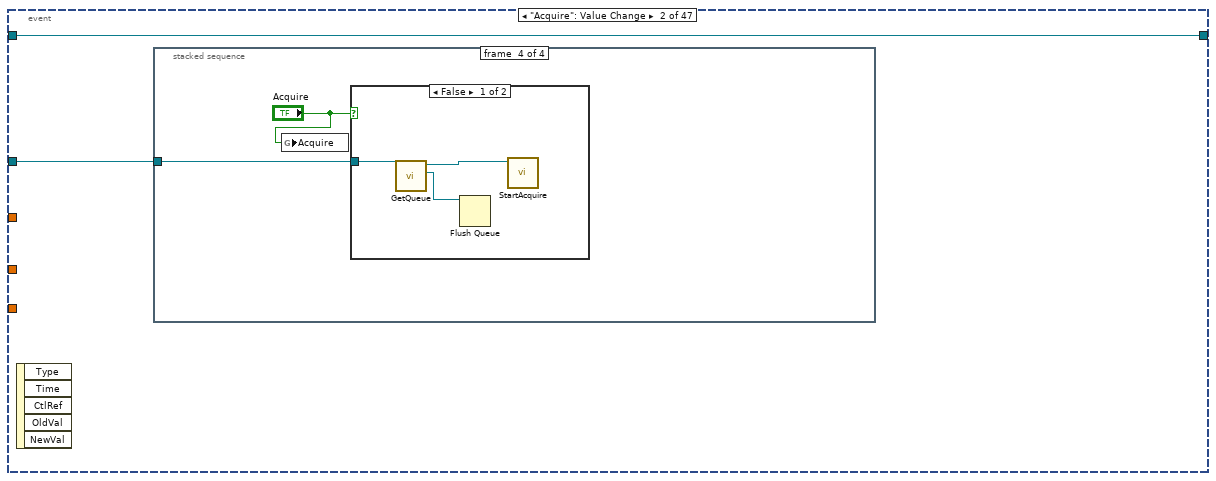
[diagram p20: hidden frame]
diagram:
  # "Starts\nMicroscope\nImage Processor\nStage Processor"
  # "Pass variables to global"
  # "initialize objects"
  # "initialize default variables and UI defaults"
  # "Event Handler\nhandles all events triggered from user inputs"
  # "Releasing the queue stops the consumer loop(s)."
  n1 = call "InitializeMicroscope.vi"("Microscope in"=refnum<class "Microscope.lvclass"> refnum ("Microscope.lvclass")) -> ("Microscope out"=w2:refnum<class "Microscope.lvclass">)  [unwired: 9 in, 1 out]
  n2 = stacked-sequence {
    tunnel: [_ w12 _ _ _ _ _] -> w1
    tunnel: w2 -> [_ w12 _ _ _ _ _]
    frame #0 {
      n3 = local read "configuration file"() -> (w8:path)
      n4 = call "LoadConfig.vi"("configuration file"=w8) -> ()  [unwired: 11 in]
    }
    frame #1 {
      n5 = global write "GlobalUI.vi" "Images Acquired"(0 ("Dgrabbed")) -> ()
      n6 = global write "GlobalUI.vi" "Images Displayed"(0 ("Frames grabbed")) -> ()
      n7 = local write "error out"(errorcluster {"status"=FALSE, "code"=0, "source"=""} ("error out")) -> ()
      n8 = global write "GlobalUI.vi" "Rotation Acquire Ready?"(FALSE ("Acquire Ready?")) -> ()
      n9 = global write "GlobalUI.vi" "Stage"("MG17Motor") -> ()
      n10 = global write "GlobalUI.vi" "Acquire"(FALSE ("Acquire")) -> ()
      n11 = global write "GlobalUI.vi" "Image Initialized"(FALSE ("Image Initialized")) -> ()
      n12 = global write "GlobalUI.vi" "Images"(dbl[][][] [] ("Images")) -> ()
      n13 = global write "GlobalUI.vi" "Image intensities"(dbl[] [] ("Images")) -> ()
    }
    frame #2 {
      w19 = 0.0 ("PMT1")
      n14 = local write "Save This"(FALSE ("Autosave")) -> ()
      n15 = property on="Acquire" class="Bool (strict)"("Value"=FALSE ("Acquire")) -> ()  [unwired: 2 in, 2 out]
      n16 = property on="PMT1" class="Slide (strict)"("Value"=w19) -> ()  [unwired: 2 in, 2 out]
      n17 = property on="PMT3" class="Slide (strict)"("Value"=w19) -> ()  [unwired: 2 in, 2 out]
      n18 = property on="PMT2" class="Slide (strict)"("Value"=w19) -> ()  [unwired: 2 in, 2 out]
    }
    frame #3 {
      n19 = local read "min3"() -> (w26:dbl)
      n20 = local read "max3"() -> (w27:dbl)
      n21 = local read "min1"() -> (w22:dbl)
      n22 = local read "max1"() -> (w23:dbl)
      n23 = local read "min2"() -> (w24:dbl)
      n24 = local read "max2"() -> (w25:dbl)
      n25 = property on="CH3" class="IntGraph (strict)"("ZScale.Minimum"=w26) -> ()  [unwired: 2 in, 2 out]
      n26 = property on="CH3" class="IntGraph (strict)"("ZScale.Maximum"=w27) -> ()  [unwired: 2 in, 2 out]
      n27 = property on="CH1" class="IntGraph (strict)"("ZScale.Minimum"=w22) -> ()  [unwired: 2 in, 2 out]
      n28 = property on="CH1" class="IntGraph (strict)"("ZScale.Maximum"=w23) -> ()  [unwired: 2 in, 2 out]
      n29 = property on="CH2" class="IntGraph (strict)"("ZScale.Minimum"=w24) -> ()  [unwired: 2 in, 2 out]
      n30 = property on="CH2" class="IntGraph (strict)"("ZScale.Maximum"=w25) -> ()  [unwired: 2 in, 2 out]
    }
    frame #4 {
      w32 = "%.2f" ("format string")
      n31 = global read "GlobalUI.vi" "PMT2"() -> (w28:dbl)
      n32 = global read "GlobalUI.vi" "PMT1"() -> (w30:dbl)
      n33 = global read "GlobalUI.vi" "PMT3"() -> (w29:dbl)
      n34 = Format Into String(format string=w32, w28) -> (resulting string=w33:string)  [unwired: 2 in, 1 out]
      n35 = Format Into String(format string=w32, w29) -> (resulting string=w31:string)  [unwired: 2 in, 1 out]
      n36 = Format Into String(format string=w32, w30) -> (resulting string=w34:string)  [unwired: 2 in, 1 out]
      n37 = property on="preset2" class="Bool"("BoolText.Text"=w33) -> ()  [unwired: 2 in, 2 out]
      n38 = property on="preset3" class="Bool"("BoolText.Text"=w31) -> ()  [unwired: 2 in, 2 out]
      n39 = property on="preset1" class="Bool"("BoolText.Text"=w34) -> ()  [unwired: 2 in, 2 out]
    }
    frame #5 {
      w38 = FALSE ("PMT2 on")
      n40 = global read "GlobalUI.vi" "Target position mm 3"() -> (w35:dbl)
      n41 = global read "GlobalUI.vi" "Target position mm 2"() -> (w36:dbl)
      n42 = global read "GlobalUI.vi" "Target position mm"() -> (w37:dbl)
      n43 = local write "Pump"(w38) -> ()
      n44 = local write "Stokes"(w38) -> ()
      n45 = global write "GlobalUI.vi" "PMT1 on"(w38) -> ()
      n46 = global write "GlobalUI.vi" "PMT2 on"(w38) -> ()
      n47 = global write "GlobalUI.vi" "PMT3 on"(w38) -> ()
      n48 = local write "Target position mm 3"(w35) -> ()
      n49 = local write "Target position mm 2"(w36) -> ()
      n50 = local write "Target position mm"(w37) -> ()
    }
    frame #6 {
      n51 = global read "GlobalUI.vi" "Stage Acquire Parameters"() -> (w43:T2)
      n52 = global read "GlobalUI.vi" "Stokes Power (mW)"() -> (w39:string)
      n53 = global read "GlobalUI.vi" "Sample Description"() -> (w41:string)
      n54 = global read "GlobalUI.vi" "Pump Power (mW)"() -> (w40:string)
      n55 = global read "GlobalUI.vi" "Hardware Settings"() -> (w42:T5)
      n56 = local write "Sample Description"(w41) -> ()
      n57 = local write "Pump Power (mW)"(w40) -> ()
      n58 = local write "Stokes Power (mW)"(w39) -> ()
      n59 = local write "Hardware Settings"(w42) -> ()
      n60 = in-place {
        n61 = in-place-cluster #1(w43) -> ()  [unwired: 1 out]
        n62 = in-place-cluster #1("Scan Mode"=ScanMode."None") -> (w44:T2)
      }
      n63 = local write "Stage Acquire Parameters"(w44) -> ()
    }
  }
  n64 = disable-structure shown="Enabled" {
    disable-tunnel: [w48 w49] -> w6
    disable-tunnel: refnum<class "MCCPMT.lvclass"> refnum ("MCCPMT.lvclass") -> [w47 w49]
    disable-tunnel: "PMTs" -> [w46 _]
    frame Enabled {
      n65 = call "MCCPMTInitialize.vi"("PMTs"=w46, "MCCPMT in"=w47) -> ("MCCPMT out"=w48:refnum<class "MCCPMT.lvclass">)  [unwired: 8 in, 1 out]
    }
    frame Disabled {
    }
  }
  n66 = disable-structure shown="Enabled" {
    disable-tunnel: w6 -> [w53 _]
    disable-tunnel: [w50 _] -> w3
    disable-tunnel: w1 -> [w50 _]
    frame Enabled {
      n67 = local read "Hardware Settings"() -> (w51:T5)
      n68 = global write "GlobalUI.vi" "MCCPMT"(w53) -> ()
      n69 = global write "GlobalUI.vi" "Get Stage Position"(FALSE ("Get Stage Position")) -> ()
      n70 = global write "GlobalUI.vi" "Hardware Settings"(w51) -> ()
    }
    frame Disabled {
    }
  }
  n71 = call "StageProcessor.vi"("Microscope in"=w3) -> ()  [unwired: 11 in]
  n72 = call "ImageProcessor.vi"("Microscope in"=w3) -> ()  [unwired: 10 in, 1 out]
  n73 = call "MicroscopeControl.vi"("Microscope in"=w3) -> ()  [unwired: 14 in, 1 out]
  n74 = while {
    shift-right: [w56] -> _
    shift-left: w6 -> [w60]
    tunnel: w3 -> [w55]
    stop <- FALSE stop-if-true
    n75 = event shown="[20] \"Close\": Value Change" {
      selector: _ -> [_ _ _ _ _ _ _ _ _ _ _ _ _ _ _ _ _ _ _ _ _ _ _ _ _ _ _ _ _ _ _ _ _ _ _ _ _ _ _ _ _ _ _ _ _ _ _]
      dyn-events: _ -> [_ _ _ _ _ _ _ _ _ _ _ _ _ _ _ _ _ _ _ _ _ _ _ _ _ _ _ _ _ _ _ _ _ _ _ _ _ _ _ _ _ _ _ _ _ _ _]
      timeout: _ -> [_ _ _ _ _ _ _ _ _ _ _ _ _ _ _ _ _ _ _ _ _ _ _ _ _ _ _ _ _ _ _ _ _ _ _ _ _ _ _ _ _ _ _ _ _ _ _]
      tunnel: w60 -> [w61 w63 w83 w87 w95 w103 w111 w121 w151 w208 w227 w232 w303 w313 w330 w347 w360 w386 w412 w433 w456 w459 w486 w508 w530 w549 w554 w556 w559 w561 w563 w565 w567 w574 w581 w588 w590 w591 w593 w595 w597 w603 w613 w630 w647 w666 w682]
      tunnel: [w61 w63 w83 w87 w95 w103 w111 w121 w151 w208 w227 w232 w303 w313 w330 w347 w360 w386 w412 w433 w456 w459 w485 w507 w529 w549 w554 w556 w559 w561 w563 w565 w567 w574 w581 w588 w590 w591 w593 w595 w597 w603 w612 w629 w646 w667 w682] -> w56
      tunnel: "PMT1" -> [_ _ _ _ _ _ _ _ _ _ _ _ _ _ _ _ _ _ _ _ _ _ _ w506 w527 _ _ _ _ _ _ _ _ _ _ _ _ _ _ _ _ _ _ _ _ _ _]
      tunnel: "PMT2" -> [_ _ _ _ _ _ _ _ _ _ _ _ _ _ _ _ _ _ _ _ _ _ w484 _ w528 _ _ _ _ _ _ _ _ _ _ _ _ _ _ _ _ _ _ _ _ _ _]
      tunnel: "PMT3" -> [_ _ _ _ _ _ _ _ _ _ _ _ _ _ _ _ _ _ _ _ _ _ w483 w505 _ _ _ _ _ _ _ _ _ _ _ _ _ _ _ _ _ _ _ _ _ _ _]
      tunnel: w55 -> [_ w62 _ _ _ _ _ w118 w148 w207 _ _ _ _ _ _ w358 w384 w410 _ w454 _ _ _ _ w545 _ _ _ _ _ _ _ _ _ _ _ _ _ _ _ w599 _ _ _ _ _]
      event Timeout {
        n76 = event-data() -> ()  [unwired: 1 in, 2 out]
      }
      event "Acquire": Value Change {
        n77 = event-data() -> ()  [unwired: 1 in, 5 out]
        n78 = stacked-sequence {
          tunnel: w62 -> [_ _ _ w78]
          frame #0 {
            n79 = control-ref of="CH2"() -> (w65:refnum<vi>)
            n80 = control-ref of="CH1"() -> (w66:refnum<vi>)
            n81 = control-ref of="CH3"() -> (w67:refnum<vi>)
            n82 = local read "Scan Parameters"() -> (w64:T4)
            n83 = call "fixgraphs.vi"("Scan Parameters"=w64, "IntGraph Refnum 3"=w67, "IntGraph Refnum in"=w66, "IntensityGraph in"=w65) -> ()  [unwired: 8 in]
          }
          frame #1 {
            # "Update Graph information"
            n84 = local read "Stage Acquire Parameters"() -> (w71:T2)
            n85 = Unbundle By Name(w71) -> ("Scan Mode"=w69:T3)
            n86 = call "GetScanMoveType.vi"("Scan Mode"=w69) -> ("Move Type"=w68:T10)  [unwired: 8 in, 2 out]
            n87 = call "isStaticScan.vi"("Move Type"=w68) -> ("Boolean"=w72:bool)  [unwired: 10 in]
            n88 = case shown="True" w72 {
              tunnel: ["Stage Position (mm)" "Time Elapsed (s)"] -> w70
              frame False {
              }
              frame True {
              }
            }
            n89 = global write "GlobalUI.vi" "Intensity x label"(w70) -> ()
            n90 = property on="XY Graph" class="XYGraph (strict)"("XScale.NameLbl.Text"=w70) -> ()  [unwired: 2 in, 2 out]
            n91 = property on="XY Graph 2" class="XYGraph (strict)"("XScale.NameLbl.Text"=w70) -> ()  [unwired: 2 in, 2 out]
            n92 = property on="XY Graph 3" class="XYGraph (strict)"("XScale.NameLbl.Text"=w70) -> ()  [unwired: 2 in, 2 out]
          }
          frame #2 {
            n93 = property on="Pass UI values" class="Bool (strict)"() -> ("Value"=w75:bool)  [unwired: 2 in, 2 out]
            n94 = Not(x=w75) -> (.not. x?=w76:bool)
            n95 = property on="Pass UI values" class="Bool (strict)"("Val(Sgnl)"=w76) -> ()  [unwired: 2 in, 2 out]
          }
          frame #3 {
            n96 = global write "GlobalUI.vi" "Acquire"("Acquire") -> ()
            n97 = case shown="False" "Acquire" {
              tunnel: w78 -> [w80 w82]
              frame False {
                n98 = call "GetQueue.vi"("Microscope in"=w80) -> ("Microscope events"=w79:refnum<queue>, "Microscope out"=w81:refnum<class "Microscope.lvclass">)  [unwired: 8 in, 1 out]
                n99 = Flush Queue(queue=w79) -> ()  [unwired: 1 in, 3 out]
                n100 = call "StartAcquire.vi"("Microscope in"=w81) -> ()  [unwired: 9 in, 2 out]
              }
              frame True {
                n101 = call "StartAcquire.vi"("Microscope in"=w82) -> ()  [unwired: 9 in, 2 out]
              }
            }
          }
        }
      }
      event Mouse Down {
        n102 = event-data() -> ()  [unwired: 1 in, 5 out]
        n103 = property on="Pass UI values" class="Bool (strict)"() -> ("Value"=w84:bool)  [unwired: 2 in, 2 out]
        n104 = Not(x=w84) -> (.not. x?=w85:bool)
        n105 = property on="Pass UI values" class="Bool (strict)"("Val(Sgnl)"=w85) -> ()  [unwired: 2 in, 2 out]
      }
      event Mouse Down? {
        n106 = event-data() -> ("Button"=w86:u16)  [unwired: 1 in, 6 out]
        n107 = case shown="2" w86 {
          frame 0, Default {
          }
          frame 2 {
            n108 = property on="XY Graph" class="XYGraph (strict)"() -> ("XScale.Minimum"=w93:dbl, "XScale.Maximum"=w92:dbl, "YScale.Minimum"=w91:dbl, "YScale.Maximum"=w88:dbl)  [unwired: 2 in, 2 out]
            n109 = call "getCenter.vi"("ymax"=w88, "ymin"=w91, "xmax"=w92, "xmin"=w93) -> ("y"=w90:dbl, "x"=w89:dbl)  [unwired: 6 in]
            n110 = property on="XY Graph" class="XYGraph (strict)"("Cursor.Cursor X"=w89, "Cursor.Cursor Y"=w90) -> ()  [unwired: 2 in, 2 out]
          }
        }
        n111 = event-data() -> ()  [unwired: 2 in, 1 out]
      }
      event "CH1", "CH2", "CH3": Mouse Down? {
        n112 = event-data() -> ("Button"=w94:u16)  [unwired: 1 in, 6 out]
        n113 = case shown="2" w94 {
          frame 0, Default {
          }
          frame 2 {
            n114 = property on="CH1" class="IntGraph (strict)"() -> ("XScale.Minimum"=w101:dbl, "XScale.Maximum"=w100:dbl, "YScale.Minimum"=w99:dbl, "YScale.Maximum"=w98:dbl)  [unwired: 2 in, 2 out]
            n115 = call "getCenter.vi"("ymax"=w98, "ymin"=w99, "xmax"=w100, "xmin"=w101) -> ("y"=w96:dbl, "x"=w97:dbl)  [unwired: 6 in]
            n116 = property on="CH1" class="IntGraph (strict)"("Cursor.Cursor X"=w97, "Cursor.Cursor Y"=w96) -> ()  [unwired: 2 in, 2 out]
            n117 = property on="CH3" class="IntGraph (strict)"("Cursor.Cursor X"=w97, "Cursor.Cursor Y"=w96) -> ()  [unwired: 2 in, 2 out]
            n118 = property on="CH2" class="IntGraph (strict)"("Cursor.Cursor X"=w97, "Cursor.Cursor Y"=w96) -> ()  [unwired: 2 in, 2 out]
          }
        }
        n119 = event-data() -> ()  [unwired: 5 in, 1 out]
      }
      event Mouse Down? {
        n120 = event-data() -> ("Button"=w102:u16)  [unwired: 1 in, 6 out]
        n121 = case shown="2" w102 {
          frame 0, Default {
          }
          frame 2 {
            n122 = property on="XY Graph 2" class="XYGraph (strict)"() -> ("XScale.Minimum"=w109:dbl, "XScale.Maximum"=w108:dbl, "YScale.Minimum"=w107:dbl, "YScale.Maximum"=w104:dbl)  [unwired: 2 in, 2 out]
            n123 = call "getCenter.vi"("ymax"=w104, "ymin"=w107, "xmax"=w108, "xmin"=w109) -> ("y"=w106:dbl, "x"=w105:dbl)  [unwired: 6 in]
            n124 = property on="XY Graph 2" class="XYGraph (strict)"("Cursor.Cursor X"=w105, "Cursor.Cursor Y"=w106) -> ()  [unwired: 2 in, 2 out]
          }
        }
        n125 = event-data() -> ()  [unwired: 2 in, 1 out]
      }
      event Mouse Down? {
        n126 = event-data() -> ("Button"=w110:u16)  [unwired: 1 in, 6 out]
        n127 = case shown="2" w110 {
          frame 0, Default {
          }
          frame 2 {
            n128 = property on="XY Graph 3" class="XYGraph (strict)"() -> ("XScale.Minimum"=w117:dbl, "XScale.Maximum"=w116:dbl, "YScale.Minimum"=w115:dbl, "YScale.Maximum"=w112:dbl)  [unwired: 2 in, 2 out]
            n129 = call "getCenter.vi"("ymax"=w112, "ymin"=w115, "xmax"=w116, "xmin"=w117) -> ("y"=w114:dbl, "x"=w113:dbl)  [unwired: 6 in]
            n130 = property on="XY Graph 3" class="XYGraph (strict)"("Cursor.Cursor X"=w113, "Cursor.Cursor Y"=w114) -> ()  [unwired: 2 in, 2 out]
          }
        }
        n131 = event-data() -> ()  [unwired: 2 in, 1 out]
      }
      event "SpeedMode", "NormalMode", "Hi-Res Mode": Value Change {
        n132 = event-data() -> ()  [unwired: 1 in, 5 out]
        n133 = local read "Scan Parameters"() -> (w119:T4)
        n134 = stacked-sequence {
          tunnel: "SpeedMode" -> [w125 _ _ _]
          tunnel: "NormalMode" -> [_ w131 _ _]
          tunnel: "Hi-Res Mode" -> [_ _ w137 _]
          tunnel: w119 -> [w124 w130 w136 _]
          tunnel: w118 -> [_ _ _ w142]
          frame #0 {
            n135 = case shown="True" w125 {
              tunnel: w124 -> [_ w126]
              frame False {
              }
              frame True {
                n136 = in-place {
                  n137 = in-place-cluster #2(w126) -> ()  [unwired: 2 out]
                  n138 = in-place-cluster #2("scan rate (ms/line)"=4.0, "x pixels"=50) -> (w127:T4)
                }
                n139 = local write "Scan Parameters"(w127) -> ()
                n140 = global write "GlobalUI.vi" "Scan Parameters"(w127) -> ()
              }
            }
          }
          frame #1 {
            n141 = case shown="True" w131 {
              tunnel: w130 -> [_ w133]
              frame False {
              }
              frame True {
                n142 = in-place {
                  n143 = in-place-cluster #3(w133) -> ()  [unwired: 2 out]
                  n144 = in-place-cluster #3("scan rate (ms/line)"=4.0, "x pixels"=200) -> (w132:T4)
                }
                n145 = local write "Scan Parameters"(w132) -> ()
                n146 = global write "GlobalUI.vi" "Scan Parameters"(w132) -> ()
              }
            }
          }
          frame #2 {
            n147 = case shown="True" w137 {
              tunnel: w136 -> [_ w138]
              frame False {
              }
              frame True {
                n148 = in-place {
                  n149 = in-place-cluster #4(w138) -> ()  [unwired: 2 out]
                  n150 = in-place-cluster #4("scan rate (ms/line)"=20.0, "x pixels"=512) -> (w139:T4)
                }
                n151 = global write "GlobalUI.vi" "Scan Parameters"(w139) -> ()
                n152 = local write "Scan Parameters"(w139) -> ()
              }
            }
          }
          frame #3 {
            n153 = global read "GlobalUI.vi" "Acquire"() -> (w143:bool)
            n154 = case shown="True" w143 {
              tunnel: w142 -> [_ w144]
              frame False {
              }
              frame True {
                n155 = stacked-sequence {
                  tunnel: w144 -> [_ _ w147]
                  frame #0 {
                    n156 = global write "GlobalUI.vi" "Acquire"(FALSE ("Stage Acquire")) -> ()
                  }
                  frame #1 {
                    n157 = Wait (ms)(milliseconds to wait=u32 0) -> ()  [unwired: 1 out]
                  }
                  frame #2 {
                    n158 = call "FullRestartAcquire.vi"("Microscope in"=w147) -> ()  [unwired: 9 in, 2 out]
                  }
                }
              }
            }
          }
        }
      }
      event "right", "left", "up", "down", "center": Value Change {
        n159 = event-data() -> ()  [unwired: 1 in, 5 out]
        n160 = stacked-sequence {
          tunnel: "right" -> [_ _ _ w174 _ _ _ _ _ _]
          tunnel: "up" -> [_ _ _ _ w183 _ _ _ _ _]
          tunnel: "down" -> [_ _ _ _ _ w192 _ _ _ _]
          tunnel: "left" -> [_ _ w165 _ _ _ _ _ _ _]
          tunnel: "center" -> [_ w159 _ _ _ _ _ _ _ _]
          tunnel: "dV" -> [_ _ w164 w173 w182 w191 _ _ _ _]
          tunnel: w148 -> [_ _ _ _ _ _ _ _ _ w203]
          frame #0 {
            n161 = local read "Scan Parameters"() -> (w157:T4)
            n162 = in-place {
              n163 = in-place-cluster #5(w157) -> ()  [unwired: 1 out]
              n164 = local read "Zoom"() -> (w158:dbl)
              n165 = global write "GlobalUI.vi" "Zoom"(w158) -> ()
              n166 = in-place-cluster #5("Zoom"=w158) -> (w156:T4)
            }
            n167 = global write "GlobalUI.vi" "Scan Parameters"(w156) -> ()
            n168 = local write "Scan Parameters"(w156) -> ()
          }
          frame #1 {
            # "center"
            n169 = case shown="True" w159 {
              frame False {
              }
              frame True {
                n170 = local read "Scan Parameters"() -> (w161:T4)
                n171 = in-place {
                  w162 = 8.0 ("x voltage max")
                  w163 = -8.0 ("x voltage min")
                  n172 = in-place-cluster #6(w161) -> ()  [unwired: 4 out]
                  n173 = in-place-cluster #6("x voltage min"=w163, "y voltage min"=w163, "x voltage max"=w162, "y voltage max"=w162) -> (w160:T4)
                }
                n174 = global write "GlobalUI.vi" "Scan Parameters"(w160) -> ()
                n175 = local write "Scan Parameters"(w160) -> ()
              }
            }
          }
          frame #2 {
            n176 = case shown="True" w165 {
              tunnel: w164 -> [_ w167]
              frame False {
              }
              frame True {
                # "left"
                n177 = local read "Scan Parameters"() -> (w172:T4)
                n178 = Unbundle By Name(w172) -> ("x voltage min"=w171:dbl, "x voltage max"=w170:dbl)
                n179 = formula code="vmin -= dv;\nvmax -= dv;"("vmin"=w171, "vmax"=w170, "dv"=w167) -> ("vmin"=w169:dbl, "vmax"=w168:dbl)
                n180 = Bundle By Name(cluster=w172, "x voltage min"=w169, "x voltage max"=w168) -> (w166:T4)
                n181 = local write "Scan Parameters"(w166) -> ()
                n182 = global write "GlobalUI.vi" "Scan Parameters"(w166) -> ()
              }
            }
          }
          frame #3 {
            n183 = case shown="True" w174 {
              tunnel: w173 -> [_ w176]
              frame False {
              }
              frame True {
                # "right"
                n184 = local read "Scan Parameters"() -> (w181:T4)
                n185 = Unbundle By Name(w181) -> ("x voltage min"=w180:dbl, "x voltage max"=w179:dbl)
                n186 = formula code="vmin += dv;\nvmax += dv;"("vmin"=w180, "vmax"=w179, "dv"=w176) -> ("vmin"=w178:dbl, "vmax"=w177:dbl)
                n187 = Bundle By Name(cluster=w181, "x voltage min"=w178, "x voltage max"=w177) -> (w175:T4)
                n188 = local write "Scan Parameters"(w175) -> ()
                n189 = global write "GlobalUI.vi" "Scan Parameters"(w175) -> ()
              }
            }
          }
          frame #4 {
            # "up"
            n190 = case shown="True" w183 {
              tunnel: w182 -> [_ w185]
              frame False {
              }
              frame True {
                n191 = local read "Scan Parameters"() -> (w190:T4)
                n192 = Unbundle By Name(w190) -> ("y voltage min"=w189:dbl, "y voltage max"=w188:dbl)
                n193 = formula code="vmin += dv;\nvmax += dv;"("vmin"=w189, "vmax"=w188, "dv"=w185) -> ("vmin"=w187:dbl, "vmax"=w186:dbl)
                n194 = Bundle By Name(cluster=w190, "y voltage min"=w187, "y voltage max"=w186) -> (w184:T4)
                n195 = local write "Scan Parameters"(w184) -> ()
                n196 = global write "GlobalUI.vi" "Scan Parameters"(w184) -> ()
              }
            }
          }
          frame #5 {
            # "down"
            n197 = case shown="True" w192 {
              tunnel: w191 -> [_ w194]
              frame False {
              }
              frame True {
                n198 = local read "Scan Parameters"() -> (w199:T4)
                n199 = Unbundle By Name(w199) -> ("y voltage min"=w198:dbl, "y voltage max"=w197:dbl)
                n200 = formula code="vmin -= dv;\nvmax -= dv;"("vmin"=w198, "vmax"=w197, "dv"=w194) -> ("vmin"=w196:dbl, "vmax"=w195:dbl)
                n201 = Bundle By Name(cluster=w199, "y voltage min"=w196, "y voltage max"=w195) -> (w193:T4)
                n202 = local write "Scan Parameters"(w193) -> ()
                n203 = global write "GlobalUI.vi" "Scan Parameters"(w193) -> ()
              }
            }
          }
          frame #6 {
            n204 = global write "GlobalUI.vi" "Acquire"(FALSE ("softstop")) -> ()
          }
          frame #7 {
            n205 = Wait (ms)(milliseconds to wait=u32 100) -> ()  [unwired: 1 out]
          }
          frame #8 {
            n206 = global write "GlobalUI.vi" "Acquire"(TRUE ("softstop")) -> ()
          }
          frame #9 {
            n207 = local read "Acquire"() -> (w204:bool)
            n208 = case shown="True" w204 {
              tunnel: w203 -> [_ w205]
              frame False {
              }
              frame True {
                n209 = call "FullRestartAcquire.vi"("Microscope in"=w205) -> ()  [unwired: 9 in, 2 out]
              }
            }
          }
        }
      }
      event "Zoom": Value Change {
        n210 = event-data() -> ()  [unwired: 1 in, 6 out]
        n211 = flat-sequence {
          tunnel: w207 -> [w211]
          tunnel: [w211] -> w206
          tunnel: w206 -> [w214]
          frame #0 {
            n212 = local read "Scan Parameters"() -> (w210:T4)
            n213 = in-place {
              n214 = in-place-cluster #7(w210) -> ()  [unwired: 1 out]
              n215 = local read "Zoom"() -> (w212:dbl)
              n216 = global write "GlobalUI.vi" "Zoom"(w212) -> ()
              n217 = in-place-cluster #7("Zoom"=w212) -> (w209:T4)
            }
            n218 = global write "GlobalUI.vi" "Scan Parameters"(w209) -> ()
            n219 = local write "Scan Parameters"(w209) -> ()
          }
          frame #1 {
            n220 = property on="Acquire" class="Bool (strict)"() -> ("Value"=w213:bool)  [unwired: 2 in, 2 out]
            n221 = global write "GlobalUI.vi" "Acquire"(w213) -> ()
            n222 = case shown="True" w213 {
              tunnel: w214 -> [w215 w216]
              frame False {
                n223 = call "SetParam.vi"("Microscope in"=w215) -> ()  [unwired: 9 in, 2 out]
              }
              frame True {
                n224 = stacked-sequence {
                  tunnel: w216 -> [_ _ _ w221]
                  frame #0 {
                    n225 = global write "GlobalUI.vi" "Acquire"(FALSE ("softstop")) -> ()
                  }
                  frame #1 {
                    n226 = Wait (ms)(milliseconds to wait=u32 100) -> ()  [unwired: 1 out]
                  }
                  frame #2 {
                    n227 = global write "GlobalUI.vi" "Acquire"(TRUE ("softstop")) -> ()
                  }
                  frame #3 {
                    n228 = call "GetQueue.vi"("Microscope in"=w221) -> ("Microscope events"=w220:refnum<queue>)  [unwired: 8 in, 2 out]
                    n229 = call-poly "sequences.vi"("Queue in"=w220) -> ()  [unwired: 9 in, 2 out]
                  }
                }
              }
            }
          }
        }
      }
      event "Preset PMT1", "Preset PMT2", "Preset PMT3": Value Change {
        w223 = "%.2f" ("format string")
        n230 = event-data() -> ()  [unwired: 1 in, 6 out]
        n231 = local read "Preset PMT2"() -> (w225:dbl)
        n232 = local read "Preset PMT1"() -> (w226:dbl)
        n233 = local read "Preset PMT3"() -> (w224:dbl)
        n234 = Format Into String(format string=w223, w225) -> (resulting string=w228:string)  [unwired: 2 in, 1 out]
        n235 = Format Into String(format string=w223, w226) -> (resulting string=w229:string)  [unwired: 2 in, 1 out]
        n236 = Format Into String(format string=w223, w224) -> (resulting string=w222:string)  [unwired: 2 in, 1 out]
        n237 = property on="preset2" class="Bool"("BoolText.Text"=w228) -> ()  [unwired: 2 in, 2 out]
        n238 = property on="preset1" class="Bool"("BoolText.Text"=w229) -> ()  [unwired: 2 in, 2 out]
        n239 = property on="preset3" class="Bool"("BoolText.Text"=w222) -> ()  [unwired: 2 in, 2 out]
      }
      event "jet", "grayscale": Value Change {
        n240 = event-data() -> ()  [unwired: 1 in, 6 out]
        n241 = stacked-sequence {
          tunnel: "jet" -> [w233 _]
          tunnel: "grayscale" -> [_ w267]
          frame #0 {
            n242 = case shown="True" w233 {
              frame False {
              }
              frame True {
                n243 = stacked-sequence {
                  frame #0 {
                    n244 = property on="CH1" class="IntGraph (strict)"() -> ("ZScale.Maximum"=w235:dbl)  [unwired: 2 in, 2 out]
                    n245 = formula code="float64 midv,minv;\nminv = 0;\nmidv = (maxv + minv)/ 2;"("maxv"=w235) -> ("maxv"=w241:dbl, "midv"=w239:dbl, "minv"=w236:dbl)
                    n246 = Bundle("maxv"=w241, u32 16711680) -> (w244:cluster{"maxv":dbl, u32})  [unwired: 1 in]
                    n247 = Bundle(w239, u32 65280) -> (w243:cluster{dbl, u32})  [unwired: 1 in]
                    n248 = Bundle(w236, u32 16860) -> (w242:cluster{dbl, u32})  [unwired: 1 in]
                    n249 = Build Array(w244, w243, w242) -> (w234:cluster{"maxv":dbl, u32}[])
                    n250 = property on="CH1" class="IntGraph (strict)"("ZScale.MarkerVals[]"=w234) -> ()  [unwired: 2 in, 2 out]
                  }
                  frame #1 {
                    n251 = property on="CH2" class="IntGraph (strict)"() -> ("ZScale.Maximum"=w246:dbl)  [unwired: 2 in, 2 out]
                    n252 = formula code="float64 midv,minv;\nminv = 0;\nmidv = (maxv + minv)/ 2;"("maxv"=w246) -> ("maxv"=w252:dbl, "midv"=w250:dbl, "minv"=w247:dbl)
                    n253 = Bundle("maxv"=w252, u32 16711680) -> (w255:cluster{"maxv":dbl, u32})  [unwired: 1 in]
                    n254 = Bundle(w250, u32 65280) -> (w254:cluster{dbl, u32})  [unwired: 1 in]
                    n255 = Bundle(w247, u32 16860) -> (w253:cluster{dbl, u32})  [unwired: 1 in]
                    n256 = Build Array(w255, w254, w253) -> (w245:cluster{"maxv":dbl, u32}[])
                    n257 = property on="CH2" class="IntGraph (strict)"("ZScale.MarkerVals[]"=w245) -> ()  [unwired: 2 in, 2 out]
                  }
                  frame #2 {
                    n258 = property on="CH3" class="IntGraph (strict)"() -> ("ZScale.Maximum"=w257:dbl)  [unwired: 2 in, 2 out]
                    n259 = formula code="float64 midv,minv;\nminv = 0;\nmidv = (maxv + minv)/ 2;"("maxv"=w257) -> ("maxv"=w263:dbl, "midv"=w261:dbl, "minv"=w258:dbl)
                    n260 = Bundle("maxv"=w263, u32 16711680) -> (w266:cluster{"maxv":dbl, u32})  [unwired: 1 in]
                    n261 = Bundle(w261, u32 65280) -> (w265:cluster{dbl, u32})  [unwired: 1 in]
                    n262 = Bundle(w258, u32 16860) -> (w264:cluster{dbl, u32})  [unwired: 1 in]
                    n263 = Build Array(w266, w265, w264) -> (w256:cluster{"maxv":dbl, u32}[])
                    n264 = property on="CH3" class="IntGraph (strict)"("ZScale.MarkerVals[]"=w256) -> ()  [unwired: 2 in, 2 out]
                  }
                }
              }
            }
          }
          frame #1 {
            n265 = case shown="True" w267 {
              frame False {
              }
              frame True {
                n266 = stacked-sequence {
                  frame #0 {
                    n267 = property on="CH1" class="IntGraph (strict)"() -> ("ZScale.Maximum"=w271:dbl)  [unwired: 2 in, 2 out]
                    n268 = formula code="float64 midv,minv;\nminv = 0;\nmidv = (maxv + minv)/ 2;"("maxv"=w271) -> ("maxv"=w275:dbl, "midv"=w274:dbl, "minv"=w272:dbl)
                    n269 = Bundle("maxv"=w275, u32 16777215) -> (w278:cluster{"maxv":dbl, u32})  [unwired: 1 in]
                    n270 = Bundle(w274, u32 8355711) -> (w277:cluster{dbl, u32})  [unwired: 1 in]
                    n271 = Bundle(w272, u32 0) -> (w276:cluster{dbl, u32})  [unwired: 1 in]
                    n272 = Build Array(w278, w277, w276) -> (w268:cluster{"maxv":dbl, u32}[])
                    n273 = property on="CH1" class="IntGraph (strict)"("ZScale.MarkerVals[]"=w268) -> ()  [unwired: 2 in, 2 out]
                  }
                  frame #1 {
                    n274 = property on="CH2" class="IntGraph (strict)"() -> ("ZScale.Maximum"=w282:dbl)  [unwired: 2 in, 2 out]
                    n275 = formula code="float64 midv,minv;\nminv = 0;\nmidv = (maxv + minv)/ 2;"("maxv"=w282) -> ("maxv"=w286:dbl, "midv"=w285:dbl, "minv"=w283:dbl)
                    n276 = Bundle("maxv"=w286, u32 16777215) -> (w289:cluster{"maxv":dbl, u32})  [unwired: 1 in]
                    n277 = Bundle(w285, u32 8355711) -> (w288:cluster{dbl, u32})  [unwired: 1 in]
                    n278 = Bundle(w283, u32 0) -> (w287:cluster{dbl, u32})  [unwired: 1 in]
                    n279 = Build Array(w289, w288, w287) -> (w279:cluster{"maxv":dbl, u32}[])
                    n280 = property on="CH2" class="IntGraph (strict)"("ZScale.MarkerVals[]"=w279) -> ()  [unwired: 2 in, 2 out]
                  }
                  frame #2 {
                    n281 = property on="CH3" class="IntGraph (strict)"() -> ("ZScale.Maximum"=w293:dbl)  [unwired: 2 in, 2 out]
                    n282 = formula code="float64 midv,minv;\nminv = 0;\nmidv = (maxv + minv)/ 2;"("maxv"=w293) -> ("maxv"=w297:dbl, "midv"=w296:dbl, "minv"=w294:dbl)
                    n283 = Bundle("maxv"=w297, u32 16777215) -> (w300:cluster{"maxv":dbl, u32})  [unwired: 1 in]
                    n284 = Bundle(w296, u32 8355711) -> (w299:cluster{dbl, u32})  [unwired: 1 in]
                    n285 = Bundle(w294, u32 0) -> (w298:cluster{dbl, u32})  [unwired: 1 in]
                    n286 = Build Array(w300, w299, w298) -> (w290:cluster{"maxv":dbl, u32}[])
                    n287 = property on="CH3" class="IntGraph (strict)"("ZScale.MarkerVals[]"=w290) -> ()  [unwired: 2 in, 2 out]
                  }
                }
              }
            }
          }
        }
      }
      event "min1", "max1", "max2", "min2", "max3", "min3": Value Change {
        n288 = event-data() -> ()  [unwired: 1 in, 6 out]
        n289 = property on="Pass UI values" class="Bool (strict)"() -> ("Value"=w302:bool)  [unwired: 2 in, 2 out]
        n290 = Not(x=w302) -> (.not. x?=w301:bool)
        n291 = property on="Pass UI values" class="Bool (strict)"("Val(Sgnl)"=w301) -> ()  [unwired: 2 in, 2 out]
      }
      event "autoscale1": Value Change {
        w312 = 0.0 ("y")
        n292 = event-data() -> ()  [unwired: 1 in, 6 out]
        n293 = local read "CH1"() -> (w314:dbl[][])
        n294 = Array Max & Min(array=w314) -> (max value=w304:dbl, min value=w310:dbl)  [unwired: 2 out]
        n295 = Greater?(x=w310, y=w312) -> (0:w311:bool)
        n296 = disable-structure shown="Enabled" {
          disable-tunnel: [w319 w320] -> w305
          disable-tunnel: w304 -> [w315 w320]
          frame Disabled {
            w316 = 250.0 ("y")
            n297 = Divide(x=w315, y=w316) -> (x/y=w318:dbl)
            n298 = Round Toward +Infinity(x=w318) -> (ceil(x): smallest int >= x=w317:dbl)
            n299 = Multiply(x=w317, y=w316) -> (x*y=w319:dbl)
          }
          frame Enabled {
          }
        }
        n300 = Select(t=w312, s=w311, f=w310) -> (s? t:f=w309:dbl)
        n301 = local write "min1"(w309) -> ()
        n302 = property on="CH1" class="IntGraph (strict)"("ZScale.Minimum"=w309) -> (error out=w306:errorcluster)  [unwired: 2 in, 1 out]
        n303 = property on="Pass UI values" class="Bool (strict)"(error in=w306) -> ("Value"=w308:bool)  [unwired: 1 in, 2 out]
        n304 = Not(x=w308) -> (.not. x?=w307:bool)
        n305 = local write "max1"(w305) -> ()
        n306 = property on="CH1" class="IntGraph (strict)"("ZScale.Maximum"=w305) -> ()  [unwired: 2 in, 2 out]
        n307 = property on="Pass UI values" class="Bool (strict)"("Val(Sgnl)"=w307) -> ()  [unwired: 2 in, 2 out]
      }
      event "autoscale2": Value Change {
        w328 = 0.0 ("y")
        n308 = event-data() -> ()  [unwired: 1 in, 6 out]
        n309 = local read "CH2"() -> (w331:dbl[][])
        n310 = Array Max & Min(array=w331) -> (max value=w321:dbl, min value=w327:dbl)  [unwired: 2 out]
        n311 = disable-structure shown="Enabled" {
          disable-tunnel: [w336 w337] -> w322
          disable-tunnel: w321 -> [w332 w337]
          frame Disabled {
            w333 = 250.0 ("y")
            n312 = Divide(x=w332, y=w333) -> (x/y=w335:dbl)
            n313 = Round Toward +Infinity(x=w335) -> (ceil(x): smallest int >= x=w334:dbl)
            n314 = Multiply(x=w334, y=w333) -> (x*y=w336:dbl)
          }
          frame Enabled {
          }
        }
        n315 = Greater?(x=w327, y=w328) -> (0:w329:bool)
        n316 = Select(t=w328, s=w329, f=w327) -> (s? t:f=w326:dbl)
        n317 = local write "max2"(w322) -> ()
        n318 = local write "min2"(w326) -> ()
        n319 = property on="CH2" class="IntGraph (strict)"("ZScale.Maximum"=w322) -> ()  [unwired: 2 in, 2 out]
        n320 = property on="CH2" class="IntGraph (strict)"("ZScale.Minimum"=w326) -> (error out=w323:errorcluster)  [unwired: 2 in, 1 out]
        n321 = property on="Pass UI values" class="Bool (strict)"(error in=w323) -> ("Value"=w325:bool)  [unwired: 1 in, 2 out]
        n322 = Not(x=w325) -> (.not. x?=w324:bool)
        n323 = property on="Pass UI values" class="Bool (strict)"("Val(Sgnl)"=w324) -> ()  [unwired: 2 in, 2 out]
      }
      event "autoscale3": Value Change {
        n324 = event-data() -> ()  [unwired: 1 in, 6 out]
        n325 = local read "CH3"() -> (w348:dbl[][])
        n326 = Array Max & Min(array=w348) -> (max value=w340:dbl, min value=w338:dbl)  [unwired: 2 out]
        n327 = Greater?(x=w338, y=0.0) -> (0:w346:bool)
        n328 = disable-structure shown="Enabled" {
          disable-tunnel: [w353 w354] -> w344
          disable-tunnel: w340 -> [w352 w354]
          frame Disabled {
            w349 = 250.0 ("y")
            n329 = Divide(x=w352, y=w349) -> (x/y=w351:dbl)
            n330 = Round Toward +Infinity(x=w351) -> (ceil(x): smallest int >= x=w350:dbl)
            n331 = Multiply(x=w350, y=w349) -> (x*y=w353:dbl)
          }
          frame Enabled {
          }
        }
        n332 = Select(t=w338, s=w346, f=w338) -> (s? t:f=w345:dbl)
        n333 = local write "min3"(w345) -> ()
        n334 = property on="CH3" class="IntGraph (strict)"("ZScale.Minimum"=w345) -> (error out=w341:errorcluster)  [unwired: 2 in, 1 out]
        n335 = property on="Pass UI values" class="Bool (strict)"(error in=w341) -> ("Value"=w343:bool)  [unwired: 1 in, 2 out]
        n336 = Not(x=w343) -> (.not. x?=w342:bool)
        n337 = local write "max3"(w344) -> ()
        n338 = property on="CH3" class="IntGraph (strict)"("ZScale.Maximum"=w344) -> ()  [unwired: 2 in, 2 out]
        n339 = property on="Pass UI values" class="Bool (strict)"("Val(Sgnl)"=w342) -> ()  [unwired: 2 in, 2 out]
      }
      event "MoveStageTarget": Value Change {
        n340 = event-data() -> ()  [unwired: 1 in, 6 out]
        n341 = property on="Pass UI values" class="Bool (strict)"() -> ("Value"=w357:bool)  [unwired: 2 in, 2 out]
        n342 = Not(x=w357) -> (.not. x?=w356:bool)
        n343 = global read "GlobalUI.vi" "Acquire"() -> (w359:bool)
        n344 = property on="Pass UI values" class="Bool (strict)"("Val(Sgnl)"=w356) -> (error out=w355:errorcluster)  [unwired: 2 in, 1 out]
        n345 = case shown="True" w359 {
          tunnel: w358 -> [w363 w374]
          tunnel: w355 -> [w362 w373]
          frame False {
            n346 = flat-sequence {
              tunnel: [w367] -> w364
              tunnel: w363 -> [w367]
              tunnel: w362 -> [w366]
              tunnel: [w366] -> w361
              tunnel: w364 -> [w370]
              tunnel: w361 -> [w369]
              frame #0 {
                n347 = Wait (ms)(milliseconds to wait=u32 10) -> ()  [unwired: 1 out]
              }
              frame #1 {
                n348 = call "Command.vi"("error in (no error)"=w369, "Stage events"=StageEvent."stage.MoveTo1" ("Stage element"), "Microscope in"=w370) -> ()  [unwired: 7 in, 2 out]
              }
            }
          }
          frame True {
            n349 = flat-sequence {
              tunnel: w374 -> [w376]
              tunnel: [w376] -> w372
              tunnel: w373 -> [w375]
              tunnel: [w375] -> w371
              tunnel: w372 -> [w380]
              tunnel: w371 -> [w379]
              frame #0 {
                n350 = Wait (ms)(milliseconds to wait=u32 10) -> ()  [unwired: 1 out]
              }
              frame #1 {
                n351 = call "Command.vi"("error in (no error)"=w379, "Stage events"=StageEvent."stage.MoveTo1" ("Enum"), "Microscope in"=w380) -> ()  [unwired: 7 in, 2 out]
              }
            }
          }
        }
      }
      event "MoveStageTarget 2": Value Change {
        n352 = event-data() -> ()  [unwired: 1 in, 6 out]
        n353 = property on="Pass UI values" class="Bool (strict)"() -> ("Value"=w383:bool)  [unwired: 2 in, 2 out]
        n354 = Not(x=w383) -> (.not. x?=w382:bool)
        n355 = global read "GlobalUI.vi" "Acquire"() -> (w385:bool)
        n356 = property on="Pass UI values" class="Bool (strict)"("Val(Sgnl)"=w382) -> (error out=w381:errorcluster)  [unwired: 2 in, 1 out]
        n357 = case shown="True" w385 {
          tunnel: w384 -> [w390 w400]
          tunnel: w381 -> [w389 w399]
          frame False {
            n358 = flat-sequence {
              tunnel: w389 -> [w392]
              tunnel: w390 -> [w393]
              tunnel: [w393] -> w388
              tunnel: [w392] -> w387
              tunnel: w388 -> [w396]
              tunnel: w387 -> [w395]
              frame #0 {
                n359 = Wait (ms)(milliseconds to wait=u32 10) -> ()  [unwired: 1 out]
              }
              frame #1 {
                n360 = call "Command.vi"("error in (no error)"=w395, "Stage events"=StageEvent."stage.MoveTo2" ("Stage element"), "Microscope in"=w396) -> ()  [unwired: 7 in, 2 out]
              }
            }
          }
          frame True {
            n361 = flat-sequence {
              tunnel: w399 -> [w402]
              tunnel: w400 -> [w403]
              tunnel: [w403] -> w398
              tunnel: [w402] -> w397
              tunnel: w398 -> [w406]
              tunnel: w397 -> [w405]
              frame #0 {
                n362 = Wait (ms)(milliseconds to wait=u32 10) -> ()  [unwired: 1 out]
              }
              frame #1 {
                n363 = call "Command.vi"("error in (no error)"=w405, "Stage events"=StageEvent."stage.MoveTo2" ("Stage element"), "Microscope in"=w406) -> ()  [unwired: 7 in, 2 out]
              }
            }
          }
        }
      }
      event "MoveStageTarget 3": Value Change {
        n364 = event-data() -> ()  [unwired: 1 in, 6 out]
        n365 = property on="Pass UI values" class="Bool (strict)"() -> ("Value"=w409:bool)  [unwired: 2 in, 2 out]
        n366 = Not(x=w409) -> (.not. x?=w408:bool)
        n367 = global read "GlobalUI.vi" "Acquire"() -> (w411:bool)
        n368 = property on="Pass UI values" class="Bool (strict)"("Val(Sgnl)"=w408) -> (error out=w407:errorcluster)  [unwired: 2 in, 1 out]
        n369 = case shown="True" w411 {
          tunnel: w410 -> [w414 w424]
          tunnel: w407 -> [w413 w423]
          frame False {
            n370 = flat-sequence {
              tunnel: [w419] -> w416
              tunnel: w414 -> [w419]
              tunnel: w413 -> [w418]
              tunnel: [w418] -> w415
              tunnel: w416 -> [w422]
              tunnel: w415 -> [w421]
              frame #0 {
                n371 = Wait (ms)(milliseconds to wait=u32 10) -> ()  [unwired: 1 out]
              }
              frame #1 {
                n372 = call "Command.vi"("error in (no error)"=w421, "Stage events"=StageEvent."stage.MoveTo3" ("Stage element"), "Microscope in"=w422) -> ()  [unwired: 7 in, 2 out]
              }
            }
          }
          frame True {
            n373 = flat-sequence {
              tunnel: [w429] -> w426
              tunnel: w424 -> [w429]
              tunnel: w423 -> [w428]
              tunnel: [w428] -> w425
              tunnel: w426 -> [w432]
              tunnel: w425 -> [w431]
              frame #0 {
                n374 = Wait (ms)(milliseconds to wait=u32 10) -> ()  [unwired: 1 out]
              }
              frame #1 {
                n375 = call "Command.vi"("error in (no error)"=w431, "Stage events"=StageEvent."stage.MoveTo3" ("Stage element"), "Microscope in"=w432) -> ()  [unwired: 7 in, 2 out]
              }
            }
          }
        }
      }
      event "SpecWiz": Value Change {
        n376 = event-data() -> ()  [unwired: 1 in, 6 out]
        n377 = case shown="False" "SpecWiz" {
          tunnel: [w436 w443] -> _
          frame True {
            w437 = FALSE ("Wait Until Done")
            n378 = vi-ref "SW-Microscoper.vi"() -> (w442:refnum<vi>)
            n379 = invoke class="VI" method="FP.Open"(reference=w442, "Activate"=TRUE ("Activate?"), "State"=T8."Standard") -> (reference out=w439:refnum<vi>, error out=w438:errorcluster)  [unwired: 2 in, 3 out]
            n380 = invoke class="VI" method="Run VI"(reference=w439, error in=w438, "Wait until done"=w437, "Auto Dispose Ref"=w437) -> (error out=w436:errorcluster)  [unwired: 1 in, 4 out]
            n381 = property on="SpecWiz" class="Bool (strict)"("Value"=FALSE ("SW")) -> ()  [unwired: 2 in, 2 out]
          }
          frame False {
            n382 = disable-structure shown="Enabled" {
              disable-tunnel: [w445 w452] -> w443
              frame Enabled {
                n383 = vi-ref "SW-Microscoper.vi"() -> (w451:refnum<vi>)
                n384 = invoke class="VI" method="FP.Open"(reference=w451, "Activate"=TRUE ("Activate?"), "State"=T8."Standard") -> (reference out=w448:refnum<vi>, error out=w447:errorcluster)  [unwired: 2 in, 3 out]
                n385 = invoke class="VI" method="Run VI"(reference=w448, error in=w447, "Wait until done"=FALSE ("Wait Until Done"), "Auto Dispose Ref"=TRUE ("Auto Dispose Reference")) -> (error out=w445:errorcluster)  [unwired: 1 in, 4 out]
              }
              frame Disabled {
                n386 = vi-ref "SW-Microscoper.vi"() -> (w453:refnum<vi>)
                n387 = invoke class="VI" method="FP.Close"(reference=w453) -> (error out=w452:errorcluster)  [unwired: 2 in, 2 out]
              }
            }
          }
        }
      }
      event "Close": Value Change {
        n388 = event-data() -> ()  [unwired: 1 in, 6 out]
        n389 = case shown="True" "Close" {
          tunnel: w454 -> [w458 _]
          frame True {
            n390 = call "Command.vi"("Microscope events"=MicroscopeEvent."M.ClearImageData", "Microscope in"=w458) -> ()  [unwired: 8 in, 2 out]
          }
          frame False {
          }
        }
      }
      event "Rot": Value Change {
        n391 = event-data() -> ()  [unwired: 1 in, 6 out]
        n392 = disable-structure shown="Disabled" {
          disable-tunnel: [w461 _] -> _
          frame Disabled {
            n393 = vi-ref "RotationApplication.vi"() -> (w462:refnum<vi>)
            n394 = invoke class="VI" method="FP.Close"(reference=w462) -> (error out=w461:errorcluster)  [unwired: 2 in, 2 out]
          }
          frame Enabled {
          }
        }
        n395 = case shown="False" "Rot" {
          tunnel: [w465 w473] -> _
          frame True {
            w464 = FALSE ("Wait Until Done")
            n396 = vi-ref "RotationApplication.vi"() -> (w468:refnum<vi>)
            n397 = invoke class="VI" method="FP.Open"(reference=w468, "Activate"=TRUE ("Activate?"), "State"=T8."Standard") -> (reference out=w467:refnum<vi>, error out=w466:errorcluster)  [unwired: 2 in, 3 out]
            n398 = property on="Rot" class="Bool (strict)"("Value"=FALSE ("RM")) -> ()  [unwired: 2 in, 2 out]
            n399 = invoke class="VI" method="Run VI"(reference=w467, error in=w466, "Wait until done"=w464, "Auto Dispose Ref"=w464) -> (error out=w465:errorcluster)  [unwired: 1 in, 4 out]
          }
          frame False {
            w472 = FALSE ("Wait Until Done")
            n400 = vi-ref "RotationApplication.vi"() -> (w476:refnum<vi>)
            n401 = invoke class="VI" method="FP.Open"(reference=w476, "Activate"=TRUE ("Activate?"), "State"=T8."Standard") -> (reference out=w475:refnum<vi>, error out=w474:errorcluster)  [unwired: 2 in, 3 out]
            n402 = property on="Rot" class="Bool (strict)"("Value"=FALSE ("RM")) -> ()  [unwired: 2 in, 2 out]
            n403 = invoke class="VI" method="Run VI"(reference=w475, error in=w474, "Wait until done"=w472, "Auto Dispose Ref"=w472) -> (error out=w473:errorcluster)  [unwired: 1 in, 4 out]
          }
        }
      }
      event "preset1": Value Change {
        n404 = event-data() -> ()  [unwired: 1 in, 6 out]
        n405 = property on="Acquire" class="Bool (strict)"() -> ("Value"=w479:bool)  [unwired: 2 in, 2 out]
        n406 = case shown="False" w479 {
          tunnel: w486 -> [w493 w499]
          tunnel: [w492 w498] -> w485
          tunnel: w484 -> [_ w497]
          tunnel: w483 -> [_ w496]
          tunnel: [w487 _] -> w480
          frame True {
            n407 = property on="preset1" class="Bool"() -> ("BoolText.Text"=w494:string)  [unwired: 2 in, 2 out]
            n408 = local write "PMT1"(TRUE ("PMT2 on")) -> ()
            n409 = Fract/Exp String To Number(string=w494) -> (number=w491:dbl)  [unwired: 3 in, 1 out]
            n410 = local write "PMT1"(w491) -> ()
            n411 = local read "PMT2"() -> (w490:dbl)
            n412 = local read "PMT3"() -> (w488:dbl)
            n413 = call "MCCPMTupdate.vi"("MCCPMT in"=w493, "pmt voltage 1"=w491, "pmt voltage 2"=w490, "pmt voltage 3"=w488) -> ("MCCPMT out"=w492:refnum<class "MCCPMT.lvclass">, "error out"=w487:errorcluster)  [unwired: 10 in]
          }
          frame False {
            n414 = property on="preset1" class="Bool"() -> ("BoolText.Text"=w500:string)  [unwired: 2 in, 2 out]
            n415 = Fract/Exp String To Number(string=w500) -> (number=w495:dbl)  [unwired: 3 in, 1 out]
            n416 = local write "PMT1"(w495) -> ()
            n417 = call "MCCPMTstore.vi"("MCCPMT in"=w499, "pmt voltage 1"=w495, "pmt voltage 2"=w497, "pmt voltage 3"=w496) -> ("MCCPMT out"=w498:refnum<class "MCCPMT.lvclass">)  [unwired: 10 in, 1 out]
          }
        }
        n418 = property on="Pass UI values" class="Bool (strict)"(error in=w480) -> ("Value"=w482:bool)  [unwired: 1 in, 2 out]
        n419 = Not(x=w482) -> (.not. x?=w481:bool)
        n420 = property on="Pass UI values" class="Bool (strict)"("Val(Sgnl)"=w481) -> ()  [unwired: 2 in, 2 out]
      }
      event "preset2": Value Change {
        n421 = event-data() -> ()  [unwired: 1 in, 6 out]
        n422 = property on="Acquire" class="Bool (strict)"() -> ("Value"=w501:bool)  [unwired: 2 in, 2 out]
        n423 = case shown="True" w501 {
          tunnel: w508 -> [w514 w521]
          tunnel: [w515 w520] -> w507
          tunnel: w506 -> [w511 _]
          tunnel: w505 -> [w510 _]
          tunnel: [w509 _] -> w502
          frame False {
            n424 = property on="preset2" class="Bool"() -> ("BoolText.Text"=w513:string)  [unwired: 2 in, 2 out]
            n425 = Fract/Exp String To Number(string=w513) -> (number=w512:dbl)  [unwired: 3 in, 1 out]
            n426 = local write "PMT2"(w512) -> ()
            n427 = call "MCCPMTstore.vi"("MCCPMT in"=w514, "pmt voltage 1"=w511, "pmt voltage 2"=w512, "pmt voltage 3"=w510) -> ("MCCPMT out"=w515:refnum<class "MCCPMT.lvclass">, "error out"=w509:errorcluster)  [unwired: 10 in]
          }
          frame True {
            n428 = property on="preset2" class="Bool"() -> ("BoolText.Text"=w522:string)  [unwired: 2 in, 2 out]
            n429 = local write "PMT2"(TRUE ("PMT2 on")) -> ()
            n430 = Fract/Exp String To Number(string=w522) -> (number=w519:dbl)  [unwired: 3 in, 1 out]
            n431 = local write "PMT2"(w519) -> ()
            n432 = local read "PMT1"() -> (w518:dbl)
            n433 = local read "PMT3"() -> (w516:dbl)
            n434 = call "MCCPMTupdate.vi"("MCCPMT in"=w521, "pmt voltage 1"=w518, "pmt voltage 2"=w519, "pmt voltage 3"=w516) -> ("MCCPMT out"=w520:refnum<class "MCCPMT.lvclass">)  [unwired: 10 in, 1 out]
          }
        }
        n435 = property on="Pass UI values" class="Bool (strict)"(error in=w502) -> ("Value"=w504:bool)  [unwired: 1 in, 2 out]
        n436 = Not(x=w504) -> (.not. x?=w503:bool)
        n437 = property on="Pass UI values" class="Bool (strict)"("Val(Sgnl)"=w503) -> ()  [unwired: 2 in, 2 out]
      }
      event "preset3": Value Change {
        n438 = event-data() -> ()  [unwired: 1 in, 6 out]
        n439 = property on="Acquire" class="Bool (strict)"() -> ("Value"=w523:bool)  [unwired: 2 in, 2 out]
        n440 = case shown="True" w523 {
          tunnel: w530 -> [w535 w544]
          tunnel: [w536 w543] -> w529
          tunnel: w528 -> [w533 w538]
          tunnel: w527 -> [w532 w539]
          tunnel: [_ w537] -> w524
          frame False {
            n441 = property on="preset3" class="Bool"() -> ("BoolText.Text"=w534:string)  [unwired: 2 in, 2 out]
            n442 = Fract/Exp String To Number(string=w534) -> (number=w531:dbl)  [unwired: 3 in, 1 out]
            n443 = global write "GlobalUI.vi" "PMT3"(w531) -> ()
            n444 = local write "PMT3"(w531) -> ()
            n445 = call "MCCPMTstore.vi"("MCCPMT in"=w535, "pmt voltage 1"=w532, "pmt voltage 2"=w533, "pmt voltage 3"=w531) -> ("MCCPMT out"=w536:refnum<class "MCCPMT.lvclass">)  [unwired: 10 in, 1 out]
          }
          frame True {
            n446 = property on="preset3" class="Bool"() -> ("BoolText.Text"=w541:string)  [unwired: 2 in, 2 out]
            n447 = local write "PMT3"(TRUE ("PMT2 on")) -> ()
            n448 = Fract/Exp String To Number(string=w541) -> (number=w540:dbl)  [unwired: 3 in, 1 out]
            n449 = local write "PMT3"(w540) -> ()
            n450 = call "MCCPMTupdate.vi"("MCCPMT in"=w544, "pmt voltage 1"=w539, "pmt voltage 2"=w538, "pmt voltage 3"=w540) -> ("MCCPMT out"=w543:refnum<class "MCCPMT.lvclass">, "error out"=w537:errorcluster)  [unwired: 10 in]
          }
        }
        n451 = property on="Pass UI values" class="Bool (strict)"(error in=w524) -> ("Value"=w526:bool)  [unwired: 1 in, 2 out]
        n452 = Not(x=w526) -> (.not. x?=w525:bool)
        n453 = property on="Pass UI values" class="Bool (strict)"("Val(Sgnl)"=w525) -> ()  [unwired: 2 in, 2 out]
      }
      event "Pump": Value Change {
        n454 = event-data() -> ()  [unwired: 1 in, 6 out]
        n455 = disable-structure shown="Disabled" {
          disable-tunnel: w545 -> [w551 _]
          frame Disabled {
            n456 = call "Command.vi"("Microscope events"=MicroscopeEvent."M.OpenPump" ("element"), "Microscope in"=w551) -> ()  [unwired: 8 in, 2 out]
          }
          frame Enabled {
          }
        }
        n457 = disable-structure shown="Enabled" {
          disable-tunnel: [w552 w553] -> w548
          frame Disabled {
            n458 = local read "Hardware Settings"() -> (w552:T5)
          }
          frame Enabled {
            n459 = global read "GlobalUI.vi" "Hardware Settings"() -> (w553:T5)
          }
        }
        n460 = call "MCCOpen.vi"("Open"="Pump", "Hardware Settings"=w548, "index"=0) -> ()  [unwired: 8 in, 1 out]
      }
      event Mouse Enter {
        n461 = event-data() -> ()  [unwired: 1 in, 4 out]
        n462 = property on="XY Graph 3" class="XYGraph (strict)"("Cursor Palette Vis"=TRUE ("Cursor Legend Visible")) -> ()  [unwired: 2 in, 2 out]
      }
      event Mouse Leave {
        n463 = event-data() -> ()  [unwired: 1 in, 4 out]
        n464 = property on="XY Graph 3" class="XYGraph (strict)"("Cursor Palette Vis"=FALSE ("Cursor Legend Visible")) -> ()  [unwired: 2 in, 2 out]
      }
      event "CH2": Mouse Leave {
        n465 = event-data() -> ()  [unwired: 1 in, 4 out]
        n466 = property on="CH2" class="IntGraph (strict)"("Cursor Palette Vis"=FALSE ("Cursor Legend Visible")) -> ()  [unwired: 2 in, 2 out]
      }
      event "CH1": Mouse Leave {
        n467 = event-data() -> ()  [unwired: 1 in, 4 out]
        n468 = property on="CH1" class="IntGraph (strict)"("Cursor Palette Vis"=FALSE ("Cursor Legend Visible")) -> ()  [unwired: 2 in, 2 out]
      }
      event "CH3": Mouse Enter {
        n469 = event-data() -> ()  [unwired: 1 in, 4 out]
        n470 = property on="CH3" class="IntGraph (strict)"("Cursor Palette Vis"=TRUE ("Cursor Legend Visible")) -> ()  [unwired: 2 in, 2 out]
      }
      event "CH2": Mouse Enter {
        n471 = event-data() -> ()  [unwired: 1 in, 4 out]
        n472 = property on="CH2" class="IntGraph (strict)"("Cursor Palette Vis"=TRUE ("Cursor Legend Visible")) -> ()  [unwired: 2 in, 2 out]
      }
      event "CH1": Mouse Enter {
        n473 = event-data() -> ()  [unwired: 1 in, 4 out]
        n474 = property on="CH1" class="IntGraph (strict)"("Cursor Palette Vis"=TRUE ("Cursor Legend Visible")) -> ()  [unwired: 2 in, 2 out]
      }
      event "CH3": Cursor Move {
        n475 = event-data() -> ("CursLoc"=w568:cluster{"X":dbl, "Y":dbl})  [unwired: 1 in, 8 out]
        n476 = property on="CH2" class="IntGraph (strict)"("Cursor.Cursor Position"=w568) -> ()  [unwired: 2 in, 2 out]
        n477 = property on="CH1" class="IntGraph (strict)"("Cursor.Cursor Position"=w568) -> ()  [unwired: 2 in, 2 out]
        n478 = Unbundle By Name(w568) -> ("X"=w572:dbl, "Y"=w571:dbl)
        n479 = property on="Scan Parameters" class="Clust (strict)"() -> ("Value"=w573:T4)  [unwired: 2 in, 2 out]
        n480 = call "Cursor_calc_voltage.vi"("Y"=w571, "X"=w572, "Scan Parameters"=w573) -> ("Y (Volts)"=w569:dbl, "X (Volts)"=w570:dbl)  [unwired: 7 in]
        n481 = global write "GlobalUI.vi" "Cursor X (V)"(w570) -> ()
        n482 = global write "GlobalUI.vi" "Cursor Y (V)"(w569) -> ()
      }
      event "CH2": Cursor Move {
        n483 = event-data() -> ("CursLoc"=w575:cluster{"X":dbl, "Y":dbl})  [unwired: 1 in, 8 out]
        n484 = property on="CH3" class="IntGraph (strict)"("Cursor.Cursor Position"=w575) -> ()  [unwired: 2 in, 2 out]
        n485 = property on="CH1" class="IntGraph (strict)"("Cursor.Cursor Position"=w575) -> ()  [unwired: 2 in, 2 out]
        n486 = Unbundle By Name(w575) -> ("X"=w579:dbl, "Y"=w578:dbl)
        n487 = property on="Scan Parameters" class="Clust (strict)"() -> ("Value"=w580:T4)  [unwired: 2 in, 2 out]
        n488 = call "Cursor_calc_voltage.vi"("Y"=w578, "X"=w579, "Scan Parameters"=w580) -> ("Y (Volts)"=w576:dbl, "X (Volts)"=w577:dbl)  [unwired: 7 in]
        n489 = global write "GlobalUI.vi" "Cursor X (V)"(w577) -> ()
        n490 = global write "GlobalUI.vi" "Cursor Y (V)"(w576) -> ()
      }
      event "CH1": Cursor Move {
        n491 = event-data() -> ("CursLoc"=w582:cluster{"X":dbl, "Y":dbl})  [unwired: 1 in, 8 out]
        n492 = property on="CH2" class="IntGraph (strict)"("Cursor.Cursor Position"=w582) -> ()  [unwired: 2 in, 2 out]
        n493 = property on="CH1" class="IntGraph (strict)"("Cursor.Cursor Position"=w582) -> ()  [unwired: 2 in, 2 out]
        n494 = Unbundle By Name(w582) -> ("X"=w586:dbl, "Y"=w585:dbl)
        n495 = property on="Scan Parameters" class="Clust (strict)"() -> ("Value"=w587:T4)  [unwired: 2 in, 2 out]
        n496 = call "Cursor_calc_voltage.vi"("Y"=w585, "X"=w586, "Scan Parameters"=w587) -> ("Y (Volts)"=w583:dbl, "X (Volts)"=w584:dbl)  [unwired: 7 in]
        n497 = global write "GlobalUI.vi" "Cursor X (V)"(w584) -> ()
        n498 = global write "GlobalUI.vi" "Cursor Y (V)"(w583) -> ()
      }
      event "CH3": Mouse Leave {
        n499 = event-data() -> ()  [unwired: 1 in, 4 out]
        n500 = property on="CH3" class="IntGraph (strict)"("Cursor Palette Vis"=FALSE ("Cursor Legend Visible")) -> ()  [unwired: 2 in, 2 out]
      }
      event Mouse Enter {
        n501 = event-data() -> ()  [unwired: 1 in, 4 out]
        n502 = property on="XY Graph 2" class="XYGraph (strict)"("Cursor Palette Vis"=TRUE ("Cursor Legend Visible")) -> ()  [unwired: 2 in, 2 out]
      }
      event Mouse Leave {
        n503 = event-data() -> ()  [unwired: 1 in, 4 out]
        n504 = property on="XY Graph 2" class="XYGraph (strict)"("Cursor Palette Vis"=FALSE ("Cursor Legend Visible")) -> ()  [unwired: 2 in, 2 out]
      }
      event Mouse Enter {
        n505 = event-data() -> ()  [unwired: 1 in, 4 out]
        n506 = property on="XY Graph" class="XYGraph (strict)"("Cursor Palette Vis"=TRUE ("Cursor Legend Visible")) -> ()  [unwired: 2 in, 2 out]
      }
      event Mouse Leave {
        n507 = event-data() -> ()  [unwired: 1 in, 4 out]
        n508 = property on="XY Graph" class="XYGraph (strict)"("Cursor Palette Vis"=FALSE ("Cursor Legend Visible")) -> ()  [unwired: 2 in, 2 out]
      }
      event "Stokes": Value Change {
        n509 = event-data() -> ()  [unwired: 1 in, 6 out]
        n510 = disable-structure shown="Disabled" {
          disable-tunnel: w599 -> [w605 _]
          frame Disabled {
            n511 = call "Command.vi"("Microscope events"=MicroscopeEvent."M.OpenStokes" ("element"), "Microscope in"=w605) -> ()  [unwired: 8 in, 2 out]
          }
          frame Enabled {
          }
        }
        n512 = disable-structure shown="Enabled" {
          disable-tunnel: [w606 w607] -> w602
          frame Disabled {
            n513 = local read "Hardware Settings"() -> (w606:T5)
          }
          frame Enabled {
            n514 = global read "GlobalUI.vi" "Hardware Settings"() -> (w607:T5)
          }
        }
        n515 = call "MCCOpen.vi"("Open"="Stokes", "Hardware Settings"=w602, "index"=1) -> ()  [unwired: 8 in, 1 out]
      }
      event "zero1": Value Change {
        n516 = event-data() -> ()  [unwired: 1 in, 6 out]
        n517 = local read "Acquire"() -> (w611:bool)
        n518 = case shown="False" w611 {
          tunnel: w613 -> [w618 w624]
          tunnel: [w617 w621] -> w612
          tunnel: [_ w619] -> w608
          frame True {
            w616 = 0.0 ("PMT1")
            n519 = local write "PMT1"(w616) -> ()
            n520 = local read "PMT2"() -> (w615:dbl)
            n521 = local read "PMT3"() -> (w614:dbl)
            n522 = call "MCCPMTupdate.vi"("MCCPMT in"=w618, "pmt voltage 1"=w616, "pmt voltage 2"=w615, "pmt voltage 3"=w614) -> ("MCCPMT out"=w617:refnum<class "MCCPMT.lvclass">)  [unwired: 10 in, 1 out]
          }
          frame False {
            w623 = 0.0 ("PMT1")
            n523 = local read "PMT3"() -> (w620:dbl)
            n524 = local write "PMT1"(w623) -> ()
            n525 = local read "PMT2"() -> (w622:dbl)
            n526 = call "MCCPMTstore.vi"("MCCPMT in"=w624, "pmt voltage 1"=w623, "pmt voltage 2"=w622, "pmt voltage 3"=w620) -> ("MCCPMT out"=w621:refnum<class "MCCPMT.lvclass">, "error out"=w619:errorcluster)  [unwired: 10 in]
          }
        }
        n527 = property on="Pass UI values" class="Bool (strict)"(error in=w608) -> ("Value"=w610:bool)  [unwired: 1 in, 2 out]
        n528 = Not(x=w610) -> (.not. x?=w609:bool)
        n529 = property on="Pass UI values" class="Bool (strict)"("Val(Sgnl)"=w609) -> ()  [unwired: 2 in, 2 out]
      }
      event "zero2": Value Change {
        n530 = event-data() -> ()  [unwired: 1 in, 6 out]
        n531 = local read "Acquire"() -> (w628:bool)
        n532 = case shown="False" w628 {
          tunnel: w630 -> [w636 w641]
          tunnel: [w633 w640] -> w629
          tunnel: [w631 _] -> w625
          frame False {
            w635 = 0.0 ("PMT1")
            n533 = local read "PMT3"() -> (w632:dbl)
            n534 = local read "PMT1"() -> (w634:dbl)
            n535 = local write "PMT2"(w635) -> ()
            n536 = call "MCCPMTstore.vi"("MCCPMT in"=w636, "pmt voltage 1"=w634, "pmt voltage 2"=w635, "pmt voltage 3"=w632) -> ("MCCPMT out"=w633:refnum<class "MCCPMT.lvclass">, "error out"=w631:errorcluster)  [unwired: 10 in]
          }
          frame True {
            w638 = 0.0 ("PMT1")
            n537 = local read "PMT1"() -> (w639:dbl)
            n538 = local write "PMT2"(w638) -> ()
            n539 = local read "PMT3"() -> (w637:dbl)
            n540 = call "MCCPMTupdate.vi"("MCCPMT in"=w641, "pmt voltage 1"=w639, "pmt voltage 2"=w638, "pmt voltage 3"=w637) -> ("MCCPMT out"=w640:refnum<class "MCCPMT.lvclass">)  [unwired: 10 in, 1 out]
          }
        }
        n541 = property on="Pass UI values" class="Bool (strict)"(error in=w625) -> ("Value"=w627:bool)  [unwired: 1 in, 2 out]
        n542 = Not(x=w627) -> (.not. x?=w626:bool)
        n543 = property on="Pass UI values" class="Bool (strict)"("Val(Sgnl)"=w626) -> ()  [unwired: 2 in, 2 out]
      }
      event "zero3": Value Change {
        n544 = event-data() -> ()  [unwired: 1 in, 6 out]
        n545 = local read "Acquire"() -> (w645:bool)
        n546 = case shown="True" w645 {
          tunnel: w647 -> [w652 w658]
          tunnel: [w650 w657] -> w646
          tunnel: [_ w653] -> w642
          frame False {
            w649 = 0.0 ("PMT1")
            n547 = local read "PMT2"() -> (w648:dbl)
            n548 = local write "PMT3"(w649) -> ()
            n549 = local read "PMT1"() -> (w651:dbl)
            n550 = call "MCCPMTstore.vi"("MCCPMT in"=w652, "pmt voltage 1"=w651, "pmt voltage 2"=w648, "pmt voltage 3"=w649) -> ("MCCPMT out"=w650:refnum<class "MCCPMT.lvclass">)  [unwired: 10 in, 1 out]
          }
          frame True {
            w654 = 0.0 ("PMT1")
            n551 = local read "PMT1"() -> (w656:dbl)
            n552 = local write "PMT3"(w654) -> ()
            n553 = local read "PMT2"() -> (w655:dbl)
            n554 = call "MCCPMTupdate.vi"("MCCPMT in"=w658, "pmt voltage 1"=w656, "pmt voltage 2"=w655, "pmt voltage 3"=w654) -> ("MCCPMT out"=w657:refnum<class "MCCPMT.lvclass">, "error out"=w653:errorcluster)  [unwired: 10 in]
          }
        }
        n555 = property on="Pass UI values" class="Bool (strict)"(error in=w642) -> ("Value"=w644:bool)  [unwired: 1 in, 2 out]
        n556 = Not(x=w644) -> (.not. x?=w643:bool)
        n557 = property on="Pass UI values" class="Bool (strict)"("Val(Sgnl)"=w643) -> ()  [unwired: 2 in, 2 out]
      }
      event "PMT2", "PMT1", "PMT3": Value Change {
        n558 = event-data() -> ()  [unwired: 1 in, 6 out]
        n559 = local read "PMT1"() -> (w664:dbl)
        n560 = local read "PMT3"() -> (w662:dbl)
        n561 = local read "PMT2"() -> (w663:dbl)
        n562 = local read "Acquire"() -> (w665:bool)
        n563 = case shown="True" w665 {
          tunnel: [w672 w677] -> w667
          tunnel: w666 -> [w671 w678]
          tunnel: w664 -> [w670 w676]
          tunnel: w663 -> [w669 w675]
          tunnel: w662 -> [w668 w674]
          tunnel: [_ w673] -> w659
          frame False {
            n564 = call "MCCPMTstore.vi"("MCCPMT in"=w671, "pmt voltage 1"=w670, "pmt voltage 2"=w669, "pmt voltage 3"=w668) -> ("MCCPMT out"=w672:refnum<class "MCCPMT.lvclass">)  [unwired: 10 in, 1 out]
          }
          frame True {
            n565 = call "MCCPMTupdate.vi"("MCCPMT in"=w678, "pmt voltage 1"=w676, "pmt voltage 2"=w675, "pmt voltage 3"=w674) -> ("MCCPMT out"=w677:refnum<class "MCCPMT.lvclass">, "error out"=w673:errorcluster)  [unwired: 10 in]
          }
        }
        n566 = property on="Pass UI values" class="Bool (strict)"(error in=w659) -> ("Value"=w661:bool)  [unwired: 1 in, 2 out]
        n567 = Not(x=w661) -> (.not. x?=w660:bool)
        n568 = property on="Pass UI values" class="Bool (strict)"("Val(Sgnl)"=w660) -> ()  [unwired: 2 in, 2 out]
      }
      event "show flyback data", "disable averaging", "Use Image Controls Min Max values for tiff": Value Change {
        n569 = event-data() -> ()  [unwired: 1 in, 6 out]
        n570 = global write "GlobalUI.vi" "show flyback data"("show flyback data") -> ()
        n571 = global write "GlobalUI.vi" "disable averaging"("disable averaging") -> ()
        n572 = global write "GlobalUI.vi" "Use Image Controls Min Max values for tiff"("Use Image Controls Min Max values for tiff") -> ()
      }
    }
    n573 = global write "GlobalUI.vi" "MCCPMT"(w56) -> ()
  }
  n574 = while {
    stop <- FALSE stop-if-true
    # "View \nUpdates the graphs"
    n575 = call "ImageData.vi"() -> ("Intensity vs Stage Position (mm)"=w692:cluster{dbl[], dbl[]}[], "Image intensities"=w699:dbl[], "Images"=w701:dbl[][][])  [unwired: 9 in]
    n576 = Index Array(array=w701) -> (element #1=→"CH1":dbl[][], element #2=→"CH2":dbl[][], element #3=→"CH3":dbl[][])  [unwired: 9 in]
    n577 = Index Array(array=w692) -> (element #1=→"XY Graph":cluster{dbl[], dbl[]}, element #2=→"XY Graph 2":cluster{dbl[], dbl[]}, element #3=→"XY Graph 3":cluster{dbl[], dbl[]})  [unwired: 3 in]
    n578 = Wait (ms)(milliseconds to wait=u32 10) -> ()  [unwired: 1 out]
    n579 = Index Array(array=w699) -> (element #1=→"intensity1":dbl, element #2=→"intensity2":dbl, element #3=→"intensity3":dbl)  [unwired: 3 in]
    n580 = global read "GlobalUI.vi" "MakeAcquireButtonFalse"() -> (w683:bool)
    n581 = global read "GlobalUI.vi" "PMT1 on"() -> (→"PMT1":bool)
    n582 = global read "GlobalUI.vi" "PMT2 on"() -> (→"PMT2":bool)
    n583 = global read "GlobalUI.vi" "PMT3 on"() -> (→"PMT3":bool)
    n584 = global read "GlobalUI.vi" "error out"() -> (→"error out":errorcluster)
    n585 = case shown="True" w683 {
      selector: w683 -> [_ w703]
      frame False {
      }
      frame True {
        n586 = Not(x=w703) -> (.not. x?=w702:bool)
        n587 = global write "GlobalUI.vi" "MakeAcquireButtonFalse"(w702) -> ()
        n588 = local write "Acquire"(w702) -> ()
      }
    }
  }
  n589 = while {
    stop <- FALSE stop-if-true
    # "Pass UI Values\nDedicated Event Structure\nto detect passing of UI variables"
    n590 = event shown="[0] \"Pass UI values\": Value Change" {
      selector: _ -> [_]
      dyn-events: _ -> [_]
      timeout: _ -> [_]
      event "Pass UI values": Value Change {
        n591 = event-data() -> ()  [unwired: 1 in, 5 out]
        n592 = stacked-sequence {
          frame #0 {
            # "Update Settings"
            n593 = global read "GlobalUI.vi" "must be an integer"() -> (→"must be an integer":dbl)
            n594 = global write "GlobalUI.vi" "Stage Acquire Parameters"("Stage Acquire Parameters") -> ()
            n595 = in-place {
              n596 = in-place-cluster #8("Scan Parameters") -> ()  [unwired: 1 out]
              n597 = local read "Zoom"() -> (w712:dbl)
              n598 = global write "GlobalUI.vi" "Zoom"(w712) -> ()
              n599 = in-place-cluster #8("Zoom"=w712) -> (w708:T4)
            }
            n600 = global write "GlobalUI.vi" "Hardware Settings"("Hardware Settings") -> ()
            n601 = global write "GlobalUI.vi" "Scan Parameters"(w708) -> ()
            n602 = local write "Scan Parameters"(w708) -> ()
            n603 = global write "GlobalUI.vi" "Reading thresholds"("Reading thresholds") -> ()
            n604 = global write "GlobalUI.vi" "Reading threshold defaults"("Reading thresholds defaults") -> ()
          }
          frame #1 {
            n605 = property on="CH3" class="IntGraph (strict)"() -> ("Cursor.Cursor X"=w717:dbl)  [unwired: 2 in, 2 out]
            n606 = property on="CH3" class="IntGraph (strict)"() -> ("Cursor.Cursor Y"=w714:dbl)  [unwired: 2 in, 2 out]
            n607 = property on="Scan Parameters" class="Clust (strict)"() -> ("Value"=w713:T4)  [unwired: 2 in, 2 out]
            n608 = call "Cursor_calc_voltage.vi"("Y"=w714, "X"=w717, "Scan Parameters"=w713) -> ("Y (Volts)"=w715:dbl, "X (Volts)"=w716:dbl)  [unwired: 7 in]
            n609 = global write "GlobalUI.vi" "Cursor Y (V)"(w715) -> ()
            n610 = global write "GlobalUI.vi" "Cursor X (V)"(w716) -> ()
            n611 = disable-structure shown="Enabled" {
              frame Disabled {
              }
              frame Enabled {
              }
            }
          }
          frame #2 {
            # "Update save information"
            n612 = global write "GlobalUI.vi" "Autosave"("Save This") -> ()
            n613 = global write "GlobalUI.vi" "Save Path"("Save Path") -> ()
            n614 = global write "GlobalUI.vi" "Pump Power (mW)"("Pump Power (mW)") -> ()
            n615 = global write "GlobalUI.vi" "Stokes Power (mW)"("Stokes Power (mW)") -> ()
            n616 = global write "GlobalUI.vi" "Sample Description"("Sample Description") -> ()
          }
          frame #3 {
            # "Intensity Chart updates"
            n617 = disable-structure shown="Enabled" {
              frame Disabled {
                n618 = property on="CH1" class="IntGraph (strict)"() -> ("ZScale.Minimum"=w728:dbl)  [unwired: 2 in, 2 out]
                n619 = property on="CH2" class="IntGraph (strict)"() -> ("ZScale.Minimum"=w729:dbl)  [unwired: 2 in, 2 out]
                n620 = property on="CH3" class="IntGraph (strict)"() -> ("ZScale.Minimum"=w730:dbl)  [unwired: 2 in, 2 out]
                n621 = Build Array(w728, w729, w730) -> (w727:dbl[])
                n622 = property on="CH1" class="IntGraph (strict)"() -> ("ZScale.Maximum"=w724:dbl)  [unwired: 2 in, 2 out]
                n623 = property on="CH2" class="IntGraph (strict)"() -> ("ZScale.Maximum"=w725:dbl)  [unwired: 2 in, 2 out]
                n624 = property on="CH3" class="IntGraph (strict)"() -> ("ZScale.Maximum"=w726:dbl)  [unwired: 2 in, 2 out]
                n625 = global write "GlobalUI.vi" "image  minimums"(w727) -> ()
                n626 = Build Array(w724, w725, w726) -> (w723:dbl[])
                n627 = global write "GlobalUI.vi" "image  maximums"(w723) -> ()
              }
              frame Enabled {
                n628 = property on="CH1" class="IntGraph (strict)"("ZScale.Minimum"="min1") -> ()  [unwired: 2 in, 2 out]
                n629 = property on="CH1" class="IntGraph (strict)"("ZScale.Maximum"="max1") -> ()  [unwired: 2 in, 2 out]
                n630 = property on="CH2" class="IntGraph (strict)"("ZScale.Minimum"="min2") -> ()  [unwired: 2 in, 2 out]
                n631 = property on="CH2" class="IntGraph (strict)"("ZScale.Maximum"="max2") -> ()  [unwired: 2 in, 2 out]
                n632 = property on="CH3" class="IntGraph (strict)"("ZScale.Minimum"="min3") -> ()  [unwired: 2 in, 2 out]
                n633 = property on="CH3" class="IntGraph (strict)"("ZScale.Maximum"="max3") -> ()  [unwired: 2 in, 2 out]
                n634 = Build Array("min1", "min2", "min3") -> (w732:dbl[])
                n635 = global write "GlobalUI.vi" "image  minimums"(w732) -> ()
                n636 = Build Array("max1", "max2", "max3") -> (w731:dbl[])
                n637 = global write "GlobalUI.vi" "image  maximums"(w731) -> ()
              }
            }
          }
          frame #4 {
            n638 = local read "PMT1"() -> (w741:dbl)
            n639 = local read "PMT3"() -> (w739:dbl)
            n640 = local read "PMT2"() -> (w740:dbl)
            n641 = global write "GlobalUI.vi" "PMT1"(w741) -> ()
            n642 = global write "GlobalUI.vi" "PMT2"(w740) -> ()
            n643 = global write "GlobalUI.vi" "PMT3"(w739) -> ()
          }
          frame #5 {
            n644 = local read "Preset PMT1"() -> (w744:dbl)
            n645 = local read "Preset PMT2"() -> (w743:dbl)
            n646 = local read "Preset PMT3"() -> (w742:dbl)
            n647 = global write "GlobalUI.vi" "PMT1"(w744) -> ()
            n648 = global write "GlobalUI.vi" "PMT2"(w743) -> ()
            n649 = global write "GlobalUI.vi" "PMT3"(w742) -> ()
            n650 = global write "GlobalUI.vi" "Target position mm"("Target position mm") -> ()
            n651 = global write "GlobalUI.vi" "Target position mm 2"("Target position mm 2") -> ()
            n652 = global write "GlobalUI.vi" "Target position mm 3"("Target position mm 3") -> ()
            n653 = global write "GlobalUI.vi" "Velocity mm/s"("Velocity mm/s") -> ()
          }
          frame #6 {
            n654 = local read "configuration file"() -> (w749:path)
            n655 = call "updateConfig.vi"("configuration file"=w749) -> ()  [unwired: 11 in]
          }
        }
      }
    }
  }
  n656 = disable-structure shown="Enabled" {
    frame Disabled {
      n657 = case shown="True" {
        selector: _ -> [_ _]
        tunnel: [_ w759] -> w757
        tunnel: [_ w758] -> w753
        frame False {
        }
        frame True {
          n658 = call "ImageFFTMasking.vi"() -> ("IFFTs"=w758:dbl[][][], "FFTs"=w759:dbl[][][])  [unwired: 10 in]
        }
      }
      n659 = Index Array(array=w757) -> (element #1=w756:dbl[][], element #2=w755:dbl[][], element #3=w754:dbl[][])  [unwired: 9 in]
      n660 = Index Array(array=w753) -> (element #1=w752:dbl[][], element #2=w751:dbl[][], element #3=w750:dbl[][])  [unwired: 9 in]
    }
    frame Enabled {
    }
  }
